vi "deleteMultichannel Lockin-Start Chopping.vi"() -> ()   [LabVIEW 2019, in "Instrument.Lockin.lvclass"]
uses:
  Instrument.Lockin/Instrument.Lockin.lvclass
  <vilib>/Utility/error.llb/DialogType.ctl
  Instrument UI.Lockin/Instrument UI.Lockin.lvclass
  <vilib>/measure/NI_MAPro.lvlib
  Instrument.DAQ/Instrument.DAQ.lvclass
  <vilib>/Utility/config.llb/NI_LVConfig.lvlib
  <vilib>/JKI/JKI SMO/SMO/SMO.lvclass
  <userlib>/LevyLab/Instrument Framework/SMOs/RemoteControl/RemoteControl.lvclass
  <userlib>/LevyLab/Instrument Framework/SMOs/RemoteControl/Typedefs/Message--Cluster.ctl
  <userlib>/LevyLab/Instrument Framework/SMOs/RemoteControl/Typedefs/PrivateEvents--RemoteControl.Configure.ctl
  Instrument.DAQ/Typedefs/Results--Cluster.ctl
  Instrument.DAQ/Typedefs/Set State-enum.ctl
  <vilib>/JKI/JKI SMO/SMO/Typedefs/Reserve State--Enum.ctl
  <vilib>/JKI/JKI SMO/SMO/Typedefs/Public Events.ctl
  <vilib>/JKI/JKI SMO/SMO/Typedefs/SMOState --Enum.ctl
  Instrument.DAQ/Typedefs/DAQ.Sampling.Sample Mode--Ring.ctl
  Instrument.DAQ/Typedefs/Sweep.Configuration--Cluster.ctl
  Instrument.DAQ/Typedefs/PublicEvents--DAQ.getSweepWaveforms.ctl
  Instrument.DAQ/Typedefs/PrivateEvents--DAQ.setCalibration.ctl
  Instrument.Lockin/Typedefs/Offset Mode--Enum.ctl
  Instrument.DAQ/Typedefs/Sweep.Pattern--Enum.ctl
  Instrument.DAQ/Typedefs/Sweep.Channel--Cluster.ctl
  Instrument.DAQ/Typedefs/DAQ.Sampling.Sampling--Cluster.ctl
  Instrument UI.Lockin/private/Set Legend (WFChart).vi
  Instrument UI.Lockin/private/Set Legend (WFGraph).vi
  Instrument UI.Lockin/private/Set Legend (WDTWFGraph).vi
  Instrument UI.Lockin/private/Set All Plot Visibility (WFGraph).vi
  Instrument UI.Lockin/private/Set All Plot Visibility (WFChart).vi
  <vilib>/Platform/browser.llb/Open URL in Default Browser (string).vi
  <userlib>/LevyLab/Instrument Framework/SMOs/Instrument/Instrument.lvclass
  Instrument UI.Lockin/private/Set Plot Visibility (WFGraph).vi
  Instrument UI.Lockin/private/Set Plot Visibility (WFChart).vi
  <userlib>/LevyLab/Instrument Framework/SMOs/Logger.Error/Logger.Error.lvclass
  f8e81ae1-39f2-419c-8ba3-60eeaa59b30a.vi
  Instrument UI.Lockin/private/Set All Plot Visibility (XYGraph).vi
  Instrument UI.Lockin/private/Set Plot Visibility (XYGraph).vi
  <userlib>/_OpenG.lib/error/error.llb/Filter Error Codes (Array)__ogtk.vi
  <vilib>/Waveform/WDTOps.llb/WDT Waveform Duration DBL.vi
  Instrument.DAQ/Typedefs/Sweep.Channel--Cluster--Array.ctl
  C:/Program Files (x86)/National Instruments/LabVIEW 2019/vi.lib/JKI/JKI SMO/SMO/SMO.lvclass
  C:/Program Files (x86)/National Instruments/LabVIEW 2019/user.lib/LevyLab/Instrument Framework/SMOs/Instrument/Instrument.lvclass
  <vilib>/measure/maspectr.llb/FFT Power Spectrum and PSD for N Chan.vi
  Instrument.DAQ/Typedefs/DAQ.Config.AI.Coupling--enum.ctl
  Instrument.DAQ/Typedefs/DAQ.Config.AI.Range--enum.ctl
  Instrument.DAQ/Typedefs/DAQ.Config.AO.Range--enum.ctl
  Instrument.DAQ/Typedefs/AO.Channel.Function--Enum.ctl
  Instrument.DAQ/Typedefs/DAQ.Calibration--Cluster.ctl
  Instrument.DAQ/Typedefs/DAQ.Type--enum.ctl
  Instrument UI.Lockin/Typedefs/Display-Enum.ctl
  Instrument.DAQ/Typedefs/Simulation Mode--enum.ctl
  Instrument.Lockin/Typedefs/DELETE_Lockin.Auto Sample Mode--Enum.ctl
  Instrument.DAQ/Typedefs/DAQ.Configuration--Cluster.ctl
  Instrument.DAQ/Typedefs/REF.Channel--Cluster.ctl
  Instrument.Lockin/Typedefs/Results Type--Enum.ctl
panel:
  out "Results Plot Names":string[](array[string])
  in  "Tab Control 4":T1(tab)
  in  "Disable all AI Ref":bool
  in  "Enable only AI Ref1":bool
  in  "Reset Phase":bool
  in  "AI Channels":T2(array[cluster]) {"References" items=["", "1"]}
  in  "AO freq link":dbl=13.0 format="%.3p"
  in  "AO Amp Limit":dbl=0.009999999 format="%.3p"
  in  "Limit Amplitudes":bool
  in  "Link Frequencies":bool
  in  "LP f (Hz)":dbl=100.0 format="%.3p"
  in  "Line":bool
  in  "Lowpass":bool
  in  "AO Channels":T4(array[cluster]) {"Phase" format="%.3g"; "Frequency" min=0.0001 max=10000.0 format="%.3g"; "Offset" format="%.3p"; "Amplitude" min=0.0 max=10.0 format="%.3p"}
  in  "REF Channels":T5[](array[typedef]) {"Roll-Off" min=1; "TC" min=0.0001 format="%#_3p"; "Phase" format="%.3g"; "Frequency" min=0.0001 max=10000.0 format="%.3g"; "Channel" min=1}
  in  "DAQ Config":T6[](array[typedef]) {"AI.Coupling" items=["AC"=10045, "DC"=10050, "GND"=10066]}
  in  "auto DAQ":bool
  in  "Max Fs Refresh Rate (Hz)":dbl=10.0 format="%#_13g"
  in  "Sampling Mode":T10
  in  "Sampling":T11={"Fs"=10000.0, "#s"=1000}
  in  "DAQ Type":T12=enum."PXI 446x"
  in  "Auto x*F1":dbl=5000.0 format="%#_13g"
  in  "Load Configuration":bool
  in  "Save Configuration":bool
  in  "AI Simulation mode":T13=enum."AI = noise*AO"
  in  "decimating factor":i32=1
  in  "Remove":bool
  in  "Measure":bool
  in  "Channels: Sweep":T15(array[cluster]) {"Channel" items=["AO1"=1, "AO2"=2, "AO3"=3, "AO4"=4, "AO5"=5, "AO6"=6, "AO7"=7, "AO8"=8]; "Start" format="%#_6p"; "End" format="%#_6p"}
  in  "Stop Sweep":bool caption="Stop"
  in  "Sweep Time (s)":dbl=20.0 format="%#_1f"
  in  "Start Sweep":bool caption="Start"
  in  "Initial Wait (s)":dbl=1.0
  out "Sweep Timer (s)":dbl caption="Timer (s)"
  in  "Return to Start?":bool
  out "Sampling Status":string="Good"
  in  "Output Gain":cluster{"AI.Ch":string, "Gain":dbl}[](array[cluster])=[{"AI.Ch"="AO1", "Gain"=1.0}, {"AI.Ch"="AO2", "Gain"=1.0}, {"AI.Ch"="AO3", "Gain"=1.0}, {"AI.Ch"="AO4", "Gain"=1.0}, {"AI.Ch"="AO5", "Gain"=1.0}, {"AI.Ch"="AO6", "Gain"=1.0}, {"AI.Ch"="AO7", "Gain"=1.0}, {"AI.Ch"="AO8", "Gain"=1.0}, {"AI.Ch"="AO9", "Gain"=1.0}, {"AI.Ch"="AO10", "Gain"=1.0}, {"AI.Ch"="AO11", "Gain"=1.0}, {"AI.Ch"="AO12", "Gain"=1.0}, {"AI.Ch"="AO13", "Gain"=1.0}, {"AI.Ch"="AO14", "Gain"=1.0}, {"AI.Ch"="AO15", "Gain"=1.0}, {"AI.Ch"="AO16", "Gain"=1.0}]
  in  "Input Gain":cluster{"AI.Ch":string, "Gain":dbl}[](array[cluster])=[{"AI.Ch"="AI1", "Gain"=1.0}, {"AI.Ch"="AI2", "Gain"=1.0}, {"AI.Ch"="AI3", "Gain"=1.0}, {"AI.Ch"="AI4", "Gain"=1.0}, {"AI.Ch"="AI5", "Gain"=1.0}, {"AI.Ch"="AI6", "Gain"=1.0}, {"AI.Ch"="AI7", "Gain"=1.0}, {"AI.Ch"="AI8", "Gain"=1.0}, {"AI.Ch"="AI9", "Gain"=1.0}, {"AI.Ch"="AI10", "Gain"=1.0}, {"AI.Ch"="AI11", "Gain"=1.0}, {"AI.Ch"="AI12", "Gain"=1.0}, {"AI.Ch"="AI13", "Gain"=1.0}, {"AI.Ch"="AI14", "Gain"=1.0}, {"AI.Ch"="AI15", "Gain"=1.0}, {"AI.Ch"="AI16", "Gain"=1.0}]
  out "State History":string=" Exit\r Data: Cleanup\r Events: Unregister\r UI: Cleanup\r UI: Disable Buttons\r Configuration: Write\r Error Logger: Destroy\r Lockin SMO: Stop\r Remote SMO: Stop\r Macro: Exit\r UI: Update Sweep Timer\r UI: Update Lockin Graphs\r UI: Update Waveform Graphs\r 4461: OUT\r UI: Update Sweep Timer\r UI: Update Lockin Graphs\r UI: Update Waveform Graphs\r 4461: OUT\r UI: Update Sweep Timer\r UI: Update Lockin Graphs\r UI: Update Waveform Graphs\r 4461: OUT"
  out "Refresh time (ms)":u32=103
  out "LockinDAQ SMO State":T16=enum."Stopped" caption="SMO State"
  out "RC SMO State":T16=enum."Stopped" caption="SMO State"
  in  "Update":bool
  in  "Enable Output":bool caption="Enable"
  in  "Output Channel":i32=1 min=1
  out "Output (V)":dbl
  in  "Aux Channel":tag="Dev2/ao0"
  in  "Voltage Output (V)":dbl min=-50.0 max=50.0
  in  "Amplifier Gain":dbl=1.0 min=-15.0 max=15.0
  out "DAQ Output (V)":dbl=-0.0 min=-3.5 max=3.5
  out "Amplified Output (V)":dbl=-0.0 min=-3.5 max=3.5
  in  "AI Channel":i32=1
  in  "Reference Channel":i32=1
  in  "Type":T17
  in  "Allowed remote system":string
  in  "Get Calibration":bool
  out "Cal Info":T18[](array[typedef]) {"SelfCal.LastDate/Time" format="%<%I:%M %p\n%m/%d/%Y>T"}
  in  "Self Calibrate":bool
  in  "Tab Control 3":enum32{"Page 1"}(tab)
  out "X":dbl=0.0014996100939563214 caption="X (V)" format="%#_3p"
  out "Y":dbl=-29.79492153733761 caption="Y (V)" format="%#_3p"
  in  "Channel":i32(ring)=1
  out "R":dbl=0.0014996100939563214 caption="R (V)" format="%#_3p"
  out "Theta":dbl=-29.79492153733761 caption="Theta (°)" format="%#_3p"
  in  "Display":T19=enum."R and Theta" caption="Enum"
  in  "Close":bool
  out "Status":string="Shutdown"
  in  "Pause":bool
  in  "Reset":bool
  in  "Start":bool
  in  "Help":bool
  in  "Trigger":bool
  in  "Tab Control 2":T20(tab)
  in  "AI Graph All":bool
  in  "AI Graph None":bool
  in  "Y Axis (Output)":enum16{"Analog Output", "Reference"}(ring) caption="Enum 3"
  in  "Y Axis (Input)":enum16{"Device", "ADC"}(ring) caption="Enum 3"
  in  "Decimate":enum16{"1", "10", "100", "1000"}(ring) caption="Enum 3"
  in  "X Axis":enum16{"Time", "Samples"}(ring) caption="Enum 3"
  out "AI Graph":waveform(dbl)[](graph)
  out "AO Graph":waveform(dbl)[](graph)
  in  "AO Graph All":bool
  in  "AO Graph None":bool
  in  "Y/Theta Range":dbl caption="Axis Range" format="%#_6p"
  in  "X/R Range":dbl caption="Axis Range" format="%#_6p"
  out "Lockin 2":waveform(dbl)[](graph) caption="Lockin Display 2"
  out "Lockin 1":waveform(dbl)[](graph)
  in  "Lockin 1 None":bool
  in  "Lockin 1 All":bool
  out "Results":string[][](table)
  out "XY Graph":cluster{"Wavenumber":dbl[], "Data":dbl[]}[](graph)
  in  "Numeric":dbl caption="Axis Range" format="%#_6p"
  out "Sweep Results Y":waveform(dbl)[](graph)
  out "Sweep Results X":waveform(dbl)[](graph)
  out "Sweep Results AI":waveform(dbl)[](graph)
  out "Sweep Results AO":waveform(dbl)[](graph)
  in  "# averages":u32=10 min=1
  in  "weighting mode":enum16{"Linear", "Exponential"}(ring)=enum."Exponential"
  in  "averaging mode":T21(ring)=enum."RMS averaging"
  in  "window":u16(ring) items=["Rectangle", "Hanning"]
  in  "export mode":u16(ring)=1 items=["Power Spectrum", "Power Spectral Density"]
  in  "restart":bool
  out "done?":bool=TRUE
  out "PS Chart":dbl[][](graph)
  out "PS WFGraph":cluster{"f0":dbl, "df":dbl, "magnitude":dbl[]}[](graph)
  out "averages":dbl=180.0
  # "Output"
  # "Input"
  # ">> DEVICE >>"
  # "Amp (V)"
  # "(*)"
  # "Ch"
  # "DC (V)"
  # "f (Hz)"
  # "Phase (°)"
  # "Function"
  # "Sweep"
  # "(*)"
  # "Ch"
  # "Ref1   2     3    4"
  # "Input: Pre-Filter"
  # "Output Settings"
  # "Reference"
  # "Reference Settings"
  # "Ch"
  # "f (Hz)"
  # "Phase (°)"
  # "TC (s)"
  # "Order"
  # "DAQ Channels"
  # "AI"
  # "Device"
  # "AO"
  # "Input: Offset"
  # "Ch"
  # "Range"
  # "Ch"
  # "Range"
  # "Coupling"
  # "Other Configuration"
  # "Sampling"
  # "Changing settings in this box will automatically\nreset the lockin and restart acquisition"
  # "Sweep"
  # "Channel"
  # "Start"
  # "End"
  # "Pattern"
  # "Status"
  # "Channel"
  # "Channel"
  # "Input Gain"
  # "Output Gain"
  # "Auxiliary Output"
  # "Configuration"
  # "- Use to control an auxiliiary card such as a multifunction DAQ (6115, 6120, etc)"
  # "Forward Lockin Input --> Lockin Output"
  # "- Choose an input lockin channel and value (X,Y, etc) and it will be written as a DC value to an output channel of your choosing.\n- Output is scaled by the input amplifier gain."
  # "Calibration"
  # "Self Cal\nLast Time"
  # "Self Cal\nLast Temp"
  # "Temp\nNow"
  # "Cal\nDue"
  # "Device"
  # "AI Graph"
  # "AO/Reference Graph"
  # "Lockin Results 1"
  # "Lockin Results 2"
  # "Lockin Results 2"
  # "Sweep Results"
  # "Sweep AO/AI"
  # "Power Spectra"
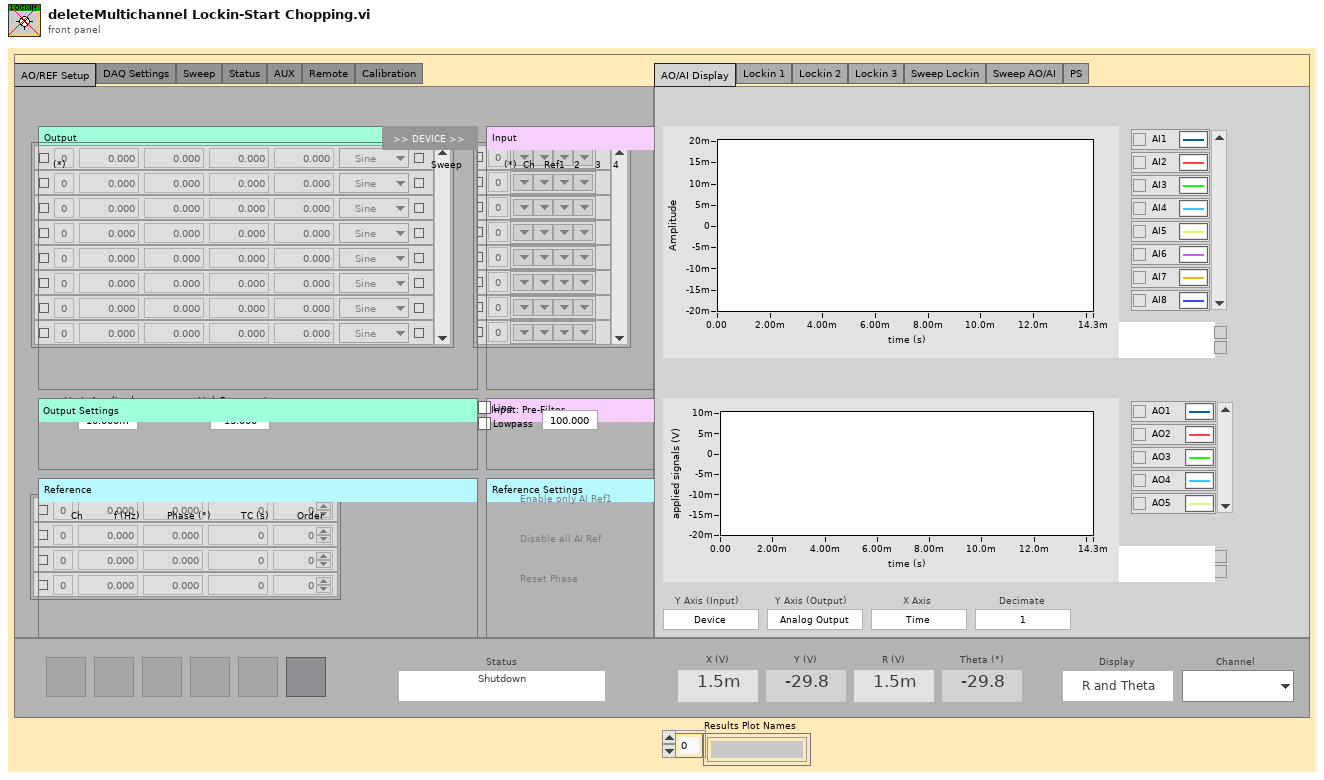
[diagram p1: front panel]
types:
  T1 = enum32{"AO/REF Setup", "DAQ Settings", "Sweep", "Status", "AUX", "Remote", "Calibration"}
  T2 = cluster{"Enable?":bool, "Channel":i32, "References":u16[]}[]
  T3 = typedef "Instrument.DAQ.lvclass/AO.Channel.Function--Enum.ctl" = enum16{"Sine", "Triangle", "Square"}
  T4 = cluster{"Enable?":bool, "Channel":i32, "Amplitude":dbl, "Offset":dbl, "Frequency":dbl, "Phase":dbl, "Function":T3, "Sweeping?":bool}[]
  T5 = typedef "Instrument.DAQ.lvclass/REF.Channel--Cluster.ctl" = cluster{"Enable?":bool, "Channel":i32, "Frequency":dbl, "Phase":dbl, "TC":dbl, "Roll-Off":i32}
  T6 = typedef "Instrument.DAQ.lvclass/DAQ.Configuration--Cluster.ctl" = cluster{"Device":string, "AO.Ch":string, "AO.Range":T7, "AI.Ch":string, "AI.Range":T8, "AI.Coupling":T9}
  T7 = typedef "Instrument.DAQ.lvclass/DAQ.Config.AO.Range--enum.ctl" = enum16{"±0.1", "±1.0", "±10.0"}
  T8 = typedef "Instrument.DAQ.lvclass/DAQ.Config.AI.Range--enum.ctl" = enum16{"±0.316", "±1.00", "±3.16", "±10.0", "±31.6", "±42.4"}
  T9 = typedef "Instrument.DAQ.lvclass/DAQ.Config.AI.Coupling--enum.ctl" = u16
  T10 = typedef "DELETE_Lockin.Auto Sample Mode--Enum.ctl" = enum16{"Manual", "Auto Fs", "Max Fs"}
  T11 = typedef "Instrument.DAQ.lvclass/DAQ.Sampling.Sampling--Cluster.ctl" = cluster{"Fs":dbl, "#s":i32}
  T12 = typedef "Instrument.DAQ.lvclass/DAQ.Type--enum.ctl" = enum16{"None", "USB 4431", "PXI 446x"}
  T13 = typedef "Instrument.DAQ.lvclass/Simulation Mode--enum.ctl" = enum16{"AI = HW simulated", "AI = noise*AO", "AI = waveguide"}
  T14 = typedef "Instrument.DAQ.lvclass/Sweep.Pattern--Enum.ctl" = enum16{"Ramp /", "Ramp /\\", "Smooth Ramp _/", "Smooth Ramp _/\\_", "Frequency"}
  T15 = cluster{"Enable?":bool, "Channel":u16, "Start":dbl, "End":dbl, "Pattern":T14}[]
  T16 = typedef "SMO.lvclass/SMOState --Enum.ctl" = enum16{"unknown", "Created", "Started", "Stopped"}
  T17 = typedef "Instrument.Lockin.lvclass/Results Type--Enum.ctl" = enum16{"X", "Y", "R", "Theta", "Mean"}
  T18 = typedef "Instrument.DAQ.lvclass/DAQ.Calibration--Cluster.ctl" = cluster{"Active Device":string, "SelfCal.LastDate/Time":dbl, "SelfCal.LastTemp":dbl, "DevTemp":dbl, "calibration due?":bool}
  T19 = typedef "Instrument UI.Lockin.lvclass/Display-Enum.ctl" = enum16{"X and Y", "R and Theta", "Mean"}
  T20 = enum32{"AO/AI Display", "Lockin 1", "Lockin 2", "Lockin 3", "Sweep Lockin", "Sweep AO/AI", "PS"}
  T21 = enum16{"No averaging", "Vector averaging", "RMS averaging", "Peak hold"}
  T22 = typedef "Instrument.DAQ.lvclass/Set State-enum.ctl" = enum16{"start", "stop", "reset", "start sweep", "stop sweep"}
  T23 = typedef "Instrument.DAQ.lvclass/Sweep.Configuration--Cluster.ctl" = cluster{"Sweep Time (s)":dbl, "Initial Wait (s)":dbl, "Return to Start":bool, "Channels":T24}
  T24 = typedef "Instrument.DAQ.lvclass/Sweep.Channel--Cluster--Array.ctl" = T25[]
  T25 = typedef "Instrument.DAQ.lvclass/Sweep.Channel--Cluster.ctl" = cluster{"Enable?":bool, "Channel":u16, "Start":dbl, "End":dbl, "Pattern":T14}
  T26 = enum32{"invalid app kind", "Development System", "Run Time System", "Student Edition", "Embedded LabVIEW", "Evaluation", "Custom"}
  T27 = enum8{"Enabled", "Disabled", "Disabled and Grayed Out"}
  T28 = enum32{"Invalid", "Standard", "Closed", "Hidden", "Minimized", "Maximized"}
  T29 = typedef "Instrument.DAQ.lvclass/PrivateEvents--DAQ.setCalibration.ctl" = enum16{"Check", "Calibrate"}
  T30 = cluster{"averaging mode":enum16{"No averaging", "Vector averaging", "RMS averaging", "Peak hold"}, "weighting mode":enum16{"Linear", "Exponential"}, "number of averages":u32}
  T31 = typedef "Instrument.Lockin.lvclass/Offset Mode--Enum.ctl" = enum16{"Measure", "Remove"}
  T32 = typedef "Instrument.DAQ.lvclass/Get State-enum.ctl" = enum16{"idle", "created", "started", "stopped", "sweeping"}
  T33 = typedef "RemoteControl.lvclass/PrivateEvents--RemoteControl.Configure.ctl" = cluster{"address":string, "Port":u16, "AllowedRemote":string, "Commands":string[], "timeout":i32}
  T34 = typedef "RemoteControl.lvclass/Message--Cluster.ctl" = cluster{"Command":string, "Data":variant, "ID":string}
  T35 = typedef "Instrument.DAQ.lvclass/PublicEvents--DAQ.getSweepWaveforms.ctl" = cluster{"Sweep AO":waveform(dbl)[], "Sweep AI":waveform(dbl)[], "Sweep Results X":waveform(dbl)[], "Sweep Results Y":waveform(dbl)[]}
  T36 = cluster{"Core":cluster{"Current VI Reference":refnum<vi>, "Close Panel on Exit?":bool}, "to":i32, "Lockin":refnum<class "Instrument.Lockin.lvclass">, "RemoteControl":refnum<class "RemoteControl.lvclass">, "Lockin.DAQ":refnum<class "Instrument.DAQ.lvclass">, "Logger.Error":refnum<class "Logger.Error.lvclass">, "RemoteControl.Configure":T33, "Message":T34, "HandledMessage":T34, "SweepWaveforms":T35}
  T37 = typedef "Instrument.DAQ.lvclass/State-enum.ctl" = enum16{"idle", "created", "started", "stopped", "sweeping"}
  T38 = typedef "Instrument.DAQ.lvclass/REF.Channel--Cluster--Array.ctl" = T5[]
  T39 = typedef "Instrument.DAQ.lvclass/DAQ Configuration--Cluster--Array.ctl" = T40[]
  T40 = typedef "Instrument.DAQ.lvclass/DAQ Configuration--Cluster.ctl" = cluster{"Device":string, "AO.Ch":string, "AO.Range":T41, "AI.Ch":string, "AI.Range":T42, "AI.Coupling":T43}
  T41 = typedef "Instrument.DAQ.lvclass/446xAO-enum.ctl" = enum16{"±0.1", "±1.0", "±10.0"}
  T42 = typedef "Instrument.DAQ.lvclass/446xAI-enum.ctl" = enum16{"±0.316", "±1.00", "±3.16", "±10.0", "±31.6", "±42.4"}
  T43 = typedef "Instrument.DAQ.lvclass/AI.coupling-enum.ctl" = u16
  T44 = typedef "Instrument.DAQ.lvclass/DAQ.Config.AO--Cluster--Array.ctl" = T45[]
  T45 = typedef "Instrument.DAQ.lvclass/DAQ.Config.AO--Cluster.ctl" = cluster{"Channels":tag, "Range":T7, "output terminal configuration":i32, "Type":T12}
  T46 = typedef "Instrument.DAQ.lvclass/DAQ.Config.AI--Cluster--Array.ctl" = T47[]
  T47 = typedef "Instrument.DAQ.lvclass/DAQ.Config.AI--Cluster.ctl" = cluster{"Channels":tag, "Coupling":T9, "Range":T8, "input terminal configuration":i32, "Type":T12}
  T48 = typedef "Instrument.DAQ.lvclass/Channel.Gain--Cluster--Array.ctl" = T49[]
  T49 = typedef "Instrument.DAQ.lvclass/Channel.Gain--Cluster.ctl" = cluster{"Channel":string, "Gain":dbl}
  T50 = typedef "Instrument.DAQ.lvclass/DAQ.Sampling.Sample Mode--Ring.ctl" = i32
  T51 = typedef "DialogType.ctl" = u16
  T52 = typedef "Instrument.DAQ.lvclass/Results--Cluster.ctl" = cluster{"Time Stamp":timestamp, "Results (Dictionary)":cluster{"key":string, "value":dbl}[]}
  T53 = cluster{"Current VI Reference":refnum<vi>, "Close Panel on Exit?":bool}
  T54 = typedef "SMO.lvclass/Public Events.ctl" = cluster{"Error":refnum<user-event>, "State":refnum<user-event>, "Reserve State":refnum<user-event>}
  T55 = typedef "RemoteControl.lvclass/PublicEvents--Cluster.ctl" = cluster{"SendMessageFromProcess":refnum<user-event>}
  T56 = typedef "Instrument.DAQ.lvclass/PublicEvents--Cluster.ctl" = cluster{"getAIChannels":refnum<user-event>, "getAOChannels":refnum<user-event>, "getREFChannels":refnum<user-event>, "getWaveforms":refnum<user-event>, "getResults":refnum<user-event>, "getSweepWaveforms":refnum<user-event>, "getCalibration":refnum<user-event>, "getDAQState":refnum<user-event>, "getDAQconfig":refnum<user-event>, "getInputGain":refnum<user-event>, "getOutputGain":refnum<user-event>, "getInputOffset":refnum<user-event>}
  T57 = typedef "Instrument.DAQ.lvclass/AI.Channel--Cluster--Array.ctl" = T58[]
  T58 = typedef "Instrument.DAQ.lvclass/AI.Channel--Cluster.ctl" = cluster{"Enable?":bool, "Channel":i32, "References":i32[]}
  T59 = typedef "Instrument.DAQ.lvclass/DAQ.Sampling--Cluster.ctl" = cluster{"Sampling":T11, "Sample Mode":T50, "Fs Mode":T60, "Fs Multiplier":dbl, "Refresh Rate (Hz)":dbl, "Decimation":i32}
  T60 = typedef "Instrument.DAQ.lvclass/DAQ.Sampling.Fs Mode--enum.ctl" = enum16{"Manual", "Auto Fs", "Max Fs"}
  T61 = typedef "Instrument.DAQ.lvclass/AO.Channel--Cluster--Array.ctl" = T62[]
  T62 = typedef "Instrument.DAQ.lvclass/AO.Channel--Cluster.ctl" = cluster{"Enable?":bool, "Channel":i32, "Amplitude":dbl, "Offset":dbl, "Frequency":dbl, "Phase":dbl, "Function":T3, "Sweeping?":bool}
  T63 = typedef "Instrument.DAQ.lvclass/Configuration.Prefilter--Cluster.ctl" = cluster{"60 Hz":bool, "Low Pass":bool, "Low Pass Cutoff (Hz)":dbl}
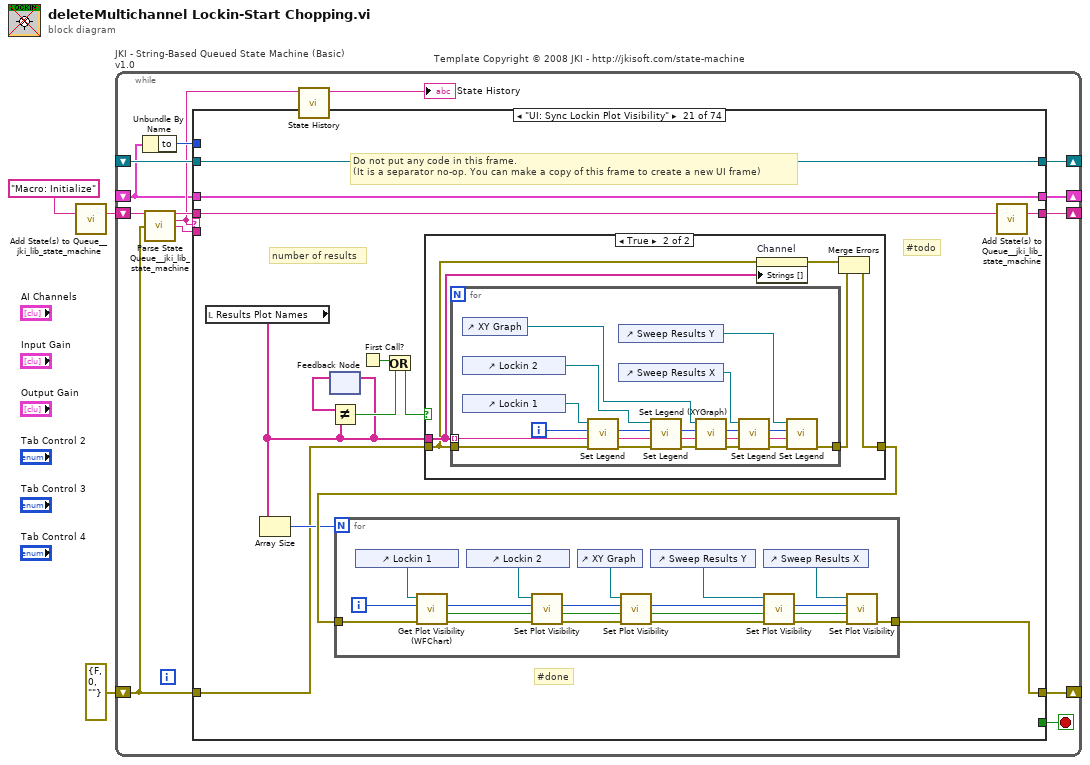
[diagram p0: block diagram]
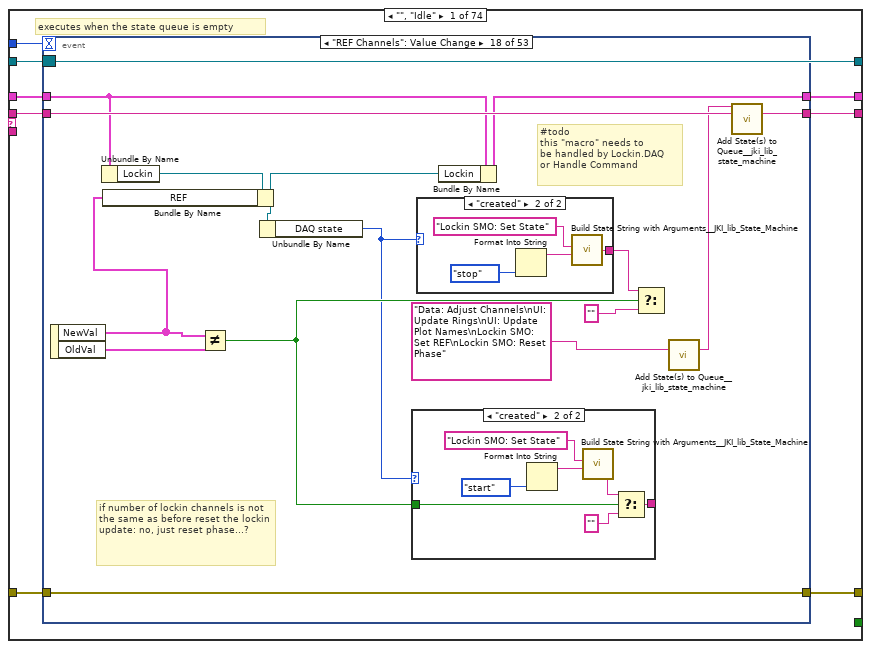
[diagram p2: hidden frame]
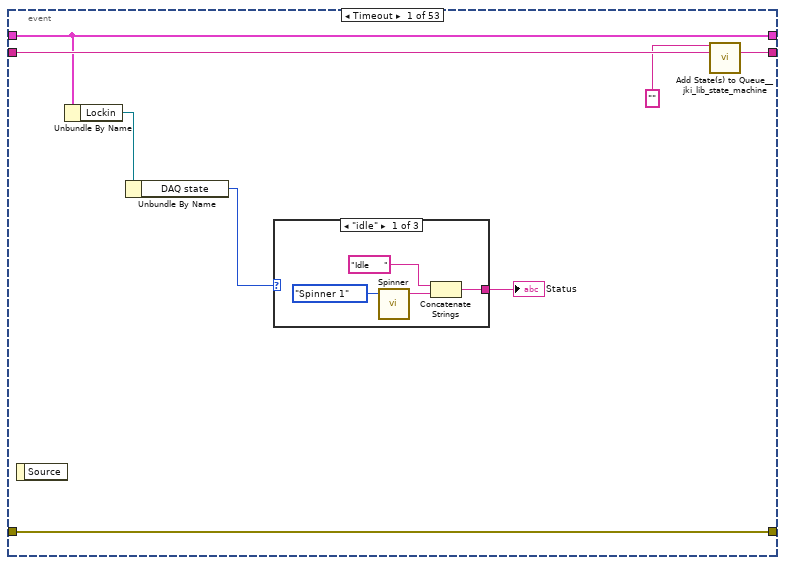
[diagram p3: hidden frame]
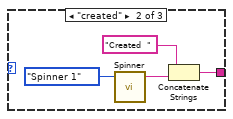
[diagram p4: hidden frame]
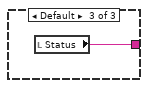
[diagram p5: hidden frame]
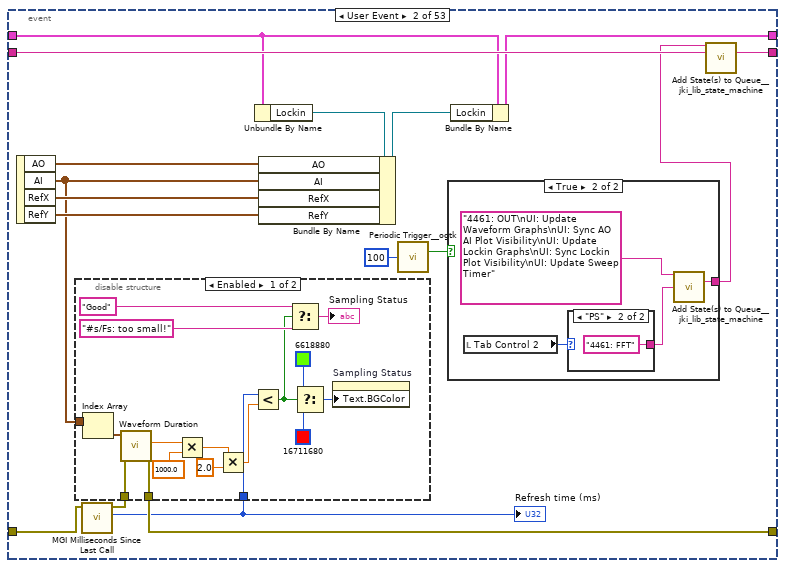
[diagram p6: hidden frame]
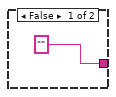
[diagram p7: hidden frame]
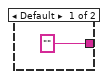
[diagram p8: hidden frame]
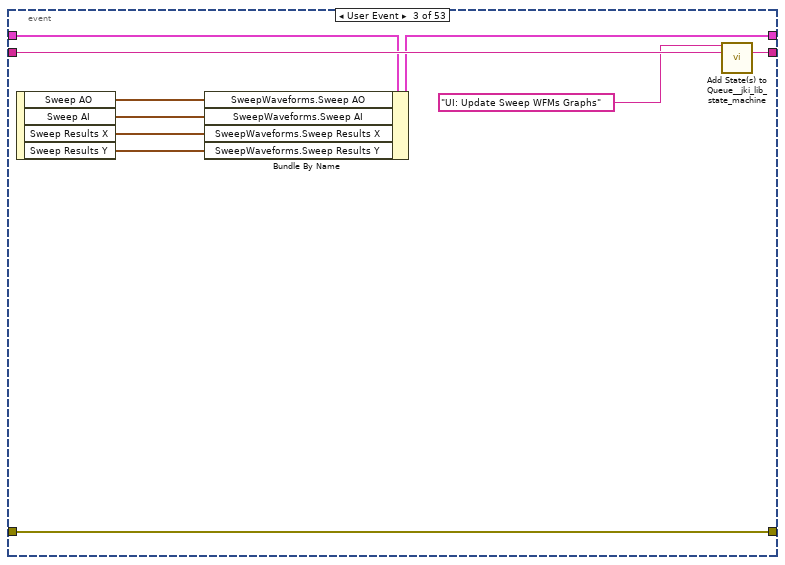
[diagram p10: hidden frame]
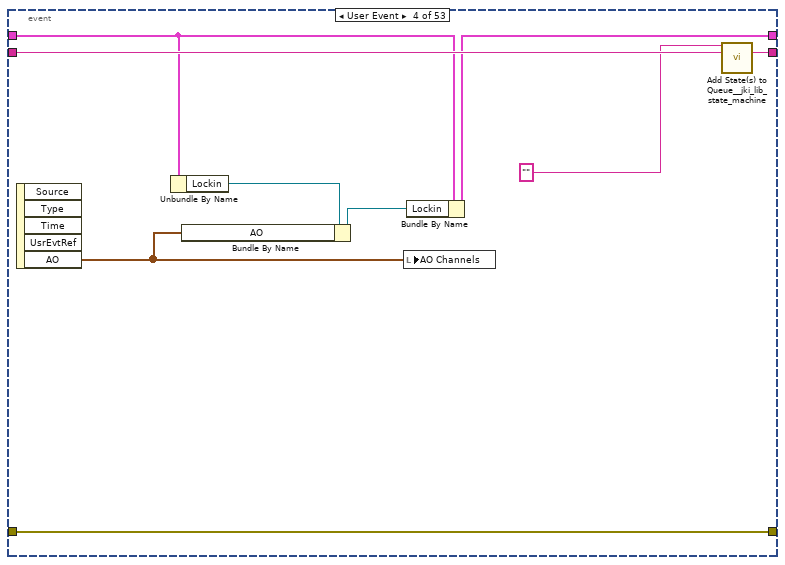
[diagram p11: hidden frame]
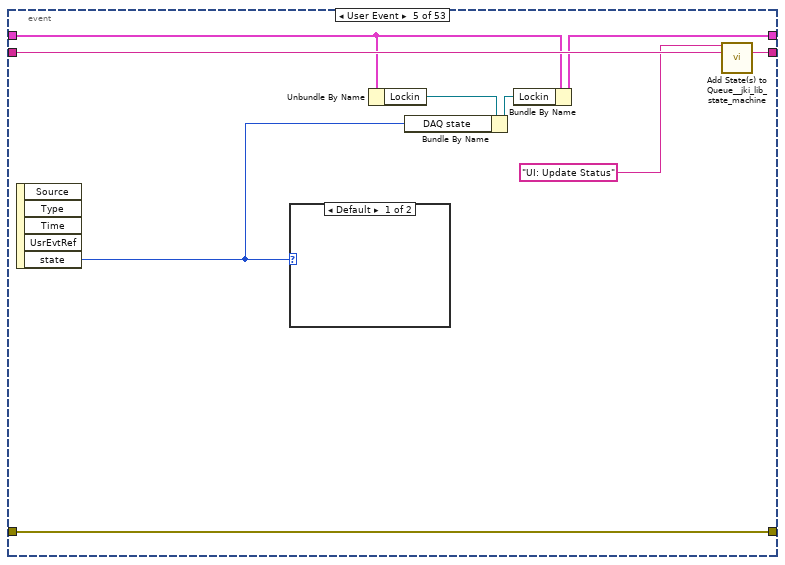
[diagram p12: hidden frame]
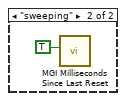
[diagram p13: hidden frame]
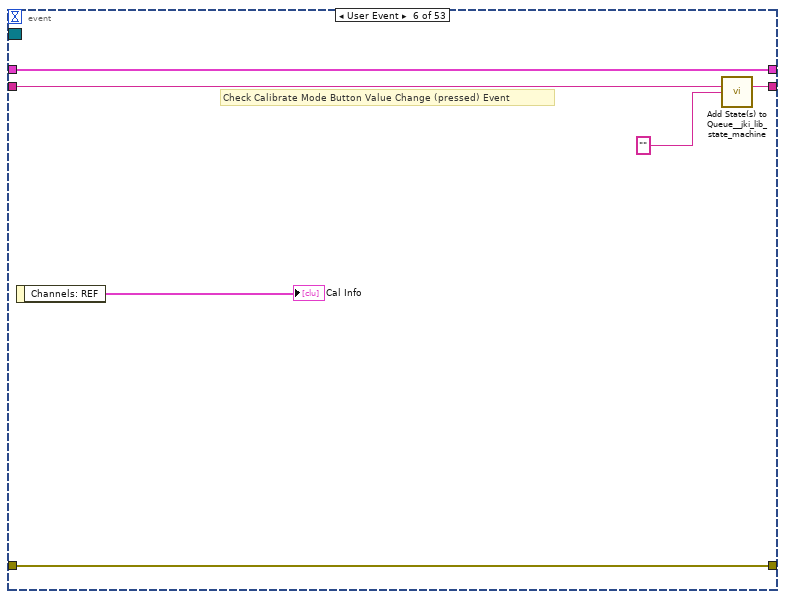
[diagram p14: hidden frame]
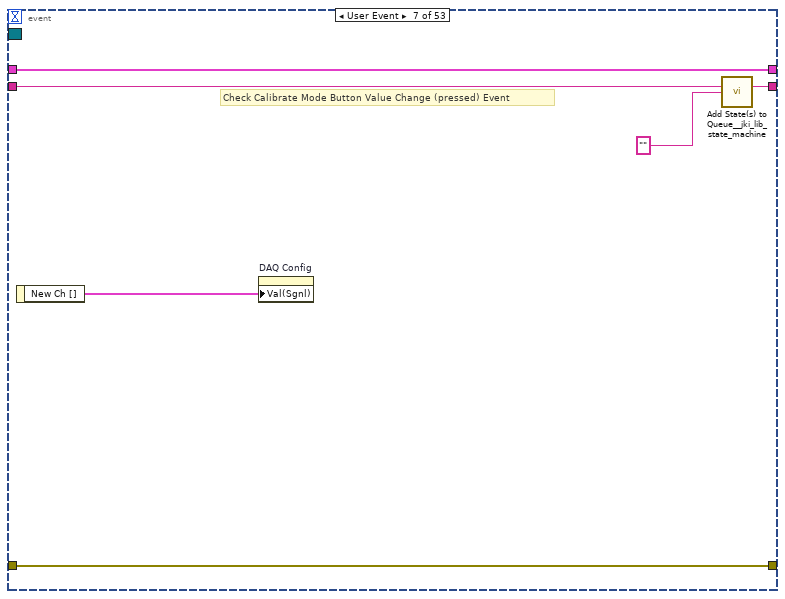
[diagram p15: hidden frame]
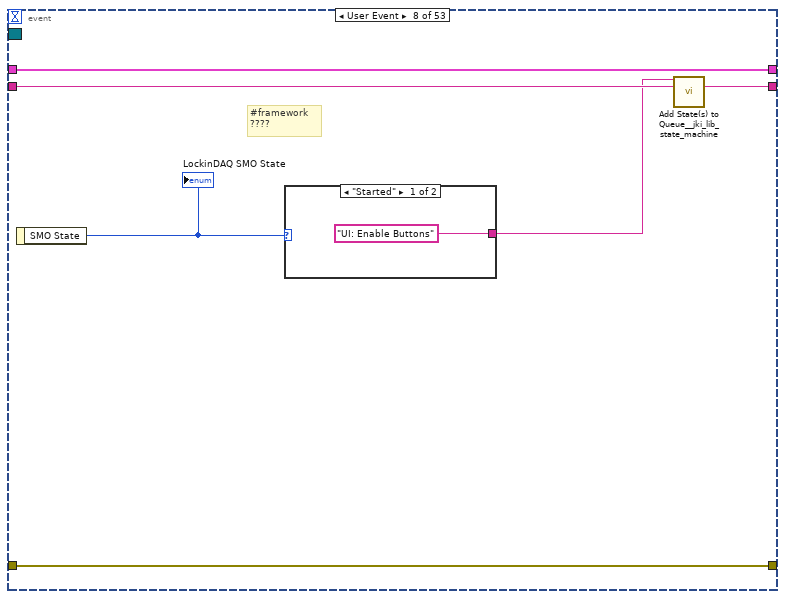
[diagram p16: hidden frame]
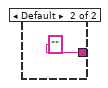
[diagram p17: hidden frame]
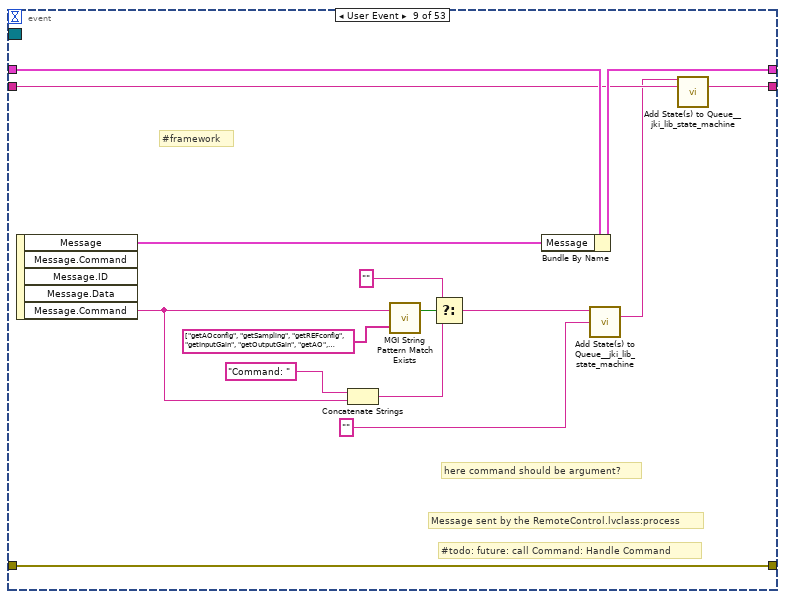
[diagram p18: hidden frame]
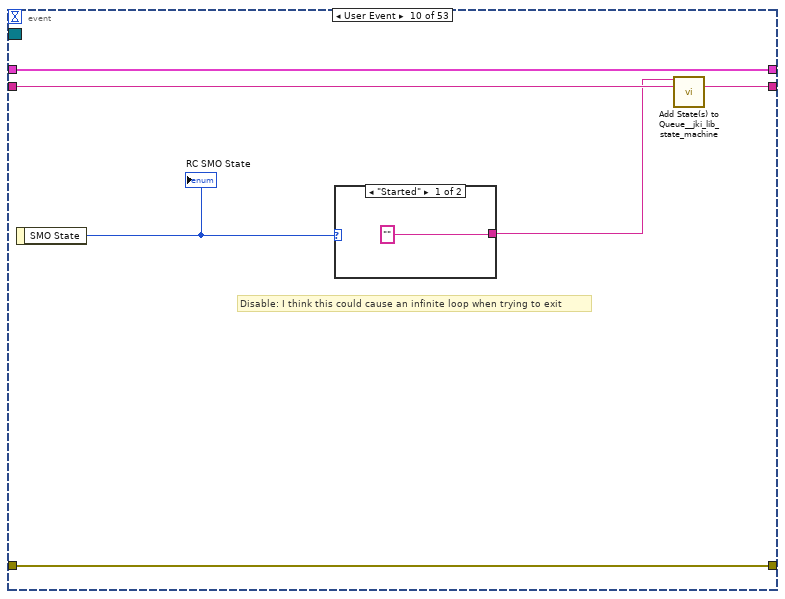
[diagram p19: hidden frame]
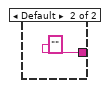
[diagram p20: hidden frame]
diagram:
  # "Template Copyright © 2008 JKI - http://jkisoft.com/state-machine"
  n1 = call <vilib>:"Add State(s) to Queue__jki_lib_state_machine.vi"("State(s) in (\"\")"="Macro: Initialize") -> ("States Out"=w3:string)  [unwired: 14 in]
  n2 = while "JKI - String-Based Queued State Machine (Basic) v1.0" {
    shift-right: [w9] -> _
    shift-left: _ -> [w4]
    shift-right: [w6] -> _
    shift-left: errorcluster {"status"=FALSE, "code"=0, "source"=""} ("error out") -> [w5]
    shift-right: [w16] -> _
    shift-left: w3 -> [w13]
    shift-right: [w10] -> _
    shift-left: _ -> [w11]
    stop <- w15 stop-if-true
    n3 = Unbundle By Name(w4) -> ("to"=w12:i32)
    n4 = call <vilib>:"Parse State Queue__jki_lib_state_machine.vi"("State Queue"=w13, "Error In (no error)"=w5) -> ("Remaining States"=w14:string, "Current State"=w7:string, "Arguments"=w17:string)  [unwired: 11 in]
    n5 = case shown="\"UI: Sync Lockin Plot Visibility\"" w7 {
      selector: w7 -> [_ _ w586 _ _ _ _ _ _ _ _ _ _ _ _ _ _ _ _ _ _ _ _ _ _ _ _ _ _ _ _ _ _ _ _ _ _ _ _ _ _ _ _ _ _ _ _ _ _ _ _ _ _ _ _ _ _ _ _ _ _ _ _ _ _ _ _ _ _ _ _ _ _ _]
      tunnel: w17 -> [_ _ _ _ _ _ _ _ _ _ _ _ _ _ _ _ w750 _ _ _ _ _ _ _ w970 w984 w1003 _ _ _ _ _ _ _ _ _ w1162 w1175 w1185 _ _ _ _ _ _ _ _ w1314 _ _ w1354 _ _ _ _ _ _ _ w1439 _ _ _ _ _ _ _ _ _ _ _ _ _ _ _]
      tunnel: [w24 w582 w589 w607 w620 w632 w637 w652 w673 w680 w685 w710 w715 w726 w737 w748 w761 w781 w799 w820 w862 w919 w948 w961 w974 w987 w1006 w1037 w1067 w1080 w1091 w1099 w1115 w1122 w1130 w1150 w1167 w1176 w1188 w1220 w1225 w1232 w1237 w1245 w1283 w1305 w1310 w1320 w1340 w1349 w1361 w1372 w1389 w1401 w1410 w1419 w1428 w1437 w1446 w1455 w1462 w1469 w1476 w1481 w1495 w1523 w1563 w1572 w1586 w1591 w1607 w1614 w1619 w1624] -> w16
      tunnel: [_ _ _ _ _ TRUE _ _ _ _ _ _ _ _ _ _ _ _ _ _ _ _ _ _ _ _ _ _ _ _ _ _ _ _ _ _ _ _ _ _ _ _ _ _ _ _ _ _ _ _ _ _ _ _ _ _ _ _ _ _ _ _ _ _ _ _ _ _ _ _ _ _ _ _] -> w15
      tunnel: w12 -> [w19 _ _ _ _ _ _ _ _ _ _ _ _ _ _ _ _ _ _ _ _ _ _ _ _ _ _ _ _ _ _ _ _ _ _ _ _ _ _ _ _ _ _ _ _ _ _ _ _ _ _ _ _ _ _ _ _ _ _ _ _ _ _ _ _ _ _ _ _ _ _ _ _ _]
      tunnel: w14 -> [w25 w583 w590 w608 w621 w633 w638 w653 w674 w681 w686 w711 w716 w727 w738 w749 w762 w782 w800 w821 w863 w920 w949 w962 w975 w988 w1007 w1038 w1068 w1081 w1092 w1100 w1116 w1123 w1131 w1151 w1168 w1177 w1189 w1221 w1226 w1227 w1238 w1246 w1284 w1306 w1311 w1321 w1341 w1350 w1362 w1373 w1390 w1402 w1411 w1420 w1429 w1438 w1447 w1456 w1463 w1470 w1477 w1482 w1496 w1522 w1559 w1573 w1587 w1592 w1608 w1615 w1620 w1625]
      tunnel: w11 -> [w18 w580 w585 w596 w616 w629 w635 w650 w672 w679 w683 _ w712 w725 w736 w747 w760 w780 w798 w819 w860 w918 w945 w958 w972 w985 w1004 w1036 w1066 w1078 w1088 w1096 w1113 w1120 w1128 w1147 w1165 w1173 w1182 w1218 w1222 w1230 w1234 w1244 w1281 w1298 w1307 w1319 w1339 w1348 w1360 w1371 w1388 w1400 w1409 w1418 w1427 w1436 w1445 w1454 w1461 w1468 w1475 w1478 w1494 w1521 w1560 w1569 w1585 w1588 w1606 w1611 w1616 w1621]
      tunnel: [w18 w580 w585 w596 w616 w629 w635 w650 w672 w679 w683 w709 w712 w725 w736 w747 w760 w780 w798 w819 w860 w918 w945 w958 w972 w985 w1004 w1036 w1066 w1078 w1088 w1096 w1113 w1120 w1128 w1147 w1165 w1173 w1182 w1218 w1222 w1230 w1234 w1244 w1281 w1298 w1307 w1319 w1339 w1348 w1360 w1371 w1388 w1400 w1409 w1418 w1427 w1436 w1445 w1454 w1461 w1468 w1475 w1478 w1494 w1521 w1560 w1569 w1585 w1588 w1606 w1611 w1616 w1621] -> w10
      tunnel: [w21 w579 w588 w606 w613 w628 w634 w647 w659 w676 w682 w708 w713 w724 w735 w746 w759 w779 w797 w807 w861 w914 w946 w959 w973 w986 w1005 w1028 w1065 w1079 w1089 w1097 w1112 w1119 w1126 w1148 w1166 w1174 w1184 w1219 w1223 w1228 w1235 w1240 w1269 w1299 w1308 w1312 w1333 w1343 w1352 w1365 w1380 w1396 w1407 w1412 w1425 w1432 w1444 w1453 w1460 w1464 w1472 w1479 w1487 w1517 w1557 w1570 w1580 w1589 w1603 w1612 w1617 w1622] -> w9
      tunnel: [w23 w581 w592 w605 w614 w631 w636 w645 w655 w675 w684 w689 w714 w717 w728 w740 w757 w768 w784 w817 w851 w915 w947 w960 w965 w978 w991 w1016 w1053 w1074 w1090 w1098 w1114 w1121 w1129 w1149 w1163 w1171 w1183 w1216 w1224 w1231 w1236 w1239 w1282 w1304 w1309 w1316 w1336 w1345 w1357 w1368 w1381 w1398 w1404 w1416 w1421 w1430 w1441 w1450 w1457 w1465 w1471 w1480 w1483 w1518 w1540 w1571 w1575 w1590 w1594 w1613 w1618 w1623] -> w6
      tunnel: w5 -> [w22 w581 w591 w605 w610 w631 w636 w645 w662 w677 w684 w688 w714 w720 w731 w742 w752 w776 w794 w804 w852 w910 w947 w960 w969 w983 w1001 w1020 w1060 w1075 w1090 w1098 w1114 w1121 w1129 w1149 w1164 w1172 w1187 w1216 w1224 w1231 w1236 w1242 w1282 w1304 w1309 w1317 w1337 w1346 w1358 w1369 w1386 w1395 w1405 w1413 w1423 w1431 w1442 w1451 w1458 w1466 w1473 w1480 w1483 w1516 w1545 w1571 w1576 w1590 w1596 w1613 w1618 w1623]
      tunnel: w4 -> [w20 w579 w588 w599 w613 w628 w634 _ w660 w676 w682 w708 w713 w723 w734 w745 w758 w778 w796 w807 w861 w914 w946 w959 w973 w986 w1005 w1028 w1065 w1079 w1089 w1097 w1112 w1119 w1126 w1148 w1166 w1174 w1184 w1219 w1223 w1228 w1235 w1240 w1269 w1299 w1308 w1312 w1333 w1343 w1352 w1365 w1380 w1396 w1407 w1412 w1425 w1432 w1444 w1453 w1460 w1464 w1472 w1479 w1488 w1517 w1557 w1570 w1578 w1589 w1602 w1612 w1617 w1622]
      frame "", "Idle" {
        # "executes when the state queue is empty"
        n6 = event shown="[17] \"REF Channels\": Value Change" {
          selector: w18 -> [_ _ _ _ _ _ _ _ _ _ _ _ _ _ _ _ _ _ _ _ _ _ _ _ _ _ _ _ _ _ _ _ _ _ _ _ _ w390 _ _ _ _ _ _ _ _ _ _ _ _ _ _ _]
          dyn-events: _ -> [_ _ _ _ _ _ _ _ _ _ _ _ _ _ _ _ _ _ _ _ _ _ _ _ _ _ _ _ _ _ _ _ _ _ _ _ _ _ _ _ _ _ _ _ _ _ _ _ _ _ _ _ _]
          timeout: w19 -> [_ _ _ _ _ _ _ _ _ _ _ _ _ _ _ _ _ _ _ _ _ _ _ _ _ _ _ _ _ _ _ _ _ _ _ _ _ _ _ _ _ _ _ _ _ _ _ _ _ _ _ _ _]
          tunnel: w25 -> [w33 w59 w94 w103 w112 w119 w125 w131 w146 w153 w160 w173 w178 w188 w194 w202 w211 w226 w253 w268 w281 w283 w293 w299 w303 w308 w313 w318 w323 w328 w333 w338 w343 w348 w353 w358 w367 w397 w445 w457 w467 w474 w482 w490 w497 w504 w510 w530 w539 w548 w557 w563 w570]
          tunnel: [w31 w58 w93 w102 w111 w118 w124 w130 w145 w152 w161 w174 w179 w187 w193 w203 w212 w227 w252 w267 w280 w284 w292 w298 w304 w309 w314 w319 w324 w329 w334 w339 w344 w349 w354 w359 w366 w396 w444 w456 w466 w473 w481 w489 w496 w503 w509 w529 w538 w547 w556 w562 w574] -> w24
          tunnel: [w28 w44 w89 w95 w109 w116 w122 w128 w140 w149 w157 w164 w175 w180 w192 w195 w204 w213 w249 w261 w274 w285 w291 w297 w301 w306 w311 w316 w321 w326 w331 w336 w341 w346 w351 w356 w365 w391 w443 w454 w464 w471 w479 w487 w494 w501 w508 w515 w537 w545 w554 w559 w573] -> w23
          tunnel: w22 -> [w28 w46 w89 w95 w109 w116 w122 w128 w140 w149 w157 w164 w175 w180 w192 w195 w204 w213 w241 w256 w274 w285 w291 w297 w301 w306 w311 w316 w321 w326 w331 w336 w341 w346 w351 w356 w365 w392 w443 w454 w464 w471 w479 w487 w494 w501 w508 w528 w537 w545 w554 w560 w573]
          tunnel: [w32 w57 w91 w100 w104 w117 w123 w126 w147 w154 w158 w171 w176 w186 w191 w201 w210 w224 w251 w265 w278 w286 w289 w295 w302 w307 w312 w317 w322 w327 w332 w337 w342 w347 w352 w357 w364 w395 w442 w455 w465 w472 w480 w488 w495 w502 w507 w519 w536 w546 w555 w561 w572] -> w21
          tunnel: w20 -> [w32 w56 w90 w99 w105 w117 w123 w126 w148 w154 w158 w170 w176 w185 w191 w199 w208 w221 w250 w264 w277 w286 w289 w295 w302 w307 w312 w317 w322 w327 w332 w337 w342 w347 w352 w357 w363 w394 w442 w455 w465 w472 w480 w488 w495 w502 w507 w519 w536 w546 w555 w561 w572]
          event Timeout {
            n7 = event-data() -> ()  [unwired: 1 in, 1 out]
            n8 = Unbundle By Name(w32) -> ("Lockin"=w27:refnum<class "Instrument.Lockin.lvclass">)
            n9 = Unbundle By Name(w27) -> ("DAQ state"=w26:T32)
            n10 = case shown="\"idle\"" w26 {
              tunnel: [w36 w40 w42] -> w30
              frame "idle" {
                n11 = call "Spinner.vi"("Enum"=enum16{"Spinner 1", "Spinner 2", "Spinner 3"}."Spinner 1") -> ("Spinner Out"=w34:string)  [unwired: 4 in]
                n12 = Concatenate Strings("Idle     " ("Status"), w34) -> (w36:string)
              }
              frame "created" {
                n13 = call "Spinner.vi"("Enum"=enum16{"Spinner 1", "Spinner 2", "Spinner 3"}."Spinner 1") -> ("Spinner Out"=w38:string)  [unwired: 4 in]
                n14 = Concatenate Strings("Created  " ("Status"), w38) -> (w40:string)
              }
              frame Default {
                n15 = local read "Status"() -> (w42:string)
              }
            }
            "Status" <- w30
            n16 = call <vilib>:"Add State(s) to Queue__jki_lib_state_machine.vi"("State(s) in Front (\"\")"="" ("t"), "State(s) in (\"\")"=w33) -> ("States Out"=w31:string)  [unwired: 13 in]
          }
          event User Event {
            n17 = event-data() -> ("AO"=w54:waveform(dbl)[], "AI"=w50:waveform(dbl)[], "RefX"=w53:waveform(dbl)[], "RefY"=w52:waveform(dbl)[])  [unwired: 1 in]
            n18 = call <userlib>:"MGI Milliseconds Since Last Call.vi"("Error In"=w46) -> ("ms"=w43:u32, "Error Out"=w45:errorcluster)  [unwired: 5 in]
            "Refresh time (ms)" <- w43
            n19 = disable-structure shown="Enabled" {
              disable-tunnel: w45 -> [w76 w84]
              disable-tunnel: [w75 w84] -> w44
              disable-tunnel: w50 -> [w68 _]
              disable-tunnel: w43 -> [w67 _]
              frame Enabled {
                n20 = Index Array(array=w68) -> (element=w83:waveform(dbl))  [unwired: 1 in]
                n21 = call-poly <vilib>:"Waveform Duration.vi"("error in (no error)"=w76, "waveform in"=w83) -> ("error out"=w75:errorcluster, "duration"=w82:dbl)  [unwired: 7 in, 1 out]
                n22 = Multiply(x=w82, y=1000.0) -> (x*y=w73:dbl)
                n23 = Multiply(x=w73, y=2.0) -> (x*y=w72:dbl)
                n24 = Less?(x=w67, y=w72) -> (x < y?=w70:bool)
                n25 = Select(t="Good", s=w70, f="#s/Fs: too small!") -> (s? t:f=→"Sampling Status":string)
                n26 = Select(t=u32 6618880, s=w70, f=u32 16711680) -> (s? t:f=w80:u32)
                n27 = property on="Sampling Status" class="Str"("Text.BGColor"=w80) -> ()  [unwired: 2 in, 2 out]
              }
              frame Disabled {
              }
            }
            n28 = Unbundle By Name(w56) -> ("Lockin"=w55:refnum<class "Instrument.Lockin.lvclass">)
            n29 = Bundle By Name(cluster=w55, "AO"=w54, "AI"=w50, "RefX"=w53, "RefY"=w52) -> (w51:refnum<class "Instrument.Lockin.lvclass">)
            n30 = call <userlib>:"Periodic Trigger__ogtk.vi"("time (ms)"=u32 100) -> ("Triggered"=w48:bool)  [unwired: 12 in, 2 out]
            n31 = case shown="True" w48 {
              tunnel: ["" ("State(s) in Front (\"\")") w63] -> w47
              frame False {
              }
              frame True {
                n32 = local read "Tab Control 2"() -> (w64:T20)
                n33 = case shown="\"PS\"" w64 {
                  tunnel: ["" ("State(s) in Front (\"\")") "4461: FFT" ("State(s) in Front (\"\")")] -> w62
                  frame Default {
                  }
                  frame "PS" {
                  }
                }
                n34 = call <vilib>:"Add State(s) to Queue__jki_lib_state_machine.vi"("State(s) in Front (\"\")"="4461: OUT\nUI: Update Waveform Graphs\nUI: Sync AO AI Plot Visibility\nUI: Update Lockin Graphs\nUI: Sync Lockin Plot Visibility\nUI: Update Sweep Timer" ("State(s) in Front (\"\")"), "State(s) at Back (\"\")"=w62) -> ("States Out"=w63:string)  [unwired: 13 in]
              }
            }
            n35 = Bundle By Name(cluster=w56, "Lockin"=w51) -> (w57:T36)
            n36 = call <vilib>:"Add State(s) to Queue__jki_lib_state_machine.vi"("State(s) in Front (\"\")"=w47, "State(s) in (\"\")"=w59) -> ("States Out"=w58:string)  [unwired: 13 in]
          }
          event User Event {
            n37 = event-data() -> ("Sweep AO"=w88:waveform(dbl)[], "Sweep AI"=w85:waveform(dbl)[], "Sweep Results X"=w86:waveform(dbl)[], "Sweep Results Y"=w87:waveform(dbl)[])  [unwired: 1 in]
            n38 = Bundle By Name(cluster=w90, "SweepWaveforms.Sweep AO"=w88, "SweepWaveforms.Sweep AI"=w85, "SweepWaveforms.Sweep Results X"=w86, "SweepWaveforms.Sweep Results Y"=w87) -> (w91:T36)
            n39 = call <vilib>:"Add State(s) to Queue__jki_lib_state_machine.vi"("State(s) in Front (\"\")"="UI: Update Sweep WFMs Graphs" ("State(s) in Front (\"\")"), "State(s) in (\"\")"=w94) -> ("States Out"=w93:string)  [unwired: 13 in]
          }
          event User Event {
            n40 = event-data() -> ("AO"=w96:waveform(dbl)[])  [unwired: 1 in, 4 out]
            n41 = Unbundle By Name(w99) -> ("Lockin"=w98:refnum<class "Instrument.Lockin.lvclass">)
            n42 = Bundle By Name(cluster=w98, "AO"=w96) -> (w97:refnum<class "Instrument.Lockin.lvclass">)
            n43 = local write "AO Channels"(w96) -> ()
            n44 = Bundle By Name(cluster=w99, "Lockin"=w97) -> (w100:T36)
            n45 = call <vilib>:"Add State(s) to Queue__jki_lib_state_machine.vi"("State(s) in Front (\"\")"="" ("State(s) in Front (\"\")"), "State(s) in (\"\")"=w103) -> ("States Out"=w102:string)  [unwired: 13 in]
          }
          event User Event {
            n46 = event-data() -> ("state"=w106:T37)  [unwired: 1 in, 4 out]
            n47 = case shown="Default" w106 {
              frame Default {
              }
              frame "sweeping" {
                n48 = call <userlib>:"MGI Milliseconds Since Last Reset.vi"("Reset (F)"=TRUE) -> ()  [unwired: 5 in, 2 out]
              }
            }
            n49 = Unbundle By Name(w105) -> ("Lockin"=w108:refnum<class "Instrument.Lockin.lvclass">)
            n50 = Bundle By Name(cluster=w108, "DAQ state"=w106) -> (w107:refnum<class "Instrument.Lockin.lvclass">)
            n51 = Bundle By Name(cluster=w105, "Lockin"=w107) -> (w104:T36)
            n52 = call <vilib>:"Add State(s) to Queue__jki_lib_state_machine.vi"("State(s) in Front (\"\")"="UI: Update Status" ("State(s) in Front (\"\")"), "State(s) in (\"\")"=w112) -> ("States Out"=w111:string)  [unwired: 13 in]
          }
          event User Event {
            # "Check Calibrate Mode Button Value Change (pressed) Event"
            n53 = event-data() -> ("Channels: REF"=→"Cal Info":T38)  [unwired: 1 in]
            n54 = call <vilib>:"Add State(s) to Queue__jki_lib_state_machine.vi"("State(s) in (\"\")"=w119, "State(s) at Back (\"\")"="" ("State(s) at Back (\"\")")) -> ("States Out"=w118:string)  [unwired: 13 in]
          }
          event User Event {
            # "Check Calibrate Mode Button Value Change (pressed) Event"
            n55 = event-data() -> ("New Ch []"=w120:T39)  [unwired: 1 in]
            n56 = property on="DAQ Config" class="Arr (strict)"("Val(Sgnl)"=w120) -> ()  [unwired: 2 in, 2 out]
            n57 = call <vilib>:"Add State(s) to Queue__jki_lib_state_machine.vi"("State(s) in (\"\")"=w125, "State(s) at Back (\"\")"="" ("State(s) at Back (\"\")")) -> ("States Out"=w124:string)  [unwired: 13 in]
          }
          event User Event {
            # "#framework\n????"
            n58 = event-data() -> ("SMO State"=w127:T16)  [unwired: 1 in]
            "LockinDAQ SMO State" <- w127
            n59 = case shown="\"Started\"" w127 {
              tunnel: ["UI: Enable Buttons" ("State Queue") "" ("State Queue")] -> w129
              frame "Started" {
              }
              frame Default {
              }
            }
            n60 = call <vilib>:"Add State(s) to Queue__jki_lib_state_machine.vi"("State(s) in Front (\"\")"=w129, "State(s) in (\"\")"=w131) -> ("States Out"=w130:string)  [unwired: 13 in]
          }
          event User Event {
            # "#framework"
            # "here command should be argument?"
            # "#todo: future: call Command: Handle Command"
            # "Message sent by the RemoteControl.lvclass:process"
            n61 = event-data() -> ("Message"=w141:T34, "Message.Command"=w137:string)  [unwired: 1 in, 3 out]
            n62 = Concatenate Strings("Command: ", w137) -> (w136:string)
            n63 = call <userlib>:"MGI String Pattern Match Exists.vi"("Patterns to Try"=string[] ["getAOconfig", "getSampling", "getREFconfig", "getInputGain", "getOutputGain", "getAO", "getAI", "getResults", "getStatus", "getSweepResults", "getSweepWaveforms", "getAutoSampling", "getState", "setAO", "setAO_Amplitude", "setAO_DC", "setAO_Frequency", "setAO_Phase", "setAO_Function", "setREF", "setREF_Frequency", "setREF_Phase", "setREF_TC", "setREF_RollOff", "setSweepConfiguration", "setState", "setSampling", "setSamplingMode", "setInputGain", "setOutputGain", "setDAQ", "HELP", "ACK", "getAll"] ("Array"), "String"=w137) -> ("Match Found"=w139:bool)  [unwired: 1 out]
            n64 = Select(t="" ("State(s) in Front (\"\")"), s=w139, f=w136) -> (s? t:f=w134:string)
            n65 = Bundle By Name(cluster=w148, "Message"=w141) -> (w147:T36)
            n66 = call <vilib>:"Add State(s) to Queue__jki_lib_state_machine.vi"("State(s) in Front (\"\")"=w134, "State(s) at Back (\"\")"="") -> ("States Out"=w143:string)  [unwired: 13 in]
            n67 = call <vilib>:"Add State(s) to Queue__jki_lib_state_machine.vi"("State(s) in Front (\"\")"=w143, "State(s) in (\"\")"=w146) -> ("States Out"=w145:string)  [unwired: 13 in]
          }
          event User Event {
            # "Disable: I think this could cause an infinite loop when trying to exit"
            n68 = event-data() -> ("SMO State"=w150:T16)  [unwired: 1 in]
            "RC SMO State" <- w150
            n69 = case shown="\"Started\"" w150 {
              tunnel: ["" ("State Queue") "" ("State Queue")] -> w151
              frame "Started" {
              }
              frame Default {
              }
            }
            n70 = call <vilib>:"Add State(s) to Queue__jki_lib_state_machine.vi"("State(s) in Front (\"\")"=w151, "State(s) in (\"\")"=w153) -> ("States Out"=w152:string)  [unwired: 13 in]
          }
          event Value Change {
            n71 = event-data() -> ()  [unwired: 1 in, 6 out]
            n72 = call <vilib>:"Add State(s) to Queue__jki_lib_state_machine.vi"("State(s) in Front (\"\")"="" ("State(s) in Front (\"\")"), "State(s) in (\"\")"=w160) -> ("States Out"=w161:string)  [unwired: 13 in]
          }
          event "DAQ Config": Value Change {
            w168 = -1 items=["Default"=-1, "RSE"=10083, "Differential"=10106, "Pseudodifferential"=12529] ("output terminal configuration")
            w169 = -1 items=["Default"=-1, "RSE"=10083, "NRSE"=10078, "Differential"=10106, "Pseudodifferential"=12529] ("input terminal configuration")
            n73 = event-data() -> ("NewVal"=w167:T6[])  [unwired: 1 in]
            n74 = Unbundle By Name(w170) -> ("Lockin"=w166:refnum<class "Instrument.Lockin.lvclass">)
            n75 = call "config UI to not UI (AO and AI).vi"("output terminal configuration"=w168, "input terminal configuration"=w169, "New Ch []"=w167) -> ("AO Config"=w162:T44, "AI Config"=w163:T46)  [unwired: 7 in]
            n76 = Bundle By Name(cluster=w166, "AI"=w163, "AO"=w162) -> (w165:refnum<class "Instrument.Lockin.lvclass">)
            n77 = Bundle By Name(cluster=w170, "Lockin"=w165) -> (w171:T36)
            n78 = call <vilib>:"Add State(s) to Queue__jki_lib_state_machine.vi"("State(s) in Front (\"\")"="Lockin SMO: Set AO Config\nLockin SMO: Set AI Config\nUI: Update AI Ch\nUI: Update Plot Names" ("State(s) in Front (\"\")"), "State(s) in (\"\")"=w173) -> ("States Out"=w174:string)  [unwired: 13 in]
          }
          event Value Change {
            n79 = event-data() -> ()  [unwired: 1 in, 1 out]
            n80 = call <vilib>:"Add State(s) to Queue__jki_lib_state_machine.vi"("State(s) in Front (\"\")"="Lockin SMO: Set AI Config" ("State(s) in Front (\"\")"), "State(s) in (\"\")"=w178) -> ("States Out"=w179:string)  [unwired: 13 in]
          }
          event Value Change {
            n81 = event-data() -> ("NewVal"=w181:T11)  [unwired: 1 in, 1 out]
            n82 = Unbundle By Name(w185) -> ("Lockin"=w183:refnum<class "Instrument.Lockin.lvclass">)
            n83 = Bundle By Name(cluster=w183, "Sampling"=w181) -> (w182:refnum<class "Instrument.Lockin.lvclass">)
            n84 = Bundle By Name(cluster=w185, "Lockin"=w182) -> (w186:T36)
            n85 = call <vilib>:"Add State(s) to Queue__jki_lib_state_machine.vi"("State(s) in Front (\"\")"="Macro: Update Sampling" ("State(s) in Front (\"\")"), "State(s) in (\"\")"=w188) -> ("States Out"=w187:string)  [unwired: 13 in]
          }
          event "Auto x*F1", "Max Fs Refresh Rate (Hz)", "decimating factor": Value Change {
            n86 = event-data() -> ()  [unwired: 1 in, 6 out]
            n87 = call <vilib>:"Add State(s) to Queue__jki_lib_state_machine.vi"("State(s) in Front (\"\")"="Macro: Update Sampling" ("State(s) in Front (\"\")")) -> ("States Out"=w190:string)  [unwired: 14 in]
            n88 = call <vilib>:"Add State(s) to Queue__jki_lib_state_machine.vi"("State(s) in Front (\"\")"=w190, "State(s) in (\"\")"=w194) -> ("States Out"=w193:string)  [unwired: 13 in]
          }
          event "AO Channels": Value Change {
            n89 = event-data() -> ("NewVal"=w196:T4)  [unwired: 1 in, 5 out]
            n90 = Unbundle By Name(w199) -> ("Lockin"=w198:refnum<class "Instrument.Lockin.lvclass">)
            n91 = Bundle By Name(cluster=w198, "AO"=w196) -> (w197:refnum<class "Instrument.Lockin.lvclass">)
            n92 = Bundle By Name(cluster=w199, "Lockin"=w197) -> (w201:T36)
            n93 = call <vilib>:"Add State(s) to Queue__jki_lib_state_machine.vi"("State(s) in Front (\"\")"="Data: Adjust Channels\nUI: Update Rings\nLockin SMO: Set AO" ("f"), "State(s) in (\"\")"=w202) -> ("States Out"=w203:string)  [unwired: 13 in]
          }
          event "AI Channels": Value Change {
            n94 = event-data() -> ("NewVal"=w205:T2)  [unwired: 1 in]
            n95 = Unbundle By Name(w208) -> ("Lockin"=w207:refnum<class "Instrument.Lockin.lvclass">)
            n96 = Bundle By Name(cluster=w207, "AI"=w205) -> (w206:refnum<class "Instrument.Lockin.lvclass">)
            n97 = Bundle By Name(cluster=w208, "Lockin"=w206) -> (w210:T36)
            n98 = call <vilib>:"Add State(s) to Queue__jki_lib_state_machine.vi"("State(s) in Front (\"\")"="UI: Update Rings\nLockin SMO: Set AI" ("f"), "State(s) in (\"\")"=w211) -> ("States Out"=w212:string)  [unwired: 13 in]
          }
          event "REF Channels": Value Change {
            # "#todo\nthis \"macro\" needs to\nbe handled by Lockin.DAQ\nor Handle Command"
            # "if number of lockin channels is not the same as before reset the lockin\nupdate: no, just reset phase...?"
            n99 = event-data() -> ("NewVal"=w214:T5[], "OldVal"=w218:T5[])  [unwired: 1 in]
            n100 = Unbundle By Name(w221) -> ("Lockin"=w216:refnum<class "Instrument.Lockin.lvclass">)
            n101 = Bundle By Name(cluster=w216, "REF"=w214) -> (w215:refnum<class "Instrument.Lockin.lvclass">)
            n102 = Not Equal?(x=w214, y=w218) -> (x != y?=w219:bool)
            n103 = Unbundle By Name(w215) -> ("DAQ state"=w217:T32)
            n104 = case shown="\"created\"" w217 {
              tunnel: ["" ("f") w235] -> _
              tunnel: w219 -> [_ w234]
              frame "idle", Default {
              }
              frame "created" {
                n105 = Format Into String(Set_State-enum."start" ("State")) -> (resulting string=w237:string)  [unwired: 3 in, 1 out]
                n106 = call <vilib>:"Build State String with Arguments__JKI_lib_State_Machine.vi"("Arguments (\"\")"=w237, "State"="Lockin SMO: Set State" ("f")) -> ("State with Arguments"=w240:string)  [unwired: 4 in]
                n107 = Select(t=w240, s=w234, f="") -> (s? t:f=w235:string)
              }
            }
            n108 = case shown="\"created\"" w217 {
              tunnel: ["" ("State with Arguments") w229] -> w222
              frame "idle", Default {
              }
              frame "created" {
                n109 = Format Into String(Set_State-enum."stop" ("State")) -> (resulting string=w232:string)  [unwired: 3 in, 1 out]
                n110 = call <vilib>:"Build State String with Arguments__JKI_lib_State_Machine.vi"("Arguments (\"\")"=w232, "State"="Lockin SMO: Set State" ("f")) -> ("State with Arguments"=w229:string)  [unwired: 4 in]
              }
            }
            n111 = Bundle By Name(cluster=w221, "Lockin"=w215) -> (w224:T36)
            n112 = Select(t=w222, s=w219, f="") -> ()  [unwired: 1 out]
            n113 = call <vilib>:"Add State(s) to Queue__jki_lib_state_machine.vi"("State(s) in (\"\")"="Data: Adjust Channels\nUI: Update Rings\nUI: Update Plot Names\nLockin SMO: Set REF\nLockin SMO: Reset Phase" ("f")) -> ("States Out"=w223:string)  [unwired: 14 in]
            n114 = call <vilib>:"Add State(s) to Queue__jki_lib_state_machine.vi"("State(s) in Front (\"\")"=w223, "State(s) in (\"\")"=w226) -> ("States Out"=w227:string)  [unwired: 13 in]
          }
          event "Input Gain": Value Change {
            n115 = event-data() -> ("NewVal"=w247:cluster{"AI.Ch":string, "Gain":dbl}[])  [unwired: 1 in, 5 out]
            n116 = for {
              tunnel: w247 -> [w255] mode=indexing
              tunnel: [w254] -> w242 mode=indexing
              n117 = Unbundle(w255) -> ("Gain"=w254:dbl)  [unwired: 1 out]
            }
            n118 = Unbundle By Name(w250) -> ("Lockin"=w245:refnum<class "Instrument.Lockin.lvclass">)
            n119 = Bundle By Name(cluster=w245, "AI.Gain"=w242) -> (w244:refnum<class "Instrument.Lockin.lvclass">)
            n120 = call "Initialize Input Gain.vi"("error in (no error)"=w241, "Instrument.DAQ"=w244) -> ("error out"=w249:errorcluster, "Input Gain"=w243:T48, "Instrument.DAQ out"=w248:refnum<class "Instrument.DAQ.lvclass">)  [unwired: 7 in]
            n121 = local write "Input Gain"(w243) -> ()
            n122 = Bundle By Name(cluster=w250, "Lockin"=w248) -> (w251:T36)
            n123 = call <vilib>:"Add State(s) to Queue__jki_lib_state_machine.vi"("State(s) in Front (\"\")"="Lockin SMO: Set Input Gain" ("State(s) in Front (\"\")"), "State(s) in (\"\")"=w253) -> ("States Out"=w252:string)  [unwired: 13 in]
          }
          event "Output Gain": Value Change {
            n124 = event-data() -> ("NewVal"=w263:cluster{"AI.Ch":string, "Gain":dbl}[])  [unwired: 1 in, 5 out]
            n125 = for {
              tunnel: w263 -> [w270] mode=indexing
              tunnel: [w269] -> w259 mode=indexing
              n126 = Unbundle(w270) -> ("Gain"=w269:dbl)  [unwired: 1 out]
            }
            n127 = Unbundle By Name(w264) -> ("Lockin"=w258:refnum<class "Instrument.Lockin.lvclass">)
            n128 = Bundle By Name(cluster=w258, "AO.Gain"=w259) -> (w257:refnum<class "Instrument.Lockin.lvclass">)
            n129 = call "Initialize Ouput Gain.vi"("error in (no error)"=w256, "Instrument.DAQ"=w257) -> ("error out"=w261:errorcluster, "Output Gain"=w260:T48, "Instrument.DAQ out"=w262:refnum<class "Instrument.DAQ.lvclass">)  [unwired: 7 in]
            n130 = local write "Output Gain"(w260) -> ()
            n131 = Bundle By Name(cluster=w264, "Lockin"=w262) -> (w265:T36)
            n132 = call <vilib>:"Add State(s) to Queue__jki_lib_state_machine.vi"("State(s) in Front (\"\")"="Lockin SMO: Set Output Gain" ("State(s) in Front (\"\")"), "State(s) in (\"\")"=w268) -> ("States Out"=w267:string)  [unwired: 13 in]
          }
          event "Line", "Lowpass", "LP f (Hz)": Value Change {
            n133 = event-data() -> ()  [unwired: 1 in, 6 out]
            n134 = Unbundle By Name(w277) -> ("Lockin"=w276:refnum<class "Instrument.Lockin.lvclass">)
            n135 = Bundle By Name(cluster=w276, "60 Hz"="Line", "Low Pass"="Lowpass", "Low Pass Cutoff (Hz)"="LP f (Hz)") -> (w275:refnum<class "Instrument.Lockin.lvclass">)
            n136 = Bundle By Name(cluster=w277, "Lockin"=w275) -> (w278:T36)
            n137 = call <vilib>:"Add State(s) to Queue__jki_lib_state_machine.vi"("State(s) in Front (\"\")"="Lockin SMO: Set Prefilter" ("State(s) in Front (\"\")"), "State(s) in (\"\")"=w281) -> ("States Out"=w280:string)  [unwired: 13 in]
          }
          event "Allowed remote system": Value Change {
            n138 = event-data() -> ()  [unwired: 1 in, 6 out]
            n139 = call <vilib>:"Add State(s) to Queue__jki_lib_state_machine.vi"("State(s) in Front (\"\")"="" ("State(s) in Front (\"\")"), "State(s) in (\"\")"=w283) -> ("States Out"=w284:string)  [unwired: 13 in]
          }
          event "Self Calibrate": Value Change {
            # "Self Calibrate Mode Button Value Change (pressed) Event"
            n140 = event-data() -> ()  [unwired: 1 in, 2 out]
            n141 = local write "Self Calibrate"(FALSE ("Self Calibrate")) -> ()
            n142 = property on="Pause" class="Bool (strict)"("Val(Sgnl)"=TRUE ("Value (Signaling)")) -> ()  [unwired: 2 in, 2 out]
            n143 = call <vilib>:"Add State(s) to Queue__jki_lib_state_machine.vi"("State(s) in Front (\"\")"="\nLockin SMO: Calibration >> True" ("f"), "State(s) in (\"\")"=w293) -> ("States Out"=w292:string)  [unwired: 13 in]
          }
          event "Get Calibration": Value Change {
            # "Self Calibrate Mode Button Value Change (pressed) Event"
            n144 = event-data() -> ()  [unwired: 1 in, 2 out]
            n145 = local write "Get Calibration"(FALSE ("Self Calibrate")) -> ()
            n146 = call <vilib>:"Add State(s) to Queue__jki_lib_state_machine.vi"("State(s) in Front (\"\")"="Lockin SMO: Calibration >> False" ("f"), "State(s) in (\"\")"=w299) -> ("States Out"=w298:string)  [unwired: 13 in]
          }
          event "X Axis": Value Change {
            # "X Axis, Y Axis Out Value Change (pressed) Event\ncall: UI: Update Waveform Graph Labels"
            n147 = event-data() -> ()  [unwired: 1 in, 6 out]
            n148 = call <vilib>:"Add State(s) to Queue__jki_lib_state_machine.vi"("State(s) in Front (\"\")"="UI: Update Waveform Graph Labels" ("State(s) in Front (\"\")"), "State(s) in (\"\")"=w303) -> ("States Out"=w304:string)  [unwired: 13 in]
          }
          event "Y Axis (Output)": Value Change {
            # "X Axis, Y Axis Out Value Change (pressed) Event\ncall: UI: Update Waveform Graph Labels"
            n149 = event-data() -> ()  [unwired: 1 in, 6 out]
            n150 = call <vilib>:"Add State(s) to Queue__jki_lib_state_machine.vi"("State(s) in Front (\"\")"="UI: Update Plot Names" ("State(s) in Front (\"\")"), "State(s) in (\"\")"=w308) -> ("States Out"=w309:string)  [unwired: 13 in]
          }
          event "AI Graph All": Value Change {
            # "X Axis, Y Axis Out Value Change (pressed) Event\ncall: UI: Update Waveform Graph Labels"
            n151 = event-data() -> ()  [unwired: 1 in, 6 out]
            n152 = call <vilib>:"Add State(s) to Queue__jki_lib_state_machine.vi"("State(s) in Front (\"\")"="UI: AI Graph Plot Visible >> All" ("State(s) in Front (\"\")"), "State(s) in (\"\")"=w313) -> ("States Out"=w314:string)  [unwired: 13 in]
          }
          event "AI Graph None": Value Change {
            # "X Axis, Y Axis Out Value Change (pressed) Event\ncall: UI: Update Waveform Graph Labels"
            n153 = event-data() -> ()  [unwired: 1 in, 6 out]
            n154 = call <vilib>:"Add State(s) to Queue__jki_lib_state_machine.vi"("State(s) in Front (\"\")"="UI: AI Graph Plot Visible >> None" ("State(s) in Front (\"\")"), "State(s) in (\"\")"=w318) -> ("States Out"=w319:string)  [unwired: 13 in]
          }
          event "AO Graph All": Value Change {
            # "X Axis, Y Axis Out Value Change (pressed) Event\ncall: UI: Update Waveform Graph Labels"
            n155 = event-data() -> ()  [unwired: 1 in, 6 out]
            n156 = call <vilib>:"Add State(s) to Queue__jki_lib_state_machine.vi"("State(s) in Front (\"\")"="UI: AO Graph Plot Visible >> All" ("State(s) in Front (\"\")"), "State(s) in (\"\")"=w323) -> ("States Out"=w324:string)  [unwired: 13 in]
          }
          event "AO Graph None": Value Change {
            # "X Axis, Y Axis Out Value Change (pressed) Event\ncall: UI: Update Waveform Graph Labels"
            n157 = event-data() -> ()  [unwired: 1 in, 6 out]
            n158 = call <vilib>:"Add State(s) to Queue__jki_lib_state_machine.vi"("State(s) in Front (\"\")"="UI: AO Graph Plot Visible >> None" ("State(s) in Front (\"\")"), "State(s) in (\"\")"=w328) -> ("States Out"=w329:string)  [unwired: 13 in]
          }
          event "Lockin 1 All": Value Change {
            # "X Axis, Y Axis Out Value Change (pressed) Event\ncall: UI: Update Waveform Graph Labels"
            n159 = event-data() -> ()  [unwired: 1 in, 6 out]
            n160 = call <vilib>:"Add State(s) to Queue__jki_lib_state_machine.vi"("State(s) in Front (\"\")"="UI: Lockin 1 Plot Visible >> All" ("State(s) in Front (\"\")"), "State(s) in (\"\")"=w333) -> ("States Out"=w334:string)  [unwired: 13 in]
          }
          event "Lockin 1 None": Value Change {
            # "X Axis, Y Axis Out Value Change (pressed) Event\ncall: UI: Update Waveform Graph Labels"
            n161 = event-data() -> ()  [unwired: 1 in, 6 out]
            n162 = call <vilib>:"Add State(s) to Queue__jki_lib_state_machine.vi"("State(s) in Front (\"\")"="UI: Lockin 1 Plot Visible >> None" ("State(s) in Front (\"\")"), "State(s) in (\"\")"=w338) -> ("States Out"=w339:string)  [unwired: 13 in]
          }
          event "Update": Value Change {
            # "Update Value Change (pressed) Event\ncall: AUX: Set AUX"
            n163 = event-data() -> ()  [unwired: 1 in, 6 out]
            n164 = call <vilib>:"Add State(s) to Queue__jki_lib_state_machine.vi"("State(s) in Front (\"\")"="AUX: Set AUX" ("State(s) in Front (\"\")"), "State(s) in (\"\")"=w343) -> ("States Out"=w344:string)  [unwired: 13 in]
          }
          event "Numeric", "X/R Range", "Y/Theta Range": Value Change {
            # "X&Y Axis Range\", \"XorR Axis Range\", \"YorTheta Axis Range\" Value Change (pressed) Event\ncall: UI: Update Lockin Graph Range"
            n165 = event-data() -> ()  [unwired: 1 in, 6 out]
            n166 = call <vilib>:"Add State(s) to Queue__jki_lib_state_machine.vi"("State(s) in Front (\"\")"="UI: Update Lockin Graph Range" ("State(s) in Front (\"\")"), "State(s) in (\"\")"=w348) -> ("States Out"=w349:string)  [unwired: 13 in]
          }
          event "Link Frequencies", "Limit Amplitudes", "AO freq link": Value Change {
            # "Same f\", \"Limit Amp\", \"AO freq link\": Value Change Value Change (pressed) Event\ncall:\nData: Adjust Channels\nConfiguration: Write\nLockin SMO: Set AO\nLockin SMO: Set REF"
            n167 = event-data() -> ()  [unwired: 1 in, 6 out]
            n168 = call <vilib>:"Add State(s) to Queue__jki_lib_state_machine.vi"("State(s) in Front (\"\")"="Data: Adjust Channels\nUI: Update Rings\nLockin SMO: Set AO\nLockin SMO: Set REF" ("f"), "State(s) in (\"\")"=w353) -> ("States Out"=w354:string)  [unwired: 13 in]
          }
          event Value Change {
            # "Display Value Change Value Change (pressed) Event\ncall:\nUI: Update Displays"
            n169 = event-data() -> ()  [unwired: 1 in, 6 out]
            n170 = call <vilib>:"Add State(s) to Queue__jki_lib_state_machine.vi"("State(s) in Front (\"\")"="UI: Update Displays" ("f"), "State(s) in (\"\")"=w358) -> ("States Out"=w359:string)  [unwired: 13 in]
          }
          event "Start": Value Change {
            # "Start Button Value Change (pressed) Event\nIf DAQ=idle:\n1. Set Sampling to Continuous Samples\n2. Start acquisition\n3. Set Pause=False\n4. Set timout=10\n\nIf DAQ=running:\n1. Do nothing"
            n171 = event-data() -> ()  [unwired: 1 in, 2 out]
            n172 = Unbundle By Name(w363) -> ("Lockin"=w361:refnum<class "Instrument.Lockin.lvclass">)
            n173 = Unbundle By Name(w361) -> ("DAQ state"=w360:T32)
            n174 = case shown="\"idle\", Default" w360 {
              tunnel: [w374 "" ("State with Arguments")] -> w362
              tunnel: w363 -> [w380 w386]
              tunnel: [w379 w386] -> w364
              frame "idle", Default {
                w375 = T50 10123 items=["Finite Samples"=10178, "Continuous Samples"=10123] ("Sample Mode")
                n175 = local write "Pause"(FALSE ("Pause")) -> ()
                n176 = Format Into String(w375) -> (resulting string=w376:string)  [unwired: 3 in, 1 out]
                n177 = Format Into String(Set_State-enum."start" ("State")) -> (resulting string=w384:string)  [unwired: 3 in, 1 out]
                n178 = First Call?() -> (First Call?: T/F=w371:bool)
                n179 = call <vilib>:"Build State String with Arguments__JKI_lib_State_Machine.vi"("Arguments (\"\")"=w376, "State"="Lockin SMO: Set Sampling" ("f")) -> ("State with Arguments"=w373:string)  [unwired: 4 in]
                n180 = call <vilib>:"Build State String with Arguments__JKI_lib_State_Machine.vi"("Arguments (\"\")"=w384, "State"="Lockin SMO: Set State" ("f")) -> ("State with Arguments"=w372:string)  [unwired: 4 in]
                n181 = Select(t="Macro: Update Sampling" ("f"), s=w371, f="") -> (s? t:f=w369:string)
                n182 = call <vilib>:"Add State(s) to Queue__jki_lib_state_machine.vi"("State(s) in Front (\"\")"=w369, "State(s) in (\"\")"=w373, "State(s) at Back (\"\")"=w372) -> ("States Out"=w374:string)  [unwired: 12 in]
                n183 = Bundle By Name(cluster=w380, "to"=-1) -> (w379:T36)
              }
              frame "created" {
              }
            }
            n184 = call <vilib>:"Add State(s) to Queue__jki_lib_state_machine.vi"("State(s) in (\"\")"=w367, "State(s) at Back (\"\")"=w362) -> ("States Out"=w366:string)  [unwired: 13 in]
          }
          event "Pause": Value Change {
            # "Pause Button Value Change (pressed) Event\nPause=True & DAQ=running:\n1. Set Sampling to Finite Samples\n2. STOP acquisition\n3. Set timeout=-1 (wait forever)\nPause=True & DAQ=idle\n1. Set timeout=-1\n2. Set Sampling to Finite\nPause=False:\n1. send T=Val(Sgnl) to Start"
            n185 = event-data() -> ("NewVal"=w393:bool)  [unwired: 1 in]
            n186 = Unbundle By Name(w394) -> ("Lockin"=w388:refnum<class "Instrument.Lockin.lvclass">)
            n187 = Unbundle By Name(w388) -> ("DAQ state"=w387:T32)
            n188 = Flush Event Queue(0:w390, 3:w392) -> (11:w391:errorcluster)  [unwired: 4 in, 2 out]
            n189 = case shown="True" w393 {
              tunnel: [w399 "" ("States Out")] -> w389
              tunnel: w394 -> [w401 w427]
              tunnel: [w400 w427] -> w395
              tunnel: w387 -> [w398 _]
              frame True {
                n190 = case shown="\"started\"" w398 {
                  tunnel: w401 -> [w406 w422]
                  tunnel: [w405 w421] -> w400
                  tunnel: [w402 w412] -> w399
                  frame "idle", Default {
                    w408 = T50 10178 items=["Finite Samples"=10178, "Continuous Samples"=10123] ("Sample Mode")
                    n191 = Format Into String(w408) -> (resulting string=w409:string)  [unwired: 3 in, 1 out]
                    n192 = call <vilib>:"Build State String with Arguments__JKI_lib_State_Machine.vi"("Arguments (\"\")"=w409, "State"="Lockin SMO: Set Sampling" ("f")) -> ("State with Arguments"=w403:string)  [unwired: 4 in]
                    n193 = call <vilib>:"Add State(s) to Queue__jki_lib_state_machine.vi"("State(s) at Back (\"\")"=w403) -> ("States Out"=w402:string)  [unwired: 14 in]
                    n194 = Bundle By Name(cluster=w406, "to"=100) -> (w405:T36)
                  }
                  frame "started" {
                    w417 = T50 10178 items=["Finite Samples"=10178, "Continuous Samples"=10123] ("Sample Mode")
                    n195 = Format Into String(Set_State-enum."stop" ("State")) -> (resulting string=w425:string)  [unwired: 3 in, 1 out]
                    n196 = Format Into String(w417) -> (resulting string=w418:string)  [unwired: 3 in, 1 out]
                    n197 = call <vilib>:"Build State String with Arguments__JKI_lib_State_Machine.vi"("Arguments (\"\")"=w425, "State"="Lockin SMO: Set State" ("f")) -> ("State with Arguments"=w410:string)  [unwired: 4 in]
                    n198 = call <vilib>:"Build State String with Arguments__JKI_lib_State_Machine.vi"("Arguments (\"\")"=w418, "State"="Lockin SMO: Set Sampling" ("f")) -> ("State with Arguments"=w411:string)  [unwired: 4 in]
                    n199 = local write "Status"("Finite Acquisition" ("Status")) -> ()
                    n200 = call <vilib>:"Add State(s) to Queue__jki_lib_state_machine.vi"("State(s) in Front (\"\")"="Lockin SMO: Set AO Zero Amplitude" ("f"), "State(s) in (\"\")"=w411, "State(s) at Back (\"\")"=w410) -> ("States Out"=w414:string)  [unwired: 12 in]
                    n201 = Bundle By Name(cluster=w422, "to"=100) -> (w421:T36)
                    n202 = call <vilib>:"Add State(s) to Queue__jki_lib_state_machine.vi"("State(s) in Front (\"\")"=w414, "State(s) at Back (\"\")"="Lockin SMO: Set AO" ("f")) -> ("States Out"=w412:string)  [unwired: 13 in]
                  }
                }
              }
              frame False {
                n203 = property on="Start" class="Bool (strict)"("Val(Sgnl)"=TRUE ("Value (Signaling)")) -> ()  [unwired: 2 in, 2 out]
              }
            }
            n204 = call <vilib>:"Add State(s) to Queue__jki_lib_state_machine.vi"("State(s) in Front (\"\")"=w389, "State(s) in (\"\")"=w397) -> ("States Out"=w396:string)  [unwired: 13 in]
          }
          event "Trigger": Value Change {
            w441 = T50 10178 items=["Finite Samples"=10178, "Continuous Samples"=10123] ("Sample Mode")
            # "Trigger Button Value Change (pressed) Event\nIf DAQ=idle:\n1. put into finite sample mode\n2. start (one) acquisition)\nIf DAQ=running:\n1. Stop current acquisition\n2. put into finite sample mode\n3. start (one) acquisition)"
            n205 = event-data() -> ()  [unwired: 1 in, 2 out]
            n206 = disable-structure shown="Disabled" {
              frame Disabled {
                n207 = local write "Trigger"(FALSE ("Trigger")) -> ()
              }
              frame Enabled {
              }
            }
            n208 = Unbundle By Name(w442) -> ("Lockin"=w429:refnum<class "Instrument.Lockin.lvclass">)
            n209 = Unbundle By Name(w429) -> ("DAQ state"=w430:T32)
            n210 = case shown="\"created\"" w430 {
              tunnel: ["" ("State with Arguments") w448] -> w433
              frame "idle", Default {
              }
              frame "created" {
                n211 = Format Into String(Set_State-enum."stop" ("State")) -> (resulting string=w451:string)  [unwired: 3 in, 1 out]
                n212 = call <vilib>:"Build State String with Arguments__JKI_lib_State_Machine.vi"("Arguments (\"\")"=w451, "State"="Lockin SMO: Set State" ("f")) -> ("State with Arguments"=w448:string)  [unwired: 4 in]
              }
            }
            n213 = local write "Pause"(TRUE ("Pause")) -> ()
            n214 = Format Into String(w441) -> (resulting string=w440:string)  [unwired: 3 in, 1 out]
            n215 = Format Into String(Set_State-enum."start" ("State")) -> (resulting string=w436:string)  [unwired: 3 in, 1 out]
            n216 = call <vilib>:"Build State String with Arguments__JKI_lib_State_Machine.vi"("Arguments (\"\")"=w440, "State"="Lockin SMO: Set Sampling" ("f")) -> ("State with Arguments"=w435:string)  [unwired: 4 in]
            n217 = call <vilib>:"Build State String with Arguments__JKI_lib_State_Machine.vi"("Arguments (\"\")"=w436, "State"="Lockin SMO: Set State" ("f")) -> ("State with Arguments"=w434:string)  [unwired: 4 in]
            n218 = call <vilib>:"Add State(s) to Queue__jki_lib_state_machine.vi"("State(s) in Front (\"\")"=w433, "State(s) in (\"\")"=w435, "State(s) at Back (\"\")"=w434) -> ("States Out"=w432:string)  [unwired: 12 in]
            n219 = call <vilib>:"Add State(s) to Queue__jki_lib_state_machine.vi"("State(s) in Front (\"\")"=w432, "State(s) in (\"\")"=w445) -> ("States Out"=w444:string)  [unwired: 13 in]
          }
          event "Reset": Value Change {
            # "RESET Button Value Change (pressed) Event\n1. Call 4461: SETUP State to calculate new Sampling\ninformation\n2. If sampling information changes, \"Sampling: value\nchange event will be triggered.\n3. Sampling: Value Change will call Stop, Set Sampling, Start"
            n220 = event-data() -> ()  [unwired: 1 in, 1 out]
            n221 = disable-structure shown="Disabled" {
              frame Disabled {
                n222 = Format Into String(Set_State-enum."reset" ("State")) -> (resulting string=w460:string)  [unwired: 3 in, 1 out]
                n223 = call <vilib>:"Build State String with Arguments__JKI_lib_State_Machine.vi"("Arguments (\"\")"=w460, "State"="Lockin SMO: Set State" ("f")) -> ()  [unwired: 4 in, 1 out]
              }
              frame Enabled {
              }
            }
            n224 = local write "Reset"(FALSE ("Reset")) -> ()
            n225 = call <vilib>:"Add State(s) to Queue__jki_lib_state_machine.vi"("State(s) in Front (\"\")"="Macro: Initialize UI\nMacro: Initialize DAQ SMO\n//UI: Update Plot Names >>Reset" ("State(s) in Front (\"\")"), "State(s) in (\"\")"=w457) -> ("States Out"=w456:string)  [unwired: 13 in]
          }
          event "Measure": Value Change {
            # "Measure Offset Button Value Change (pressed) Event\n1. send \"measure offset\" command to DAQ"
            n226 = event-data() -> ()  [unwired: 1 in, 1 out]
            n227 = local write "Measure"(FALSE ("Measure\nOffset")) -> ()
            n228 = call <vilib>:"Add State(s) to Queue__jki_lib_state_machine.vi"("State(s) in Front (\"\")"="Lockin SMO: Measure Offset" ("State(s) in Front (\"\")")) -> ("States Out"=w463:string)  [unwired: 14 in]
            n229 = call <vilib>:"Add State(s) to Queue__jki_lib_state_machine.vi"("State(s) in Front (\"\")"=w463, "State(s) in (\"\")"=w467) -> ("States Out"=w466:string)  [unwired: 13 in]
          }
          event "Reset Phase": Value Change {
            # "Measure Offset Button Value Change (pressed) Event\n1. send \"measure offset\" command to DAQ"
            n230 = event-data() -> ()  [unwired: 1 in, 1 out]
            n231 = local write "Reset Phase"(FALSE ("Measure\nOffset")) -> ()
            n232 = call <vilib>:"Add State(s) to Queue__jki_lib_state_machine.vi"("State(s) in Front (\"\")"="Lockin SMO: Reset Phase" ("State(s) in Front (\"\")")) -> ("States Out"=w470:string)  [unwired: 14 in]
            n233 = call <vilib>:"Add State(s) to Queue__jki_lib_state_machine.vi"("State(s) in Front (\"\")"=w470, "State(s) in (\"\")"=w474) -> ("States Out"=w473:string)  [unwired: 13 in]
          }
          event "Disable all AI Ref": Value Change {
            # "Measure Offset Button Value Change (pressed) Event\n1. send \"measure offset\" command to DAQ"
            n234 = event-data() -> ()  [unwired: 1 in, 1 out]
            n235 = local write "Disable all AI Ref"(FALSE ("Measure\nOffset")) -> ()
            n236 = call <vilib>:"Build State String with Arguments__JKI_lib_State_Machine.vi"("Arguments (\"\")"="Disable" ("Arguments (\"\")"), "State"="UI: Update AI Reference Channels" ("State(s) in Front (\"\")")) -> ("State with Arguments"=w478:string)  [unwired: 4 in]
            n237 = call <vilib>:"Add State(s) to Queue__jki_lib_state_machine.vi"("State(s) in Front (\"\")"=w478, "State(s) in (\"\")"=w482) -> ("States Out"=w481:string)  [unwired: 13 in]
          }
          event "Enable only AI Ref1": Value Change {
            # "Measure Offset Button Value Change (pressed) Event\n1. send \"measure offset\" command to DAQ"
            n238 = event-data() -> ()  [unwired: 1 in, 1 out]
            n239 = local write "Enable only AI Ref1"(FALSE ("Measure\nOffset")) -> ()
            n240 = call <vilib>:"Build State String with Arguments__JKI_lib_State_Machine.vi"("Arguments (\"\")"="All 1" ("Arguments (\"\")"), "State"="UI: Update AI Reference Channels" ("State(s) in Front (\"\")")) -> ("State with Arguments"=w486:string)  [unwired: 4 in]
            n241 = call <vilib>:"Add State(s) to Queue__jki_lib_state_machine.vi"("State(s) in Front (\"\")"=w486, "State(s) in (\"\")"=w490) -> ("States Out"=w489:string)  [unwired: 13 in]
          }
          event "auto DAQ": Value Change {
            # "Measure Offset Button Value Change (pressed) Event\n1. send \"measure offset\" command to DAQ"
            n242 = event-data() -> ()  [unwired: 1 in, 1 out]
            n243 = local write "auto DAQ"(FALSE ("Measure\nOffset")) -> ()
            n244 = call <vilib>:"Add State(s) to Queue__jki_lib_state_machine.vi"("State(s) in Front (\"\")"="Lockin SMO: Auto DAQ" ("State(s) in Front (\"\")")) -> ("States Out"=w493:string)  [unwired: 14 in]
            n245 = call <vilib>:"Add State(s) to Queue__jki_lib_state_machine.vi"("State(s) in Front (\"\")"=w493, "State(s) in (\"\")"=w497) -> ("States Out"=w496:string)  [unwired: 13 in]
          }
          event "Remove": Value Change {
            # "Zero Offset Button Value Change (pressed) Event\n1. send \"zero offset\" command to DAQ"
            n246 = event-data() -> ()  [unwired: 1 in, 1 out]
            n247 = local write "Remove"(FALSE ("Zero\nOffset")) -> ()
            n248 = call <vilib>:"Add State(s) to Queue__jki_lib_state_machine.vi"("State(s) in Front (\"\")"="Lockin SMO: Remove Offset" ("State(s) in Front (\"\")")) -> ("States Out"=w500:string)  [unwired: 14 in]
            n249 = call <vilib>:"Add State(s) to Queue__jki_lib_state_machine.vi"("State(s) in Front (\"\")"=w500, "State(s) in (\"\")"=w504) -> ("States Out"=w503:string)  [unwired: 13 in]
          }
          event "Close": Value Change {
            w505 = "Macro: Exit"
            # "Stop Button Value Change (pressed) Event\n(this executes Macro: Exit to terminate the VI)"
            n250 = event-data() -> ("OldVal"=w506:bool)  [unwired: 1 in]
            n251 = local write "Close"(w506) -> ()
            n252 = disable-structure shown="Disabled" {
              disable-tunnel: w505 -> [w511 _]
              frame Disabled {
                n253 = Two Button Dialog(message="Are you sure you want to exit?") -> (T button?=w513:bool)  [unwired: 2 in]
                n254 = Select(t=w511, s=w513, f="") -> ()  [unwired: 1 out]
              }
              frame Enabled {
              }
            }
            n255 = call <vilib>:"Add State(s) to Queue__jki_lib_state_machine.vi"("State(s) in Front (\"\")"=w505, "State(s) in (\"\")"=w510) -> ("States Out"=w509:string)  [unwired: 13 in]
          }
          event "Start Sweep": Value Change {
            # "New Start Button Value Change (pressed) Event"
            n256 = event-data() -> ()  [unwired: 1 in, 1 out]
            n257 = Unbundle By Name(w519) -> ("Lockin.DAQ"=w517:refnum<class "Instrument.DAQ.lvclass">)
            n258 = Bundle By Name(cluster=T23 {"Sweep Time (s)"=0.0, "Initial Wait (s)"=0.0, "Return to Start"=FALSE, "Channels"=[]} ("Configure Sweep"), "Channels"="Channels: Sweep", "Sweep Time (s)"="Sweep Time (s)", "Initial Wait (s)"="Initial Wait (s)", "Return to Start"="Return to Start?") -> (w526:T23)
            n259 = call "DAQ.setSweep.vi"("error in (no error)"=w528, "setSweep"=w526, "Instrument.DAQ"=w517) -> ("error out"=w515:errorcluster)  [unwired: 7 in, 1 out]
            n260 = Format Into String(Set_State-enum."start sweep" ("State")) -> (resulting string=w525:string)  [unwired: 3 in, 1 out]
            n261 = call <vilib>:"Build State String with Arguments__JKI_lib_State_Machine.vi"("Arguments (\"\")"=w525, "State"="Lockin SMO: Set State" ("f")) -> ("State with Arguments"=w522:string)  [unwired: 4 in]
            n262 = call <vilib>:"Add State(s) to Queue__jki_lib_state_machine.vi"("State(s) in Front (\"\")"=w522, "State(s) in (\"\")"=w530) -> ("States Out"=w529:string)  [unwired: 13 in]
          }
          event "Stop Sweep": Value Change {
            # "New Start Button Value Change (pressed) Event"
            n263 = event-data() -> ()  [unwired: 1 in, 6 out]
            n264 = local write "Stop Sweep"(FALSE ("Sweep Start")) -> ()
            n265 = Format Into String(Set_State-enum."stop sweep" ("State")) -> (resulting string=w534:string)  [unwired: 3 in, 1 out]
            n266 = call <vilib>:"Build State String with Arguments__JKI_lib_State_Machine.vi"("Arguments (\"\")"=w534, "State"="Lockin SMO: Set State" ("f")) -> ("State with Arguments"=w531:string)  [unwired: 4 in]
            n267 = call <vilib>:"Add State(s) to Queue__jki_lib_state_machine.vi"("State(s) in Front (\"\")"=w531, "State(s) in (\"\")"=w539) -> ("States Out"=w538:string)  [unwired: 13 in]
          }
          event "Load Configuration": Value Change {
            # "LOAD CONFIG Button Value Change (pressed) Event"
            n268 = event-data() -> ("NewVal"=w544:bool)  [unwired: 1 in, 1 out]
            n269 = local write "Load Configuration"(FALSE ("load config")) -> ()
            n270 = Select(t="" ("State(s) at Back (\"\")"), s=w544, f="") -> (s? t:f=w541:string)
            n271 = call <vilib>:"Add State(s) to Queue__jki_lib_state_machine.vi"("State(s) in Front (\"\")"=w541, "State(s) in (\"\")"=w548) -> ("States Out"=w547:string)  [unwired: 13 in]
          }
          event "Save Configuration": Value Change {
            # "save config Button Value Change (pressed) Event"
            n272 = event-data() -> ("NewVal"=w551:bool)  [unwired: 1 in]
            n273 = local write "Save Configuration"(FALSE ("save config")) -> ()
            n274 = Select(t="" ("State(s) at Back (\"\")"), s=w551, f="") -> (s? t:f=w552:string)
            n275 = call <vilib>:"Add State(s) to Queue__jki_lib_state_machine.vi"("State(s) in Front (\"\")"=w552, "State(s) in (\"\")"=w557) -> ("States Out"=w556:string)  [unwired: 13 in]
          }
          event "Help": Value Change {
            # "Help Button Value Change (pressed) Event\nIf Help = True: Send user to help webpage; Set Help=False\nIf Help=Fale, Do nothing"
            n276 = event-data() -> ("NewVal"=w558:bool)  [unwired: 1 in]
            n277 = case shown="False" w558 {
              tunnel: w560 -> [w564 w568]
              tunnel: [w564 w566] -> w559
              frame False {
              }
              frame True {
                n278 = local write "Help"(FALSE ("Help")) -> ()
                n279 = call-poly <vilib>:"Open URL in Default Browser.vi"("error in (no error)"=w568, "URL"="https://app.asana.com/0/205665857037275/list") -> ("error out"=w566:errorcluster)  [unwired: 4 in, 1 out]
              }
            }
            n280 = call <vilib>:"Add State(s) to Queue__jki_lib_state_machine.vi"("State(s) in (\"\")"=w563) -> ("States Out"=w562:string)  [unwired: 14 in]
          }
          event Panel Close? {
            w569 = "Macro: Exit"
            # "Discard the event because we'll close the front panel ourselves in Macro: Exit"
            # "Close Panel button (pressed) Event\n(this executes Macro: Exit to terminate the VI)"
            n281 = event-data() -> ()  [unwired: 1 in, 1 out]
            n282 = disable-structure shown="Disabled" {
              disable-tunnel: w569 -> [w575 _]
              frame Disabled {
                n283 = Two Button Dialog(message="Are you sure you want to exit?") -> (T button?=w577:bool)  [unwired: 2 in]
                n284 = Select(t=w575, s=w577, f="") -> ()  [unwired: 1 out]
              }
              frame Enabled {
              }
            }
            n285 = call <vilib>:"Add State(s) to Queue__jki_lib_state_machine.vi"("State(s) in Front (\"\")"=w569, "State(s) in (\"\")"=w570) -> ("States Out"=w574:string)  [unwired: 13 in]
            n286 = event-data("Discard?"=TRUE) -> ()  [unwired: 1 in, 1 out]
          }
        }
      }
      frame "---------- Core ----------" {
        # "Do not put any code in this frame.\n(it is a separator no-op)"
        n287 = call <vilib>:"Add State(s) to Queue__jki_lib_state_machine.vi"("State(s) in (\"\")"=w583) -> ("States Out"=w582:string)  [unwired: 14 in]
      }
      frame Default {
        w595 = 42 items=["No error", "Argument error", "Memory is full", "Out of zone", "End of file", "File already open", "Generic file I/O error", "File not found", "File permission error", "Disk is full", "Duplicate path", "Too many files open", "System feature not enabled", "Resource file not found", "Cannot add resource", "Resource not found", "Image not found", "Image memory error", "Pen does not exist", "Config type invalid", "Config token not found", "Config parse error", "Config memory error", "Bad external code format", "Bad external code offset", "External code not present", "Null window", "Destroy window error", "Null menu", "Print aborted", "Bad print record", "Print driver error", "Windows error during printing", "Memory error during printing", "Print dialog error", "Generic print error", "Invalid device refnum", "Device not found", "Device parameter error", "Device unit error", "Cannot open device", "Device call aborted", "Generic error", "Cancelled by user", "Object ID too low", "Object ID too high", "Object not in heap", "Unknown heap", "Unknown object (invalid DefProc)", "Unknown object (DefProc not in table)", "Message out of range", "Invalid (null) method", "Unknown message", "Manager call not supported", "Bad address", "Network operation in progress", "Network operation timed out", "Connection is busy", "Network attribute not supported", "Network error", "Address in use", "System out of memory", "Connection aborted", "Connection refused", "Not connected", "Already connected", "Connection closed", "Initialization error (interapplication manager)", "Bad occurrence", "Wait on unbound occurrence handler", "Occurrence queue overflow", "Datalog type conflict", "Unused", "Unrecognized type (interapplication manager)", "Memory corrupt", "Failed to make temporary DLL", "Old CIN version", "Drag socket not found", "Failed to load drop-object", "Failed to register OLE object", "Failed to release OLE object", "Format specifier type mismatch", "Unknown format specifier", "Too few format specifiers", "Too many format specifiers", "Scan failed", "Newer CIN version", "Error converting to variant", "Runtime menu error", "Password tampered", "Variant attribute not found", "Incompatible variant data type", "Event data is not available", "Event Store is not present", "Occurrence is not found", "Event Queue is not created", "Event info is not available", "Refnum passed is NULL", "Error retrieving Class GUID", "Error retrieving CoClass GUID", "Error retrieving TypeLib GUID.", "Bad built application magic bytes.", "Specific driver is different from the specific driver associated with the Logical Name.", "There is no session opened to the class driver.", "Max Error", "MAX - Error with config objects", "MAX - Error loading configuration", "MAX - Group not supported"]
        # "Current State"
        # "Do not delete, rename, or modify this frame.\n(this is used to capture unhandled states and typos)"
        # "Handle mistyped state name (developer tool)"
        n288 = Format Into String(format string="Software Exception: Unhandled State \"%s\"." ("message"), error in=w591, w586) -> (resulting string=w594:string, error out=w593:errorcluster)  [unwired: 1 in]
        n289 = call <vilib>:"Error Cluster From Error Code.vi"("show call chain? (False)"=TRUE, "error in (no error)"=w593, "error message (\"\")"=w594, "error code (0)"=w595) -> ("error out"=w592:errorcluster)  [unwired: 5 in]
        n290 = call <vilib>:"Add State(s) to Queue__jki_lib_state_machine.vi"("State(s) in (\"\")"=w590) -> ("States Out"=w589:string)  [unwired: 14 in]
      }
      frame "Initialize Core Data" {
        # "Do not delete, rename, or modify this frame.\n(this is used to determine panel behavior on exit)"
        # "originally closed?"
        # "exe?"
        # "If panel starts closed or is an EXE, then close it when we exit"
        n291 = property class="VI"() -> ("Front Panel.Open"=w604:bool)  [unwired: 2 in, 2 out]
        n292 = property class="App"() -> ("App.Kind"=w603:T26)  [unwired: 2 in, 2 out]
        n293 = control-ref of="Current VI Reference"() -> (w597:refnum<vi>)
        n294 = Not(x=w604) -> (.not. x?=w601:bool)
        n295 = Equal?(x=w603, y=T26."Run Time System" ("Application:Kind")) -> (x = y?=w600:bool)
        n296 = Or(x=w601, y=w600) -> (x .or. y?=w598:bool)
        n297 = Bundle By Name(cluster=w599, "Core.Current VI Reference"=w597, "Core.Close Panel on Exit?"=w598) -> (w606:T36)
        n298 = call <vilib>:"Add State(s) to Queue__jki_lib_state_machine.vi"("State(s) in (\"\")"=w608) -> ("States Out"=w607:string)  [unwired: 14 in]
      }
      frame "Error Handler" {
        # "Handle any errors here.\nYou can also output any states to clean-up after errors occur"
        # "Clear error"
        n299 = Unbundle By Name(w613) -> ("Lockin"=w612:refnum<class "Instrument.Lockin.lvclass">)
        n300 = call-dynamic "Handle Error.vi"("Stop on Unhandled Error (T)"=FALSE, "error in"=w610, "SMO"=w612) -> ("handling error"=w609:errorcluster)  [unwired: 6 in, 2 out]
        n301 = call-poly <userlib>:"Filter Error Codes__ogtk.vi"("Error In"=w609, "Error Codes to Filter"=i32[] [-200077, -200462, -200245, -200279]) -> ("Error Out"=w617:errorcluster)  [unwired: 7 in, 2 out]
        n302 = case shown="Error" w617 {
          selector: w617 -> [w622 w627]
          tunnel: ["" "Macro: Exit"] -> w619
          tunnel: [w622 w624] -> w615
          frame No Error {
          }
          frame Error {
            w625 = T51 1 items=["no dialog", "OK message", "continue or stop message", "OK message + warnings", "continue/stop + warnings"] ("type of dialog (OK msg:1)")
            # "Unhandled Error -- Display it"
            n303 = call <vilib>:"General Error Handler.vi"("type of dialog (OK msg:1)"=w625, "error in (no error)"=w627) -> ("error out"=w624:errorcluster)  [unwired: 9 in, 4 out]
          }
        }
        n304 = call <userlib>:"Clear All Errors__ogtk.vi"("Error In"=w615) -> ("Error Out"=w614:errorcluster)  [unwired: 3 in]
        n305 = call <vilib>:"Add State(s) to Queue__jki_lib_state_machine.vi"("State(s) in Front (\"\")"=w619, "State(s) in (\"\")"=w621) -> ("States Out"=w620:string)  [unwired: 13 in]
      }
      frame "Exit" {
        # "Do not put any code in this frame.\n(No errors that occur here will be handled.)"
        n306 = call <vilib>:"Add State(s) to Queue__jki_lib_state_machine.vi"("State(s) in (\"\")"=w633) -> ("States Out"=w632:string)  [unwired: 14 in]
      }
      frame "---------- Data ----------" {
        # "Do not put any code in this frame.\n(It is a separator no-op. You can make a copy of this frame to create a new Data frame)"
        n307 = call <vilib>:"Add State(s) to Queue__jki_lib_state_machine.vi"("State(s) in (\"\")"=w638) -> ("States Out"=w637:string)  [unwired: 14 in]
      }
      frame "Data: Initialize" {
        w640 = T34 {"Command"="", "Data"=variant, "ID"=""}  # Message
        w641 = refnum<class "Logger.Error.lvclass"> refnum  # Logger.Error
        w643 = refnum<class "Instrument.DAQ.lvclass"> refnum  # Lockin.DAQ
        w646 = T35 {"Sweep AO"=[], "Sweep AI"=[], "Sweep Results X"=[], "Sweep Results Y"=[]}  # SweepWaveforms
        w648 = T33 {"address"="", "Port"=0, "AllowedRemote"="", "Commands"=[], "timeout"=0}  # RemoteControl.Configure
        (unwired) T52 {"Time Stamp"=timestamp(0 s since 1904-01-01), "Results (Dictionary)"=[]}  # Results
        w649 = T34 {"Command"="", "Data"=variant, "ID"=""}  # HandledMessage
        w639 = refnum<class "Instrument.Lockin.lvclass"> refnum  # Lockin
        w642 = refnum<class "RemoteControl.lvclass"> refnum  # RemoteControl
        (unwired) waveform(dbl)[] []  # AI WFM
        w644 = 100  # to
        (unwired) waveform(dbl)[] []  # AO WFM
        (unwired) waveform(dbl)[] []  # REF WFM
        w651 = T53 {"Current VI Reference"=refnum, "Close Panel on Exit?"=FALSE}  # Core
        # "#todo\nPut all of this stuff on the class wire\nso I can use Handle Command.vi..."
        # "is sent to RC:process"
        # "comes from RC:process"
        # "do not delete - used by framework"
        # "Initialize the shift-register data, here.\n(data names are defined by what you wire into the bundle function)"
        n308 = call <vilib>:"Add State(s) to Queue__jki_lib_state_machine.vi"("State(s) in (\"\")"=w653) -> ("States Out"=w652:string)  [unwired: 14 in]
        n309 = Bundle("Core"=w651, "to"=w644, "Lockin"=w639, "RemoteControl"=w642, "Lockin.DAQ"=w643, "Logger.Error"=w641, "RemoteControl.Configure"=w648, "Message"=w640, "HandledMessage"=w649, "SweepWaveforms"=w646) -> (w647:T36)  [unwired: 1 in]
      }
      frame "Data: Adjust Channels" {
        # "#todo\nshould some of these methods be owned by Lockin.DAQ?"
        n310 = Unbundle By Name(w660) -> ("Lockin"=w661:refnum<class "Instrument.Lockin.lvclass">)
        n311 = call "Initialize REF Channels.vi"("error in (no error)"=w662, "Instrument.DAQ"=w661) -> ("error out"=w663:errorcluster, "Instrument.DAQ out"=w664:refnum<class "Instrument.DAQ.lvclass">)  [unwired: 8 in]
        n312 = call "Initialize AO Channels.vi"("error in (no error)"=w663, "Instrument.DAQ"=w664) -> ("error out"=w668:errorcluster, "Instrument.DAQ out"=w670:refnum<class "Instrument.DAQ.lvclass">)  [unwired: 8 in]
        n313 = call "Limit AO Amplitude.vi"("error in (no error)"=w668, 9:"Limit Amplitudes", 10:"AO Amp Limit", "Instrument.DAQ"=w670) -> ("error out"=w667:errorcluster, "Instrument.DAQ out"=w669:refnum<class "Instrument.DAQ.lvclass">)  [unwired: 6 in]
        n314 = call "Set all f same.vi"("error in (no error)"=w667, 9:"Link Frequencies", 10:"AO freq link", "Instrument.DAQ"=w669) -> ("error out"=w655:errorcluster, "Instrument.DAQ out"=w665:refnum<class "Instrument.DAQ.lvclass">)  [unwired: 6 in]
        n315 = Unbundle By Name(w665) -> ("AO"=w654, "REF"=w671)
        n316 = Bundle By Name(cluster=w660, "Lockin"=w665) -> (w659:T36)
        n317 = local write "REF Channels"(w671) -> ()
        n318 = local write "AO Channels"(w654) -> ()
        n319 = call <vilib>:"Add State(s) to Queue__jki_lib_state_machine.vi"("State(s) in (\"\")"=w674) -> ("States Out"=w673:string)  [unwired: 14 in]
      }
      frame "Data: Cleanup" {
        # "Cleanup any data and references, here.\n(this is called automatically, by the Macro: Exit)"
        n320 = Unbundle By Name(w676) -> ("Core.Current VI Reference"=w678:refnum<vi>)
        n321 = Close Reference(reference=w678, error in (no error)=w677) -> (error out=w675:errorcluster)
        n322 = call <vilib>:"Add State(s) to Queue__jki_lib_state_machine.vi"("State(s) in (\"\")"=w681) -> ("States Out"=w680:string)  [unwired: 14 in]
      }
      frame "---------- Events ----------" {
        # "Template Separator\n(You can make a copy of, or modify, this frame)"
        n323 = call <vilib>:"Add State(s) to Queue__jki_lib_state_machine.vi"("State(s) in (\"\")"=w686) -> ("States Out"=w685:string)  [unwired: 14 in]
      }
      frame "Events: Register" {
        w695 = T54 {"Error"=refnum, "State"=refnum, "Reserve State"=refnum}  # LockinDAQ SMO Public Events
        w704 = T54 {"Error"=refnum, "State"=refnum, "Reserve State"=refnum}  # RC SMO Public Events
        n324 = Unbundle By Name(w708) -> ("RemoteControl"=w700:refnum<class "RemoteControl.lvclass">, "Lockin.DAQ"=w687:refnum<class "Instrument.DAQ.lvclass">)
        n325 = call <vilib>:"GetPublicEvents.vi"("SMO"=w700) -> ("error out"=w699:errorcluster, "Public Events"=w703:T54, "SMO out"=w697:refnum<class "RemoteControl.lvclass">)  [unwired: 8 in]
        n326 = Variant To Data(error in=w699, type=w704, Variant=w703) -> (data=w702:T54, error out=w698:errorcluster)
        n327 = call <vilib>:"GetPublicEvents.vi"("SMO"=w687) -> ("error out"=w692:errorcluster, "Public Events"=w694:T54, "SMO out"=w690:refnum<class "Instrument.DAQ.lvclass">)  [unwired: 8 in]
        n328 = call <userlib>:"RemoteControl.GetPublicEvents.vi"("RemoteControl"=w697) -> ("error out"=w696:errorcluster, "RC Public Events"=w707:T55)  [unwired: 8 in, 1 out]
        n329 = Variant To Data(error in=w692, type=w695, Variant=w694) -> (data=w693:T54, error out=w691:errorcluster)
        n330 = call "DAQ.GetPublicEvents.vi"("Instrument.DAQ"=w690) -> ("error out"=w705:errorcluster, "DAQ Public Events"=w701:T56)  [unwired: 8 in, 1 out]
        n331 = register-events(w702, w707, w693, w701) -> (reference out=w709:refnum<event-registration>, error out=w706:errorcluster)  [unwired: 2 in]
        n332 = Merge Errors(w706, w705, w696, w691, w698, w688) -> (w689:errorcluster)
        n333 = call <vilib>:"Add State(s) to Queue__jki_lib_state_machine.vi"("State(s) in (\"\")"=w711) -> ("States Out"=w710:string)  [unwired: 14 in]
      }
      frame "---------- UI ----------" {
        # "Do not put any code in this frame.\n(It is a separator no-op. You can make a copy of this frame to create a new UI frame)"
        n334 = call <vilib>:"Add State(s) to Queue__jki_lib_state_machine.vi"("State(s) in (\"\")"=w716) -> ("States Out"=w715:string)  [unwired: 14 in]
      }
      frame "UI: Initialize REF Ch" {
        n335 = Unbundle By Name(w723) -> ("Lockin"=w722:refnum<class "Instrument.Lockin.lvclass">)
        n336 = call "Initialize REF Channels.vi"("error in (no error)"=w720, "Instrument.DAQ"=w722) -> ("error out"=w718:errorcluster, 2:w719, "Instrument.DAQ out"=w721:refnum<class "Instrument.DAQ.lvclass">)  [unwired: 7 in]
        n337 = property on="REF Channels" class="Arr (strict)"(error in=w718, "Val(Sgnl)"=w719) -> (error out=w717:errorcluster)  [unwired: 1 in, 1 out]
        n338 = Bundle By Name(cluster=w723, "Lockin"=w721) -> (w724:T36)
        n339 = call <vilib>:"Add State(s) to Queue__jki_lib_state_machine.vi"("State(s) in (\"\")"=w727) -> ("States Out"=w726:string)  [unwired: 14 in]
      }
      frame "UI: Initialize AO Ch" {
        n340 = Unbundle By Name(w734) -> ("Lockin"=w733:refnum<class "Instrument.Lockin.lvclass">)
        n341 = call "Initialize AO Channels.vi"("error in (no error)"=w731, "Instrument.DAQ"=w733) -> ("error out"=w730:errorcluster, 2:w729, "Instrument.DAQ out"=w732:refnum<class "Instrument.DAQ.lvclass">)  [unwired: 7 in]
        n342 = property on="AO Channels" class="Arr (strict)"(error in=w730, "Val(Sgnl)"=w729) -> (error out=w728:errorcluster)  [unwired: 1 in, 1 out]
        n343 = Bundle By Name(cluster=w734, "Lockin"=w732) -> (w735:T36)
        n344 = call <vilib>:"Add State(s) to Queue__jki_lib_state_machine.vi"("State(s) in (\"\")"=w738) -> ("States Out"=w737:string)  [unwired: 14 in]
      }
      frame "UI: Update AI Ch" {
        # "Add or remove AI channels"
        n345 = Unbundle By Name(w745) -> ("Lockin"=w743:refnum<class "Instrument.Lockin.lvclass">)
        n346 = call "Initialize AI Channels.vi"("error in (no error)"=w742, "Instrument.DAQ"=w743) -> ("error out"=w741:errorcluster, 2:w744, "Instrument.DAQ out"=w739:refnum<class "Instrument.DAQ.lvclass">)  [unwired: 7 in]
        n347 = property on="AI Channels" class="Arr (strict)"(error in=w741, "Val(Sgnl)"=w744) -> (error out=w740:errorcluster)  [unwired: 1 in, 1 out]
        n348 = Bundle By Name(cluster=w745, "Lockin"=w739) -> (w746:T36)
        n349 = call <vilib>:"Add State(s) to Queue__jki_lib_state_machine.vi"("State(s) in (\"\")"=w749) -> ("States Out"=w748:string)  [unwired: 14 in]
      }
      frame "UI: Update AI Reference Channels" {
        # "Add or remove AI channels"
        n350 = Unbundle By Name(w758) -> ("Lockin"=w755:refnum<class "Instrument.Lockin.lvclass">)
        n351 = case shown="\"All 1\"" w750 {
          tunnel: [u16[] [1] ("References") u16[] [0] ("References")] -> w751
          frame "All 1" {
          }
          frame "Disable", Default {
          }
        }
        n352 = Unbundle By Name(w755) -> ("AI"=w756:T57)
        n353 = for {
          tunnel: w756 -> [w767] mode=indexing
          tunnel: [w766] -> w754 mode=indexing
          tunnel: w751 -> [w765]
          n354 = Bundle By Name(cluster=w767, "References"=w765) -> (w766:T58)
        }
        n355 = Bundle By Name(cluster=w755, "AI"=w754) -> (w753:refnum<class "Instrument.Lockin.lvclass">)
        n356 = property on="AI Channels" class="Arr (strict)"(error in=w752, "Val(Sgnl)"=w754) -> (error out=w757:errorcluster)  [unwired: 1 in, 1 out]
        n357 = Bundle By Name(cluster=w758, "Lockin"=w753) -> (w759:T36)
        n358 = call <vilib>:"Add State(s) to Queue__jki_lib_state_machine.vi"("State(s) in (\"\")"=w762) -> ("States Out"=w761:string)  [unwired: 14 in]
      }
      frame "UI: Initialize Gains" {
        n359 = Unbundle By Name(w778) -> ("Lockin"=w777:refnum<class "Instrument.Lockin.lvclass">)
        n360 = call "Initialize Input Gain.vi"("error in (no error)"=w776, "Instrument.DAQ"=w777) -> ("error out"=w774:errorcluster, "Input Gain"=w772:T48, "Instrument.DAQ out"=w775:refnum<class "Instrument.DAQ.lvclass">)  [unwired: 7 in]
        n361 = property on="Input Gain" class="Arr (strict)"(error in=w774, "Val(Sgnl)"=w772) -> (error out=w773:errorcluster)  [unwired: 1 in, 1 out]
        n362 = call "Initialize Ouput Gain.vi"("error in (no error)"=w773, "Instrument.DAQ"=w775) -> ("error out"=w769:errorcluster, "Output Gain"=w771:T48, "Instrument.DAQ out"=w770:refnum<class "Instrument.DAQ.lvclass">)  [unwired: 7 in]
        n363 = property on="Output Gain" class="Arr (strict)"(error in=w769, "Val(Sgnl)"=w771) -> (error out=w768:errorcluster)  [unwired: 1 in, 1 out]
        n364 = Bundle By Name(cluster=w778, "Lockin"=w770) -> (w779:T36)
        n365 = call <vilib>:"Add State(s) to Queue__jki_lib_state_machine.vi"("State(s) in (\"\")"=w782) -> ("States Out"=w781:string)  [unwired: 14 in]
      }
      frame "UI: Update Rings" {
        # "update Sweep Channel ring"
        n366 = Unbundle By Name(w796) -> ("Lockin"=w795:refnum<class "Instrument.Lockin.lvclass">)
        n367 = disable-structure shown="Enabled" {
          frame Disabled {
            n368 = call "Get AI REF (f) StringsAndValues.vi"() -> ("error out"=w803:errorcluster, "AI REF (f) StringsAndValues"=w802:cluster{string, i32}[], 3:w801)  [unwired: 9 in]
            n369 = property on="Channel" class="Ring (strict)"(error in=w803, "StringsAndValues[]"=w802) -> ()  [unwired: 1 in, 2 out]
          }
          frame Enabled {
          }
        }
        n370 = call "Get AO StringsAndValues.vi"("error in (no error)"=w794, "Configuration.DAQ"=w795) -> ("error out"=w792:errorcluster, "AO Strings and Values"=w793:cluster{string, i32}[], 3:w790)  [unwired: 7 in]
        n371 = property on="Channel" class="Ring (strict)"(error in=w792, "StringsAndValues[]"=w793) -> (error out=w789:errorcluster)  [unwired: 1 in, 1 out]
        n372 = call "Get REF StringsAndValues.vi"("error in (no error)"=w789, "Channels.REF"=w790) -> ("error out"=w791:errorcluster, "REF Strings and Values"=w788:cluster{string, i32}[], 3:w787)  [unwired: 7 in]
        n373 = property on="Reference" class="Ring (strict)"(error in=w791, "StringsAndValues[]"=w788) -> (error out=w785:errorcluster)  [unwired: 1 in, 1 out]
        n374 = call "Remove Unused References.vi"("error in (no error)"=w785, "Channels.AI"=w787) -> ("error out"=w784:errorcluster, 2:w783, "Channels.AI out"=w786:T57)  [unwired: 7 in]
        n375 = Bundle By Name(cluster=w796, "Lockin"=w786) -> (w797:T36)
        n376 = local write "AI Channels"(w783) -> ()
        n377 = call <vilib>:"Add State(s) to Queue__jki_lib_state_machine.vi"("State(s) in (\"\")"=w800) -> ("States Out"=w799:string)  [unwired: 14 in]
      }
      frame "UI: Update Plot Names" {
        n378 = Unbundle By Name(w807) -> ("Lockin"=w812:refnum<class "Instrument.Lockin.lvclass">)
        n379 = call "Get AO StringsAndValues.vi"("error in (no error)"=w804, "Configuration.DAQ"=w812) -> ("error out"=w814:errorcluster, "AO Strings and Values"=w809:cluster{string, i32}[])  [unwired: 8 in]
        n380 = call "Get AI StringsAndValues.vi"("error in (no error)"=w804, "Configuration.DAQ"=w812) -> ("error out"=w815:errorcluster, "AI StringsAndValues"=w816:cluster{string, i32}[])  [unwired: 8 in]
        n381 = call "Get AI REF StringsAndValues.vi"("error in (no error)"=w804, "Channels.REF"=w812) -> ("error out"=w805:errorcluster, "REF StringsAndValues"=w806:cluster{string, i32}[])  [unwired: 8 in]
        n382 = for {
          tunnel: w809 -> [w833] mode=indexing
          tunnel: w814 -> [w834]
          tunnel: [w831] -> w813
          i -> [w835]
          n383 = control-ref of="Sweep Results AO"() -> (w832:refnum<vi>)
          n384 = Unbundle(w833) -> (w836:string)  [unwired: 1 out]
          n385 = call-poly "Set Legend.vi"("error in (no error)"=w834, "Plot.Plot Name"=w836, "Active Plot"=w835, "WFGraph in"=w832) -> ("error out"=w831:errorcluster)  [unwired: 4 in, 3 out]
        }
        n386 = for {
          tunnel: w816 -> [w846] mode=indexing
          tunnel: w815 -> [w847]
          tunnel: [w841] -> w818
          i -> [w848]
          n387 = control-ref of="AI Graph"() -> (w849:refnum<vi>)
          n388 = Unbundle(w846) -> (w850:string)  [unwired: 1 out]
          n389 = control-ref of="Sweep Results AI"() -> (w837:refnum<vi>)
          n390 = call-poly "Set Legend.vi"("error in (no error)"=w847, "Plot.Plot Name"=w850, "Active Plot"=w848, "WFGraph in"=w849) -> ("error out"=w845:errorcluster, "Plot.Plot Name"=w844:string, "Active Plot"=w843:i32)  [unwired: 4 in, 1 out]
          n391 = call-poly "Set Legend.vi"("error in (no error)"=w845, "Plot.Plot Name"=w844, "Active Plot"=w843, "WFGraph in"=w837) -> ("error out"=w842:errorcluster, "Plot.Plot Name"=w840:string, "Active Plot"=w839:i32)  [unwired: 4 in, 1 out]
          n392 = control-ref of="PS WFGraph"() -> (w838:refnum<vi>)
          n393 = call-poly "Set Legend.vi"("error in (no error)"=w842, "Plot.Plot Name"=w840, "Active Plot"=w839, "WFGraph (WDT) in"=w838) -> ("error out"=w841:errorcluster)  [unwired: 4 in, 3 out]
          n394 = call-poly "Set Legend.vi"("WFGraph (WDT) in"=w838) -> ()  [unwired: 7 in, 4 out]
          n395 = call-poly "Set Legend.vi"("WFGraph in"=w837) -> ()  [unwired: 7 in, 4 out]
        }
        n396 = local read "Y Axis (Output)"() -> (w808:enum16{"Analog Output", "Reference"})
        n397 = case shown="\"Analog Output\", Default" w808 {
          tunnel: [w822 w824] -> w811
          tunnel: w806 -> [_ w823]
          tunnel: w809 -> [w822 _]
          frame "Analog Output", Default {
          }
          frame "Reference" {
            n398 = Interleave 1D Arrays(w823, w823) -> (w824:cluster{string, i32}[])
          }
        }
        n399 = for {
          tunnel: w811 -> [w829] mode=indexing
          tunnel: w805 -> [w827]
          tunnel: [w826] -> w810
          i -> [w828]
          n400 = Unbundle(w829) -> (w825:string)  [unwired: 1 out]
          n401 = control-ref of="AO Graph"() -> (w830:refnum<vi>)
          n402 = call-poly "Set Legend.vi"("error in (no error)"=w827, "Plot.Plot Name"=w825, "Active Plot"=w828, "WFGraph in"=w830) -> ("error out"=w826:errorcluster)  [unwired: 4 in, 3 out]
        }
        n403 = call <vilib>:"Add State(s) to Queue__jki_lib_state_machine.vi"("State(s) in (\"\")"=w821) -> ("States Out"=w820:string)  [unwired: 14 in]
        n404 = Merge Errors(w813, w818, w810, w804) -> (w817:errorcluster)
      }
      frame "UI: Sync Lockin Plot Visibility" {
        # "#todo"
        # "#done"
        # "number of results"
        # "Do not put any code in this frame.\n(It is a separator no-op. You can make a copy of this frame to create a new UI frame)"
        n405 = local read "Results Plot Names"() -> (w853:string[])
        n406 = Array Size(array=w853) -> (size(s)=w854:i32)
        n407 = feedback #1() -> (w856:string[])  [unwired: 1 in]
        n408 = feedback-in #1(w853) -> ()
        n409 = Not Equal?(x=w856, y=w853) -> (x != y?=w858:bool)
        n410 = First Call?() -> (First Call?: T/F=w859:bool)
        n411 = Or(x=w859, y=w858) -> (x .or. y?=w857:bool)
        n412 = case shown="True" w857 {
          tunnel: w852 -> [w881 w885]
          tunnel: w853 -> [_ w886]
          tunnel: [w881 w882] -> w855
          frame False {
          }
          frame True {
            n413 = for {
              tunnel: w885 -> [w907]
              tunnel: [w892] -> w883
              tunnel: w886 -> [w887] mode=indexing
              i -> [w902]
              n414 = control-ref of="XY Graph"() -> (w897:refnum<vi>)
              n415 = control-ref of="Lockin 2"() -> (w898:refnum<vi>)
              n416 = control-ref of="Lockin 1"() -> (w899:refnum<vi>)
              n417 = call-poly "Set Legend.vi"("error in (no error)"=w907, "Plot.Plot Name"=w887, "Active Plot"=w902, "WaveformChart in"=w899) -> ("error out"=w903:errorcluster, "Plot.Plot Name"=w901:string, "Active Plot"=w906:i32)  [unwired: 4 in, 1 out]
              n418 = control-ref of="Sweep Results Y"() -> (w895:refnum<vi>)
              n419 = control-ref of="Sweep Results X"() -> (w896:refnum<vi>)
              n420 = call-poly "Set Legend.vi"("error in (no error)"=w903, "Plot.Plot Name"=w901, "Active Plot"=w906, "WaveformChart in"=w898) -> ("error out"=w904:errorcluster, "Plot.Plot Name"=w900:string, "Active Plot"=w905:i32)  [unwired: 4 in, 1 out]
              n421 = call "Set Legend (XYGraph).vi"("error in (no error)"=w904, "Plot.Plot Name"=w900, "Active Plot"=w905, "XYGraph in"=w897) -> ("error out"=w894:errorcluster, "Plot.Plot Name"=w888:string, "Active Plot"=w891:i32)  [unwired: 4 in, 1 out]
              n422 = call-poly "Set Legend.vi"("error in (no error)"=w894, "Plot.Plot Name"=w888, "Active Plot"=w891, "WFGraph in"=w896) -> ("error out"=w893:errorcluster, "Plot.Plot Name"=w889:string, "Active Plot"=w890:i32)  [unwired: 4 in, 1 out]
              n423 = call-poly "Set Legend.vi"("error in (no error)"=w893, "Plot.Plot Name"=w889, "Active Plot"=w890, "WFGraph in"=w895) -> ("error out"=w892:errorcluster)  [unwired: 4 in, 3 out]
            }
            n424 = property on="Channel" class="Ring (strict)"(error in=w885, "Strings []"=w886) -> (error out=w884:errorcluster)  [unwired: 1 in, 1 out]
            n425 = Merge Errors(w884, w883) -> (w882:errorcluster)
          }
        }
        n426 = for {
          N: w854 -> [_]
          tunnel: w855 -> [w870]
          tunnel: [w865] -> w851
          i -> [w879]
          n427 = control-ref of="Lockin 1"() -> (w880:refnum<vi>)
          n428 = call "Get Plot Visibility (WFChart).vi"("error in (no error)"=w870, "ActPlot"=w879, "WaveformChart in"=w880) -> ("error out"=w869:errorcluster, "Plot.Visible?"=w864:bool, "Active Plot"=w874:i32)  [unwired: 6 in]
          n429 = control-ref of="Lockin 2"() -> (w878:refnum<vi>)
          n430 = call-poly "Set Plot Visibility.vi"("error in (no error)"=w869, "Plot.Visible?"=w864, "ActPlot"=w874, "WaveformChart in"=w878) -> ("error out"=w868:errorcluster, "Active Plot"=w873:i32)  [unwired: 6 in]
          n431 = control-ref of="XY Graph"() -> (w877:refnum<vi>)
          n432 = call-poly "Set Plot Visibility.vi"("error in (no error)"=w868, "Plot.Visible?"=w864, "ActPlot"=w873, "XYGraph in"=w877) -> ("error out"=w867:errorcluster, "Active Plot"=w872:i32)  [unwired: 6 in]
          n433 = control-ref of="Sweep Results Y"() -> (w876:refnum<vi>)
          n434 = control-ref of="Sweep Results X"() -> (w875:refnum<vi>)
          n435 = call-poly "Set Plot Visibility.vi"("error in (no error)"=w867, "Plot.Visible?"=w864, "ActPlot"=w872, "WFGraph in"=w876) -> ("error out"=w866:errorcluster, "Active Plot"=w871:i32)  [unwired: 6 in]
          n436 = call-poly "Set Plot Visibility.vi"("error in (no error)"=w866, "Plot.Visible?"=w864, "ActPlot"=w871, "WFGraph in"=w875) -> ("error out"=w865:errorcluster)  [unwired: 6 in, 1 out]
        }
        n437 = call <vilib>:"Add State(s) to Queue__jki_lib_state_machine.vi"("State(s) in (\"\")"=w863) -> ("States Out"=w862:string)  [unwired: 14 in]
      }
      frame "UI: Sync AO AI Plot Visibility" {
        # "#done"
        # "Do not put any code in this frame.\n(It is a separator no-op. You can make a copy of this frame to create a new UI frame)"
        n438 = Unbundle By Name(w914) -> ("Lockin"=w912:refnum<class "Instrument.Lockin.lvclass">)
        n439 = call "Get AO StringsAndValues.vi"("error in (no error)"=w910, "Configuration.DAQ"=w912) -> ("error out"=w908:errorcluster, "AO Strings and Values"=w911:cluster{string, i32}[])  [unwired: 8 in]
        n440 = call "Get AI StringsAndValues.vi"("error in (no error)"=w910, "Configuration.DAQ"=w912) -> ("error out"=w909:errorcluster, "AI StringsAndValues"=w913:cluster{string, i32}[])  [unwired: 8 in]
        n441 = for {
          tunnel: w909 -> [w934]
          tunnel: [w930] -> w916
          tunnel: w913 -> [_] mode=indexing
          i -> [w937]
          n442 = control-ref of="AI Graph"() -> (w933:refnum<vi>)
          n443 = property on="Property Node" class="WFGraph (strict)"(reference=w933, error in=w934, "Active Plot"=w937) -> (error out=w938:errorcluster, "Plot.Visible?"=w936:bool)  [unwired: 1 out]
          n444 = control-ref of="Sweep Results AI"() -> (w935:refnum<vi>)
          n445 = property on="Property Node" class="WFGraph (strict)"(reference=w935, error in=w938, "Active Plot"=w937, "Plot.Visible?"=w936) -> (error out=w931:errorcluster)  [unwired: 1 out]
          n446 = call <vilib>:"Clear Errors.vi"("error in (no error)"=w931, "specific error code to clear (0: all)"=1077) -> ("error out"=w930:errorcluster)  [unwired: 4 in, 1 out]
        }
        n447 = for {
          tunnel: w908 -> [w924]
          tunnel: [w921] -> w917
          tunnel: w911 -> [_] mode=indexing
          i -> [w928]
          n448 = control-ref of="AO Graph"() -> (w925:refnum<vi>)
          n449 = property on="Property Node" class="WFGraph (strict)"(reference=w925, error in=w924, "Active Plot"=w928) -> (error out=w929:errorcluster, "Plot.Visible?"=w927:bool)  [unwired: 1 out]
          n450 = control-ref of="Sweep Results AO"() -> (w926:refnum<vi>)
          n451 = property on="Property Node" class="WFGraph (strict)"(reference=w926, error in=w929, "Active Plot"=w928, "Plot.Visible?"=w927) -> (error out=w922:errorcluster)  [unwired: 1 out]
          n452 = call <vilib>:"Clear Errors.vi"("error in (no error)"=w922, "specific error code to clear (0: all)"=1077) -> ("error out"=w921:errorcluster)  [unwired: 4 in, 1 out]
        }
        n453 = Merge Errors(w916, w917) -> (w915:errorcluster)
        n454 = call <vilib>:"Add State(s) to Queue__jki_lib_state_machine.vi"("State(s) in (\"\")"=w920) -> ("States Out"=w919:string)  [unwired: 14 in]
      }
      frame "UI: Disable Buttons" {
        # "#done"
        n455 = control-ref of="Start"() -> (w944:refnum<vi>)
        n456 = control-ref of="Pause"() -> (w943:refnum<vi>)
        n457 = control-ref of="Trigger"() -> (w942:refnum<vi>)
        n458 = control-ref of="Reset"() -> (w941:refnum<vi>)
        n459 = control-ref of="Help"() -> (w940:refnum<vi>)
        n460 = Build Array(w944, w943, w942, w941, w940) -> (w939:refnum<vi>[])
        n461 = for {
          tunnel: w939 -> [w951] mode=indexing
          n462 = property class="Bool (strict)"(reference=w951, "DisabledEnum"=T27."Disabled and Grayed Out" ("Disabled")) -> ()  [unwired: 1 in, 2 out]
        }
        n463 = call <vilib>:"Add State(s) to Queue__jki_lib_state_machine.vi"("State(s) in (\"\")"=w949) -> ("States Out"=w948:string)  [unwired: 14 in]
      }
      frame "UI: Enable Buttons" {
        # "#done"
        n464 = control-ref of="Start"() -> (w957:refnum<vi>)
        n465 = control-ref of="Pause"() -> (w956:refnum<vi>)
        n466 = control-ref of="Trigger"() -> (w955:refnum<vi>)
        n467 = control-ref of="Reset"() -> (w954:refnum<vi>)
        n468 = control-ref of="Help"() -> (w953:refnum<vi>)
        n469 = Build Array(w957, w956, w955, w954, w953) -> (w952:refnum<vi>[])
        n470 = for {
          tunnel: w952 -> [w964] mode=indexing
          n471 = property class="Bool (strict)"(reference=w964, "DisabledEnum"=T27."Enabled" ("Disabled")) -> ()  [unwired: 1 in, 2 out]
        }
        n472 = call <vilib>:"Add State(s) to Queue__jki_lib_state_machine.vi"("State(s) in (\"\")"=w962) -> ("States Out"=w961:string)  [unwired: 14 in]
      }
      frame "UI: AI Graph Plot Visible" {
        # "#done"
        # "Do not put any code in this frame.\n(It is a separator no-op. You can make a copy of this frame to create a new UI frame)"
        n473 = case shown="\"None\", Default" w970 {
          tunnel: [FALSE TRUE] -> w967
          frame "None", Default {
          }
          frame "ALL" {
          }
        }
        n474 = control-ref of="AI Graph"() -> (w971:refnum<vi>)
        n475 = control-ref of="Sweep Results AI"() -> (w968:refnum<vi>)
        n476 = call-poly "Set All Plot Visibility.vi"("error in (no error)"=w969, "All Visible?"=w967, "WFGraph in"=w971) -> ("error out"=w966:errorcluster)  [unwired: 7 in, 1 out]
        n477 = call-poly "Set All Plot Visibility.vi"("error in (no error)"=w966, "All Visible?"=w967, "WFGraph in"=w968) -> ("error out"=w965:errorcluster)  [unwired: 7 in, 1 out]
        n478 = call <vilib>:"Add State(s) to Queue__jki_lib_state_machine.vi"("State(s) in (\"\")"=w975) -> ("States Out"=w974:string)  [unwired: 14 in]
      }
      frame "UI: AO Graph Plot Visible" {
        # "#done"
        # "Do not put any code in this frame.\n(It is a separator no-op. You can make a copy of this frame to create a new UI frame)"
        n479 = case shown="\"ALL\"" w984 {
          tunnel: [FALSE TRUE] -> w980
          frame "None", Default {
          }
          frame "ALL" {
          }
        }
        n480 = control-ref of="AO Graph"() -> (w982:refnum<vi>)
        n481 = call-poly "Set All Plot Visibility.vi"("error in (no error)"=w983, "All Visible?"=w980, "WFGraph in"=w982) -> ("error out"=w979:errorcluster)  [unwired: 7 in, 1 out]
        n482 = control-ref of="Sweep Results AO"() -> (w981:refnum<vi>)
        n483 = call-poly "Set All Plot Visibility.vi"("error in (no error)"=w979, "All Visible?"=w980, "WFGraph in"=w981) -> ("error out"=w978:errorcluster)  [unwired: 7 in, 1 out]
        n484 = call <vilib>:"Add State(s) to Queue__jki_lib_state_machine.vi"("State(s) in (\"\")"=w988) -> ("States Out"=w987:string)  [unwired: 14 in]
      }
      frame "UI: Lockin 1 Plot Visible" {
        # "#done"
        # "Do not put any code in this frame.\n(It is a separator no-op. You can make a copy of this frame to create a new UI frame)"
        n485 = case shown="\"ALL\"" w1003 {
          tunnel: [FALSE TRUE] -> w999
          frame "None", Default {
          }
          frame "ALL" {
          }
        }
        n486 = control-ref of="Lockin 1"() -> (w1002:refnum<vi>)
        n487 = control-ref of="Lockin 2"() -> (w1000:refnum<vi>)
        n488 = control-ref of="Sweep Results X"() -> (w998:refnum<vi>)
        n489 = control-ref of="Sweep Results Y"() -> (w997:refnum<vi>)
        n490 = call-poly "Set All Plot Visibility.vi"("error in (no error)"=w1001, "All Visible?"=w999, "WaveformChart in"=w1002) -> ("error out"=w995:errorcluster)  [unwired: 7 in, 1 out]
        n491 = call-poly "Set All Plot Visibility.vi"("error in (no error)"=w995, "All Visible?"=w999, "WaveformChart in"=w1000) -> ("error out"=w994:errorcluster)  [unwired: 7 in, 1 out]
        n492 = call-poly "Set All Plot Visibility.vi"("error in (no error)"=w994, "All Visible?"=w999, "WFGraph in"=w998) -> ("error out"=w993:errorcluster)  [unwired: 7 in, 1 out]
        n493 = control-ref of="XY Graph"() -> (w996:refnum<vi>)
        n494 = call-poly "Set All Plot Visibility.vi"("error in (no error)"=w993, "All Visible?"=w999, "WFGraph in"=w997) -> ("error out"=w992:errorcluster)  [unwired: 7 in, 1 out]
        n495 = call-poly "Set All Plot Visibility.vi"("error in (no error)"=w992, "All Visible?"=w999, "XYGraph in"=w996) -> ("error out"=w991:errorcluster)  [unwired: 7 in, 1 out]
        n496 = call <vilib>:"Add State(s) to Queue__jki_lib_state_machine.vi"("State(s) in (\"\")"=w1007) -> ("States Out"=w1006:string)  [unwired: 14 in]
      }
      frame "UI: Update Waveform Graphs" {
        # "#todo\nshould be owned by Lockin UI"
        # "private"
        # "private"
        n497 = Unbundle By Name(w1028) -> ("Lockin"=w1021:refnum<class "Instrument.Lockin.lvclass">)
        n498 = Unbundle By Name(w1021) -> ("AI.Gain"=w1017:T48, "AI"=w1031:waveform(dbl)[], "AO"=w1011:waveform(dbl)[], "RefX"=w1013:waveform(dbl)[], "RefY"=w1012:waveform(dbl)[])
        n499 = local read "Y Axis (Output)"() -> (w1014:enum16{"Analog Output", "Reference"})
        n500 = Interleave 1D Arrays(w1013, w1012) -> (w1010:waveform(dbl)[])
        n501 = case shown="\"Analog Output\", Default" w1014 {
          tunnel: w1011 -> [w1039 _]
          tunnel: w1010 -> [_ w1040]
          tunnel: [w1039 w1040] -> w1022
          frame "Analog Output", Default {
          }
          frame "Reference" {
          }
        }
        n502 = local read "X Axis"() -> (w1019:enum16{"Time", "Samples"})
        n503 = Power Of 10(x="Decimate") -> (10^x=w1023:dbl)
        n504 = call "Display n or dt.vi"("error in (no error)"=w1020, "X Axis"=w1019, "Input Waveforms"=w1031) -> ("error out"=w1030:errorcluster, "Output Waveforms"=w1018:waveform(dbl)[])  [unwired: 7 in]
        n505 = call "Display n or dt.vi"("error in (no error)"=w1020, "X Axis"=w1019, "Input Waveforms"=w1022) -> ("error out"=w1029:errorcluster, "Output Waveforms"=w1034:waveform(dbl)[])  [unwired: 7 in]
        n506 = call "Decimate Waveforms.vi"("WFM"=w1034, "averaging"=FALSE, "decimating factor"=w1023, "error in (no error)"=w1029) -> ("WFM out"=→"AO Graph":waveform(dbl)[])  [unwired: 5 in, 1 out]
        n507 = call "Decimate Waveforms.vi"("WFM"=w1018, "averaging"=FALSE, "decimating factor"=w1023, "error in (no error)"=w1030) -> ("WFM out"=w1027:waveform(dbl)[], "error out"=w1025:errorcluster)  [unwired: 5 in]
        n508 = case shown="\"ADC\"" "Y Axis (Input)" {
          tunnel: w1027 -> [w1042 w1047]
          tunnel: w1017 -> [_ w1045]
          tunnel: [w1042 w1046] -> w1026
          tunnel: w1025 -> [w1041 w1044]
          tunnel: [w1041 w1043] -> w1016
          frame "Device", Default {
          }
          frame "ADC" {
            n509 = call "Multiply by Gain.vi"("error in (no error)"=w1044, "Gain"=w1045, "WFM in"=w1047) -> ("error out"=w1043:errorcluster, "WFM out"=w1046:waveform(dbl)[])  [unwired: 7 in]
          }
        }
        "AI Graph" <- w1026
        n510 = call <vilib>:"Add State(s) to Queue__jki_lib_state_machine.vi"("State(s) in (\"\")"=w1038) -> ("States Out"=w1037:string)  [unwired: 14 in]
      }
      frame "UI: Update Lockin Graphs" {
        # "#todo\nshould be owned by Lockin UI"
        # "#todo\nshould be owned by Lockin UI"
        # "#todo\nshould be owned by Lockin UI"
        n511 = Unbundle By Name(w1065) -> ("Lockin"=w1055:refnum<class "Instrument.Lockin.lvclass">)
        n512 = call "Parse Results (table).vi"("error in (no error)"=w1060, "Results (Dictionary)"=w1055) -> ("error out"=w1059:errorcluster, 1:→"Results", "Table"=w1054:string[][])  [unwired: 6 in, 1 out]
        n513 = call "Dictionary to Chart.vi"("error in (no error)"=w1059, "Display"="Display", "Results (Dictionary)"=w1054) -> ("error out"=w1061:errorcluster, "Y/Theta Array"=→"XY Graph":waveform(dbl)[], "X/R Array"=→"Lockin 2":waveform(dbl)[], "Results (Dictionary) out"=→"Lockin 1":cluster{"key":string, "value":dbl}[], "Plot Names"=→"Results Plot Names":string[])  [unwired: 4 in]
        n514 = call "Dictionary to Indicator.vi"("Results (Dictionary)"=w1054, "AI Channel"="Channel", "error in (no error)"=w1061) -> ("X"=→"X":dbl, "Y"=→"Y":dbl, "R"=→"R":dbl, "Theta"=→"Theta":dbl, "error out"=w1053:errorcluster)  [unwired: 8 in]
        n515 = call <vilib>:"Add State(s) to Queue__jki_lib_state_machine.vi"("State(s) in (\"\")"=w1068) -> ("States Out"=w1067:string)  [unwired: 14 in]
      }
      frame "UI: Update Waveform Graph Labels" {
        n516 = control-ref of="AI Graph"() -> (w1073:refnum<vi>)
        n517 = control-ref of="AO Graph"() -> (w1070:refnum<vi>)
        n518 = call "Set AO AI Graph X Axis (WFGraph).vi"("error in (no error)"=w1075, "X Axis"="X Axis", "WaveformGraph in"=w1073) -> ("error out"=w1077:errorcluster)  [unwired: 8 in]
        n519 = call "Set AO AI Graph X Axis (WFGraph).vi"("error in (no error)"=w1077, "X Axis"="X Axis", "WaveformGraph in"=w1070) -> ("error out"=w1076:errorcluster)  [unwired: 8 in]
        n520 = control-ref of="AO Graph"() -> (w1071:refnum<vi>)
        n521 = call "Set AO Graph Y Axis (WFGraph).vi"("error in (no error)"=w1076, "Y Axis (Output)"="Y Axis (Output)", "WaveformGraph in"=w1071) -> ("error out"=w1074:errorcluster)  [unwired: 8 in]
        n522 = call <vilib>:"Add State(s) to Queue__jki_lib_state_machine.vi"("State(s) in (\"\")"=w1081) -> ("States Out"=w1080:string)  [unwired: 14 in]
      }
      frame "UI: Update Lockin Graph Range" {
        n523 = Negate(x="Numeric") -> (-x=w1084:dbl)
        n524 = Negate(x="X/R Range") -> (-x=w1086:dbl)
        n525 = Negate(x="Y/Theta Range") -> (-x=w1087:dbl)
        n526 = property on="Lockin 1" class="WFChart (strict)"("YScale.Maximum"="X/R Range", "YScale.Minimum"=w1086) -> ()  [unwired: 2 in, 2 out]
        n527 = property on="Lockin 2" class="WFChart (strict)"("YScale.Maximum"="Y/Theta Range", "YScale.Minimum"=w1087) -> ()  [unwired: 2 in, 2 out]
        n528 = property on="XY Graph" class="XYGraph (strict)"("XScale.Maximum"="Numeric", "XScale.Minimum"=w1084, "YScale.Maximum"="Numeric", "YScale.Minimum"=w1084) -> ()  [unwired: 2 in, 2 out]
        n529 = call <vilib>:"Add State(s) to Queue__jki_lib_state_machine.vi"("State(s) in (\"\")"=w1092) -> ("States Out"=w1091:string)  [unwired: 14 in]
      }
      frame "UI: Update Displays" {
        n530 = local read "Display"() -> (w1095:T19)
        n531 = case shown="\"R and Theta\"" w1095 {
          tunnel: ["X (V)" "R (V)"] -> _
          tunnel: ["Y (V)" "Theta (°)"] -> _
          tunnel: ["Lockin X (V)" "R (V)"] -> w1094
          tunnel: ["Lockin Y (V)" "Theta (°)"] -> w1093
          frame "X and Y", Default {
          }
          frame "R and Theta" {
          }
        }
        n532 = property on="Lockin 1" class="WFChart (strict)"("YScale.NameLbl.Text"=w1094) -> ()  [unwired: 2 in, 2 out]
        n533 = property on="Lockin 2" class="WFChart (strict)"("YScale.NameLbl.Text"=w1093) -> ()  [unwired: 2 in, 2 out]
        n534 = call <vilib>:"Add State(s) to Queue__jki_lib_state_machine.vi"("State(s) in (\"\")"=w1100) -> ("States Out"=w1099:string)  [unwired: 14 in]
      }
      frame "UI: Update Sweep Results Graphs" {
        n535 = Unbundle By Name(w1112) -> ("Lockin"=w1111:refnum<class "Instrument.Lockin.lvclass">)
        n536 = Unbundle By Name(w1111) -> ("Sweep Results X"=→"Sweep Results X":waveform(dbl)[], "Sweep Results Y"=→"Sweep Results Y":waveform(dbl)[])
        n537 = call <vilib>:"Add State(s) to Queue__jki_lib_state_machine.vi"("State(s) in (\"\")"=w1116) -> ("States Out"=w1115:string)  [unwired: 14 in]
      }
      frame "UI: Update Sweep WFMs Graphs" {
        n538 = Unbundle By Name(w1119) -> ("SweepWaveforms.Sweep AO"=→"Sweep Results AO":waveform(dbl)[], "SweepWaveforms.Sweep AI"=→"Sweep Results AI":waveform(dbl)[])
        n539 = call <vilib>:"Add State(s) to Queue__jki_lib_state_machine.vi"("State(s) in (\"\")"=w1123) -> ("States Out"=w1122:string)  [unwired: 14 in]
      }
      frame "UI: Update Status" {
        n540 = Unbundle By Name(w1126) -> ("Lockin"=w1125:refnum<class "Instrument.Lockin.lvclass">)
        n541 = Unbundle By Name(w1125) -> ("DAQ state"=w1124:T32)
        n542 = case shown="\"idle\", Default" w1124 {
          tunnel: ["Idle" ("Status") "Started" ("Status") "Stopped" ("Status") "Running" ("Status") "Sweeping" ("Status")] -> w1127
          frame "idle", Default {
            w1133 = FALSE ("Trigger")
            n543 = local write "Reset"(w1133) -> ()
            n544 = local write "Trigger"(w1133) -> ()
            n545 = local write "Start"(w1133) -> ()
          }
          frame "started" {
            w1134 = FALSE ("Trigger")
            n546 = local write "Start Sweep"(w1134) -> ()
            n547 = local write "Reset"(w1134) -> ()
            n548 = local write "Stop Sweep"(w1134) -> ()
            n549 = disable-structure shown="Disabled" {
              frame Disabled {
                n550 = local read "Trigger"() -> ()  [unwired: 1 in]
              }
              frame Enabled {
              }
            }
            n551 = local write "Start"(TRUE ("Trigger")) -> ()
          }
          frame "stopped" {
            w1139 = FALSE ("Trigger")
            n552 = local write "Reset"(w1139) -> ()
            n553 = local write "Trigger"(w1139) -> ()
            n554 = local write "Start"(FALSE ("Trigger")) -> ()
          }
          frame "created" {
            n555 = local write "Start"(TRUE ("Start")) -> ()
            n556 = local write "Reset"(FALSE ("Reset")) -> ()
          }
          frame "sweeping" {
            n557 = call <userlib>:"MGI Milliseconds Since Last Reset.vi"("Reset (F)"=TRUE) -> ()  [unwired: 5 in, 2 out]
          }
        }
        n558 = local write "Status"(w1127) -> ()
        n559 = call <vilib>:"Add State(s) to Queue__jki_lib_state_machine.vi"("State(s) in (\"\")"=w1131) -> ("States Out"=w1130:string)  [unwired: 14 in]
      }
      frame "UI: Update Sweep Timer" {
        n560 = local read "Status"() -> (w1146:string)
        n561 = case shown="\"Sweeping\"" w1146 {
          tunnel: [0.0 w1154] -> w1145
          frame Default {
          }
          frame "Sweeping" {
            # "some overhead"
            n562 = call <userlib>:"MGI Milliseconds Since Last Reset.vi"() -> ("ms"=w1160:u32)  [unwired: 6 in, 1 out]
            n563 = local read "Sweep Time (s)"() -> (w1156:dbl)
            n564 = local read "Initial Wait (s)"() -> (w1157:dbl)
            n565 = Divide(x=w1160, y=u32 1000) -> (x/y=w1158:dbl)
            n566 = Negate(x=w1158) -> (-x=w1155:dbl)
            n567 = Compound Arithmetic op=ADD(2.0 ("value"), w1157, w1156, w1155) -> (w1154:dbl)
          }
        }
        "Sweep Timer (s)" <- w1145
        n568 = call <vilib>:"Add State(s) to Queue__jki_lib_state_machine.vi"("State(s) in (\"\")"=w1151) -> ("States Out"=w1150:string)  [unwired: 14 in]
      }
      frame "UI: Defer Panel Updates" {
        n569 = case shown="\"True\"" w1162 {
          tunnel: [FALSE ("Defer Updates?") TRUE ("Defer Updates?")] -> w1161
          frame "False", Default {
          }
          frame "True" {
          }
        }
        n570 = call <userlib>:"MGI Defer Panel Updates.vi"("Error In"=w1164, "Defer Updates?"=w1161) -> ("Error Out"=w1163:errorcluster)  [unwired: 9 in]
        n571 = call <vilib>:"Add State(s) to Queue__jki_lib_state_machine.vi"("State(s) in (\"\")"=w1168) -> ("States Out"=w1167:string)  [unwired: 14 in]
      }
      frame "UI: Cursor Set" {
        # "Argument"
        # "Set and Unset Cursor Busy.\n(Usage: \"UI: Cursor Set >> Busy|Idle\")"
        n572 = case shown="\"Busy\"" w1175 {
          tunnel: w1172 -> [w1179 w1181]
          tunnel: [w1178 w1180] -> w1171
          frame "Idle", Default {
            n573 = call <vilib>:"Unset Busy.vi"("error in (no error)"=w1179) -> ("error out"=w1178:errorcluster)  [unwired: 10 in]
          }
          frame "Busy" {
            n574 = call <vilib>:"Set Busy.vi"("error in (no error)"=w1181) -> ("error out"=w1180:errorcluster)  [unwired: 9 in, 1 out]
          }
        }
        n575 = call <vilib>:"Add State(s) to Queue__jki_lib_state_machine.vi"("State(s) in (\"\")"=w1177) -> ("States Out"=w1176:string)  [unwired: 14 in]
      }
      frame "UI: Front Panel State" {
        # "Argument"
        n576 = Unbundle By Name(w1184) -> ("Core.Current VI Reference"=w1186:refnum<vi>)
        n577 = case shown="\"Open\", Default" w1185 {
          tunnel: w1187 -> [w1193 w1206]
          tunnel: [w1195 w1207] -> w1183
          tunnel: w1186 -> [w1194 w1204]
          frame "Open", Default {
            n578 = property class="VI"(reference=w1194, error in=w1193) -> (reference out=w1191:refnum<vi>, error out=w1192:errorcluster, "Front Panel.Open"=w1190:bool)
            n579 = case shown="True" w1190 {
              tunnel: [w1198 w1201] -> w1195
              tunnel: w1192 -> [w1197 w1201]
              tunnel: w1191 -> [w1196 _]
              frame False {
                n580 = invoke class="VI" method="FP.Open"(reference=w1196, error in=w1197, "Activate"=TRUE, "State"=T28."Standard") -> (error out=w1198:errorcluster)  [unwired: 1 in, 4 out]
              }
              frame True {
              }
            }
          }
          frame "Close" {
            n581 = property class="VI"(reference=w1204, error in=w1206) -> (reference out=w1203:refnum<vi>, error out=w1205:errorcluster, "Front Panel.Open"=w1202:bool)
            n582 = case shown="True" w1202 {
              tunnel: [w1208 w1211] -> w1207
              tunnel: w1205 -> [w1208 w1210]
              tunnel: w1203 -> [_ w1209]
              frame False {
              }
              frame True {
                n583 = invoke class="VI" method="FP.Close"(reference=w1209, error in=w1210) -> (error out=w1211:errorcluster)  [unwired: 1 in, 2 out]
              }
            }
          }
        }
        n584 = call <vilib>:"Add State(s) to Queue__jki_lib_state_machine.vi"("State(s) in (\"\")"=w1189) -> ("States Out"=w1188:string)  [unwired: 14 in]
      }
      frame "UI: Cleanup" {
        w1213 = FALSE ("Close")
        w1212 = waveform(dbl)[] [] ("Signals Graph")
        w1215 = waveform(dbl)[][] [] ("History Data")
        # "Initialize the User Interface, here.\n(this is called automatically, by the Macro: Exit)"
        n585 = property on="Lockin 1" class="WFChart (strict)"("History Data"=w1215) -> ()  [unwired: 2 in, 2 out]
        n586 = local write "Sweep Results X"(w1212) -> ()
        n587 = local write "Sweep Results Y"(w1212) -> ()
        n588 = property on="AI Graph" class="WFGraph (strict)"("Value"=w1212) -> (error out=w1214:errorcluster)  [unwired: 2 in, 1 out]
        n589 = property on="Lockin 2" class="WFChart (strict)"("History Data"=w1215) -> ()  [unwired: 2 in, 2 out]
        n590 = property on="AO Graph" class="WFGraph (strict)"(error in=w1214, "Value"=w1212) -> ()  [unwired: 1 in, 2 out]
        n591 = local write "Self Calibrate"(w1213) -> ()
        n592 = local write "Trigger"(w1213) -> ()
        n593 = local write "Close"(w1213) -> ()
        n594 = local write "Pause"(w1213) -> ()
        n595 = local write "Reset"(w1213) -> ()
        n596 = local write "Start"(w1213) -> ()
        n597 = local write "Status"("Shutdown" ("Status")) -> ()
        n598 = call <vilib>:"Add State(s) to Queue__jki_lib_state_machine.vi"("State(s) in (\"\")"=w1221) -> ("States Out"=w1220:string)  [unwired: 14 in]
      }
      frame "---------- Macro ----------" {
        # "Do not put any code in this frame.\n(It is a separator no-op. You can make a copy of this frame to create a new Macro frame)"
        n599 = call <vilib>:"Add State(s) to Queue__jki_lib_state_machine.vi"("State(s) in (\"\")"=w1226) -> ("States Out"=w1225:string)  [unwired: 14 in]
      }
      frame "Macro: Initialize" {
        n600 = call <vilib>:"Add State(s) to Queue__jki_lib_state_machine.vi"("State(s) in Front (\"\")"="Data: Initialize\nInitialize Core Data\n\n\nEvents: Register\n\n\nUI: Front Panel State >> Open\n\n\nMacro: Initialize UI\nUI: Update Sweep WFMs Graphs\nUI: Disable Buttons\n\n\nMacro: Initialize DAQ SMO", "State(s) in (\"\")"=w1227) -> ("States Out"=w1232:string)  [unwired: 13 in]
      }
      frame "Macro: Initialize UI" {
        n601 = call <vilib>:"Add State(s) to Queue__jki_lib_state_machine.vi"("State(s) in Front (\"\")"="UI: Update AI Ch\nUI: Update Plot Names\nUI: Update Waveform Graph Labels\nUI: Update Displays" ("State(s) in Front (\"\")"), "State(s) in (\"\")"=w1238) -> ("States Out"=w1237:string)  [unwired: 13 in]
      }
      frame "Macro: Initialize DAQ SMO" {
        n602 = Unbundle By Name(w1240) -> ("Lockin.DAQ"=w1243:refnum<class "Instrument.DAQ.lvclass">)
        n603 = while {
          tunnel: [w1258] -> w1241
          tunnel: w1243 -> [w1257]
          tunnel: w1242 -> [w1256]
          tunnel: [w1254] -> w1239
          i -> [w1251]
          stop <- w1248 stop-if-true
          n604 = call <vilib>:"GetState.vi"("error in (no error)"=w1256, "SMO"=w1257) -> ("error out"=w1255:errorcluster, "SMO State"=w1253:T16)  [unwired: 7 in, 1 out]
          n605 = case shown="\"Started\"" w1253 {
            tunnel: ["" "Lockin SMO: Set AI Config\nLockin SMO: Set AO Config\nLockin SMO: Set AI\nLockin SMO: Set AO\nLockin SMO: Set REF\nLockin SMO: Set Input Gain\nLockin SMO: Set Output Gain\nMacro: Update Sampling\n//Lockin SMO: Set Sampling"] -> w1258
            tunnel: w1255 -> [w1260 w1263]
            tunnel: [w1259 w1263] -> w1254
            frame Default {
              n606 = call <userlib>:"Wait (ms)__ogtk.vi"("error in (no error)"=w1260, "milliseconds to wait"=u32 100) -> ("error out"=w1259:errorcluster)  [unwired: 8 in, 1 out]
            }
            frame "Started" {
              # "send all stuff to the Lockin.DAQ"
            }
          }
          n607 = Equal?(x=w1253, y=SMOState_--Enum."Started") -> (x = y?=w1249:bool)
          n608 = Greater?(x=w1251, y=10) -> (0:w1247:bool)
          n609 = Or(x=w1249, y=w1247) -> (x .or. y?=w1248:bool)
        }
        n610 = call <vilib>:"Add State(s) to Queue__jki_lib_state_machine.vi"("State(s) in Front (\"\")"=w1241, "State(s) in (\"\")"=w1246) -> ("States Out"=w1245:string)  [unwired: 13 in]
      }
      frame "Macro: Update Sampling" {
        w1279 = T50 10123 items=["Finite Samples"=10178, "Continuous Samples"=10123] ("Sample Mode")
        w1278 = T50 10178 items=["Finite Samples"=10178, "Continuous Samples"=10123] ("Sample Mode")
        # "#todo\nthis \"macro\" needs to\nbe handled by Lockin.DAQ\nor Handle Command"
        n611 = Unbundle By Name(w1269) -> ("Lockin"=w1266:refnum<class "Instrument.Lockin.lvclass">)
        n612 = Unbundle By Name(w1266) -> ("DAQ state"=w1265:T32)
        n613 = local read "Start"() -> (w1267:bool)
        n614 = case shown="\"created\", Default" w1265 {
          tunnel: ["" ("State with Arguments") w1291] -> w1273
          frame "idle" {
          }
          frame "created", Default {
            n615 = Format Into String(Set_State-enum."start" ("State")) -> (resulting string=w1292:string)  [unwired: 3 in, 1 out]
            n616 = call <vilib>:"Build State String with Arguments__JKI_lib_State_Machine.vi"("Arguments (\"\")"=w1292, "State"="Lockin SMO: Set State" ("f")) -> ("State with Arguments"=w1291:string)  [unwired: 4 in]
          }
        }
        n617 = case shown="\"created\", Default" w1265 {
          tunnel: ["" ("State with Arguments") w1286] -> w1275
          frame "idle" {
          }
          frame "created", Default {
            n618 = Format Into String(Set_State-enum."stop" ("State")) -> (resulting string=w1289:string)  [unwired: 3 in, 1 out]
            n619 = call <vilib>:"Build State String with Arguments__JKI_lib_State_Machine.vi"("Arguments (\"\")"=w1289, "State"="Lockin SMO: Set State" ("f")) -> ("State with Arguments"=w1286:string)  [unwired: 4 in]
          }
        }
        n620 = Select(t=w1279, s=w1267, f=w1278) -> (s? t:f=w1277:T50)
        n621 = Format Into String(w1277) -> (resulting string=w1276:string)  [unwired: 3 in, 1 out]
        n622 = call <vilib>:"Build State String with Arguments__JKI_lib_State_Machine.vi"("Arguments (\"\")"=w1276, "State"="Lockin SMO: Set Sampling") -> ("State with Arguments"=w1274:string)  [unwired: 4 in]
        n623 = call <vilib>:"Add State(s) to Queue__jki_lib_state_machine.vi"("State(s) in Front (\"\")"=w1275, "State(s) in (\"\")"=w1274, "State(s) at Back (\"\")"=w1273) -> ("States Out"=w1268:string)  [unwired: 12 in]
        n624 = call <vilib>:"Add State(s) to Queue__jki_lib_state_machine.vi"("State(s) in Front (\"\")"="4461: SAMPLING SETUP" ("State(s) in Front (\"\")"), "State(s) in (\"\")"="" ("State(s) in Front (\"\")"), "State(s) at Back (\"\")"=w1268) -> ("States Out"=w1270:string)  [unwired: 12 in]
        n625 = call <vilib>:"Add State(s) to Queue__jki_lib_state_machine.vi"("State(s) in Front (\"\")"=w1270, "State(s) in (\"\")"=w1284) -> ("States Out"=w1283:string)  [unwired: 13 in]
      }
      frame "Macro: Exit" {
        # "Exit Macro\n(This is called once, when the VI exits)"
        n626 = Unbundle By Name(w1299) -> ("Core.Close Panel on Exit?"=w1303:bool)
        n627 = Select(t="UI: Front Panel State >> Close", s=w1303, f="") -> (s? t:f=w1302:string)
        n628 = call <vilib>:"Add State(s) to Queue__jki_lib_state_machine.vi"("State(s) in Front (\"\")"="Lockin SMO: Set AO Zero Amplitude\nUI: Disable Buttons\nUI: Cleanup", "State(s) in (\"\")"=w1302, "State(s) at Back (\"\")"="Data: Cleanup\nExit") -> ("States Out"=w1300:string)  [unwired: 12 in]
        n629 = call <vilib>:"Add State(s) to Queue__jki_lib_state_machine.vi"("State(s) in Front (\"\")"=w1300, "State(s) in (\"\")"=w1306) -> ("States Out"=w1305:string)  [unwired: 13 in]
      }
      frame "---------- Lockin SMO ----------" {
        n630 = call <vilib>:"Add State(s) to Queue__jki_lib_state_machine.vi"("State(s) in (\"\")"=w1311) -> ("States Out"=w1310:string)  [unwired: 14 in]
      }
      frame "Lockin SMO: Set State" {
        # "#lockin:process"
        n631 = Unbundle By Name(w1312) -> ("Lockin.DAQ"=w1318:refnum<class "Instrument.DAQ.lvclass">)
        n632 = case shown="\"start\"" w1314 {
          tunnel: [Set_State-enum."stop" ("State") Set_State-enum."start" ("State") Set_State-enum."reset" ("State") Set_State-enum."start sweep" ("State") Set_State-enum."stop sweep" ("State")] -> w1313
          tunnel: [FALSE ("Trigger") TRUE ("Trigger") w1326 TRUE ("Trigger") TRUE ("Trigger")] -> w1315
          frame "stop", Default {
          }
          frame "start" {
          }
          frame "reset" {
            n633 = local read "Start"() -> (w1326:bool)
          }
          frame "start sweep" {
          }
          frame "stop sweep" {
          }
        }
        n634 = local write "Start"(w1315) -> ()
        n635 = call "DAQ.setstate.vi"("error in (no error)"=w1317, "setState"=w1313, "Instrument.DAQ"=w1318) -> ("error out"=w1316:errorcluster)  [unwired: 7 in, 1 out]
        n636 = call <vilib>:"Add State(s) to Queue__jki_lib_state_machine.vi"("State(s) in (\"\")"=w1321) -> ("States Out"=w1320:string)  [unwired: 14 in]
      }
      frame "Lockin SMO: Set AI Config" {
        # "#lockin:process"
        n637 = Unbundle By Name(w1333) -> ("Lockin.DAQ"=w1338:refnum<class "Instrument.DAQ.lvclass">, "Lockin"=w1334:refnum<class "Instrument.Lockin.lvclass">)
        n638 = Unbundle By Name(w1334) -> ("AI"=w1335:T46)
        n639 = call "DAQ.setAIconfig.vi"("error in (no error)"=w1337, "Simulation mode"="AI Simulation mode", "AI Configuration"=w1335, "Instrument.DAQ"=w1338) -> ("error out"=w1336:errorcluster)  [unwired: 6 in, 1 out]
        n640 = call <vilib>:"Add State(s) to Queue__jki_lib_state_machine.vi"("State(s) in (\"\")"=w1341) -> ("States Out"=w1340:string)  [unwired: 14 in]
      }
      frame "Lockin SMO: Set AO Config" {
        # "#lockin:process"
        n641 = Unbundle By Name(w1343) -> ("Lockin.DAQ"=w1347:refnum<class "Instrument.DAQ.lvclass">, "Lockin"=w1344:refnum<class "Instrument.Lockin.lvclass">)
        n642 = Unbundle By Name(w1344) -> ("AO"=w1342:T44)
        n643 = call "DAQ.setAOconfig.vi"("error in (no error)"=w1346, "AO Configuration"=w1342, "Instrument.DAQ"=w1347) -> ("error out"=w1345:errorcluster)  [unwired: 7 in, 1 out]
        n644 = call <vilib>:"Add State(s) to Queue__jki_lib_state_machine.vi"("State(s) in (\"\")"=w1350) -> ("States Out"=w1349:string)  [unwired: 14 in]
      }
      frame "Lockin SMO: Set Sampling" {
        # "#lockin:process"
        # "Is there a more elegant way to do this?"
        n645 = Unbundle By Name(w1352) -> ("Lockin.DAQ"=w1359:refnum<class "Instrument.DAQ.lvclass">, "Lockin"=w1355:refnum<class "Instrument.Lockin.lvclass">)
        n646 = Unbundle By Name(w1355) -> ("Sampling"=w1353:T59)
        n647 = case shown="\"10178\", Default" w1354 {
          tunnel: [w1363 w1364] -> w1356
          frame "10178", Default {
            w1363 = T50 10178 items=["Finite Samples"=10178, "Continuous Samples"=10123] ("Sample Mode")
          }
          frame "10123" {
            w1364 = T50 10123 items=["Finite Samples"=10178, "Continuous Samples"=10123] ("Sample Mode")
          }
        }
        n648 = call "DAQ.setSampling.vi"(6:"decimating factor", "error in (no error)"=w1358, 9:w1356, "Sampling"=w1353, "Instrument.DAQ"=w1359) -> ("error out"=w1357:errorcluster)  [unwired: 5 in, 1 out]
        n649 = call <vilib>:"Add State(s) to Queue__jki_lib_state_machine.vi"("State(s) in (\"\")"=w1362) -> ("States Out"=w1361:string)  [unwired: 14 in]
      }
      frame "Lockin SMO: Set AO" {
        # "#lockin:process"
        n650 = Unbundle By Name(w1365) -> ("Lockin.DAQ"=w1370:refnum<class "Instrument.DAQ.lvclass">, "Lockin"=w1367:refnum<class "Instrument.Lockin.lvclass">)
        n651 = Unbundle By Name(w1367) -> ("AO"=w1366:T61)
        n652 = call "DAQ.setAO.vi"("error in (no error)"=w1369, "AO Channels"=w1366, "Instrument.DAQ"=w1370) -> ("error out"=w1368:errorcluster)  [unwired: 7 in, 1 out]
        n653 = call <vilib>:"Add State(s) to Queue__jki_lib_state_machine.vi"("State(s) in (\"\")"=w1373) -> ("States Out"=w1372:string)  [unwired: 14 in]
      }
      frame "Lockin SMO: Set AO Zero Amplitude" {
        # "#lockin:process"
        n654 = Unbundle By Name(w1380) -> ("Lockin.DAQ"=w1387:refnum<class "Instrument.DAQ.lvclass">, "Lockin"=w1379:refnum<class "Instrument.Lockin.lvclass">)
        n655 = Unbundle By Name(w1379) -> ("AO"=w1374:T61, "#s"=w1385:i32, "Fs"=w1384:dbl)
        n656 = Divide(x=w1385, y=w1384) -> (x/y=w1377:dbl)
        n657 = Multiply(x=1000.0 ("y"), y=w1377) -> (x*y=w1383:dbl)
        n658 = for {
          tunnel: w1374 -> [w1393] mode=indexing
          tunnel: [w1391] -> w1376 mode=indexing
          n659 = Bundle By Name(cluster=w1393, "Amplitude"=0.0 ("element")) -> (w1391:T62)
        }
        n660 = To Unsigned Long Integer(number=w1383) -> (unsigned 32bit integer=w1382:u32)
        n661 = call "DAQ.setAO.vi"("error in (no error)"=w1386, "AO Channels"=w1376, "Instrument.DAQ"=w1387) -> ("error out"=w1375:errorcluster)  [unwired: 7 in, 1 out]
        n662 = call <userlib>:"Wait (ms)__ogtk.vi"("error in (no error)"=w1375, "milliseconds to wait"=w1382) -> ("error out"=w1381:errorcluster)  [unwired: 8 in, 1 out]
        n663 = call <vilib>:"Add State(s) to Queue__jki_lib_state_machine.vi"("State(s) in (\"\")"=w1390) -> ("States Out"=w1389:string)  [unwired: 14 in]
      }
      frame "Lockin SMO: Set REF" {
        # "#lockin:process"
        n664 = Unbundle By Name(w1396) -> ("Lockin.DAQ"=w1399:refnum<class "Instrument.DAQ.lvclass">, "Lockin"=w1397:refnum<class "Instrument.Lockin.lvclass">)
        n665 = Unbundle By Name(w1397) -> ("REF"=w1394:T38)
        n666 = call "DAQ.setREF.vi"("error in (no error)"=w1395, "Channels: Lockin"=w1394, "Instrument.DAQ"=w1399) -> ("error out"=w1398:errorcluster)  [unwired: 7 in, 1 out]
        n667 = call <vilib>:"Add State(s) to Queue__jki_lib_state_machine.vi"("State(s) in (\"\")"=w1402) -> ("States Out"=w1401:string)  [unwired: 14 in]
      }
      frame "Lockin SMO: Set AI" {
        # "#lockin:process"
        n668 = Unbundle By Name(w1407) -> ("Lockin.DAQ"=w1406:refnum<class "Instrument.DAQ.lvclass">, "Lockin"=w1408:refnum<class "Instrument.Lockin.lvclass">)
        n669 = Unbundle By Name(w1408) -> ("AI"=w1403:T57)
        n670 = call "DAQ.setAI.vi"("error in (no error)"=w1405, "AI Channels"=w1403, "Instrument.DAQ"=w1406) -> ("error out"=w1404:errorcluster)  [unwired: 7 in, 1 out]
        n671 = call <vilib>:"Add State(s) to Queue__jki_lib_state_machine.vi"("State(s) in (\"\")"=w1411) -> ("States Out"=w1410:string)  [unwired: 14 in]
      }
      frame "Lockin SMO: Set Input Gain" {
        # "#lockin:process"
        n672 = Unbundle By Name(w1412) -> ("Lockin.DAQ"=w1417:refnum<class "Instrument.DAQ.lvclass">, "Lockin"=w1415:refnum<class "Instrument.Lockin.lvclass">)
        n673 = Unbundle By Name(w1415) -> ("AI.Gain"=w1414:T48)
        n674 = call "DAQ.setInputGain.vi"("error in (no error)"=w1413, "Input Gain"=w1414, "Instrument.DAQ"=w1417) -> ("error out"=w1416:errorcluster)  [unwired: 7 in, 1 out]
        n675 = call <vilib>:"Add State(s) to Queue__jki_lib_state_machine.vi"("State(s) in (\"\")"=w1420) -> ("States Out"=w1419:string)  [unwired: 14 in]
      }
      frame "Lockin SMO: Set Output Gain" {
        # "#lockin:process"
        n676 = Unbundle By Name(w1425) -> ("Lockin.DAQ"=w1424:refnum<class "Instrument.DAQ.lvclass">, "Lockin"=w1426:refnum<class "Instrument.Lockin.lvclass">)
        n677 = Unbundle By Name(w1426) -> ("AO.Gain"=w1422:T48)
        n678 = call "DAQ.setOutputGain.vi"("error in (no error)"=w1423, "Output Gain"=w1422, "Instrument.DAQ"=w1424) -> ("error out"=w1421:errorcluster)  [unwired: 7 in, 1 out]
        n679 = call <vilib>:"Add State(s) to Queue__jki_lib_state_machine.vi"("State(s) in (\"\")"=w1429) -> ("States Out"=w1428:string)  [unwired: 14 in]
      }
      frame "Lockin SMO: Set Prefilter" {
        # "#lockin:process"
        n680 = Unbundle By Name(w1432) -> ("Lockin.DAQ"=w1434:refnum<class "Instrument.DAQ.lvclass">, "Lockin"=w1435:refnum<class "Instrument.Lockin.lvclass">)
        n681 = Unbundle By Name(w1435) -> ("Prefilter"=w1433:T63)
        n682 = call "DAQ.setPreFilter.vi"("error in (no error)"=w1431, "PreFilter"=w1433, "Instrument.DAQ"=w1434) -> ("error out"=w1430:errorcluster)  [unwired: 7 in, 1 out]
        n683 = call <vilib>:"Add State(s) to Queue__jki_lib_state_machine.vi"("State(s) in (\"\")"=w1438) -> ("States Out"=w1437:string)  [unwired: 14 in]
      }
      frame "Lockin SMO: Calibration" {
        # "?????????????????"
        # "#lockin:process"
        # "This will only get the current calibration inf\nActually doing calibration is done via Set State >> Calibration"
        n684 = Unbundle By Name(w1444) -> ("Lockin.DAQ"=w1443:refnum<class "Instrument.DAQ.lvclass">)
        n685 = case shown="\"True\"" w1439 {
          tunnel: [PrivateEvents--DAQ.setCalibration."Check" ("setCalibration") PrivateEvents--DAQ.setCalibration."Check" ("setCalibration")] -> w1440
          frame "False", Default {
            # "check calibration"
          }
          frame "True" {
            # "calibrate"
          }
        }
        n686 = call "DAQ.setCalibration.vi"("error in (no error)"=w1442, "setCalibration"=w1440, "Instrument.DAQ"=w1443) -> ("error out"=w1441:errorcluster)  [unwired: 7 in, 1 out]
        n687 = call <vilib>:"Add State(s) to Queue__jki_lib_state_machine.vi"("State(s) in (\"\")"=w1447) -> ("States Out"=w1446:string)  [unwired: 14 in]
      }
      frame "Lockin SMO: Auto DAQ" {
        # "#lockin:process"
        n688 = Unbundle By Name(w1453) -> ("Lockin.DAQ"=w1452:refnum<class "Instrument.DAQ.lvclass">)
        n689 = call "DAQ.autoConfigureDAQ.vi"("error in (no error)"=w1451, "Instrument.DAQ"=w1452) -> ("error out"=w1450:errorcluster)  [unwired: 8 in, 1 out]
        n690 = call <vilib>:"Add State(s) to Queue__jki_lib_state_machine.vi"("State(s) in (\"\")"=w1456) -> ("States Out"=w1455:string)  [unwired: 14 in]
      }
      frame "Lockin SMO: Reset Phase" {
        # "#lockin:process"
        n691 = Unbundle By Name(w1460) -> ("Lockin.DAQ"=w1459:refnum<class "Instrument.DAQ.lvclass">)
        n692 = call "DAQ.zeroPhase.vi"("error in (no error)"=w1458, "Instrument.DAQ"=w1459) -> ("error out"=w1457:errorcluster)  [unwired: 8 in, 1 out]
        n693 = call <vilib>:"Add State(s) to Queue__jki_lib_state_machine.vi"("State(s) in (\"\")"=w1463) -> ("States Out"=w1462:string)  [unwired: 14 in]
      }
      frame "Lockin SMO: Measure Offset" {
        # "#lockin:process"
        n694 = Unbundle By Name(w1464) -> ("Lockin.DAQ"=w1467:refnum<class "Instrument.DAQ.lvclass">)
        n695 = call "DAQ.measureOffset.vi"("error in (no error)"=w1466, "Instrument.DAQ"=w1467) -> ("error out"=w1465:errorcluster)  [unwired: 8 in, 1 out]
        n696 = call <vilib>:"Add State(s) to Queue__jki_lib_state_machine.vi"("State(s) in (\"\")"=w1470) -> ("States Out"=w1469:string)  [unwired: 14 in]
      }
      frame "Lockin SMO: Remove Offset" {
        # "#lockin:process"
        n697 = Unbundle By Name(w1472) -> ("Lockin.DAQ"=w1474:refnum<class "Instrument.DAQ.lvclass">)
        n698 = call "DAQ.zeroOffset.vi"("error in (no error)"=w1473, "Instrument.DAQ"=w1474) -> ("error out"=w1471:errorcluster)  [unwired: 8 in, 1 out]
        n699 = call <vilib>:"Add State(s) to Queue__jki_lib_state_machine.vi"("State(s) in (\"\")"=w1477) -> ("States Out"=w1476:string)  [unwired: 14 in]
      }
      frame "---------- 4461----------" {
        n700 = call <vilib>:"Add State(s) to Queue__jki_lib_state_machine.vi"("State(s) in (\"\")"=w1482) -> ("States Out"=w1481:string)  [unwired: 14 in]
      }
      frame "4461: SAMPLING SETUP" {
        # "#todo\n*I think* this \"macro\" needs to\nbe handled by Lockin.DAQ\nor Handle Command"
        # "#macro sorta"
        # "#todo\nshould this be in Lockin.DAQ SMO? or in Handle Command?"
        # "Max Fs"
        n701 = Unbundle By Name(w1488) -> ("Lockin"=w1486:refnum<class "Instrument.Lockin.lvclass">)
        n702 = case shown="Default" "DAQ Type" {
          tunnel: [102400.0 ("upper limit") 204800.0 ("upper limit")] -> w1490
          frame "USB 4431" {
          }
          frame Default {
          }
        }
        n703 = case shown="\"Auto Fs\"" "Sampling Mode" {
          tunnel: [w1499 w1500 w1514] -> w1491
          tunnel: w1486 -> [_ w1502 _]
          tunnel: w1490 -> [_ w1505 w1515]
          tunnel: "Max Fs Refresh Rate (Hz)" -> [_ _ w1510]
          frame "Manual", Default {
            n704 = local read "Sampling"() -> (w1499:T11)
          }
          frame "Auto Fs" {
            # "#todo: owned by Lockin or LockinDAQ?"
            # "#todo: make subVI?"
            # "max Fs"
            n705 = Unbundle By Name(w1502) -> ("AO"=w1506:T61)
            n706 = Index Array(array=w1506) -> (element=w1503:T62)  [unwired: 1 in]
            n707 = Unbundle By Name(w1503) -> ("Frequency"=w1501:dbl)
            n708 = Multiply(x="Auto x*F1", y=w1501) -> (x*y=w1504:dbl)
            n709 = In Range and Coerce(upper limit=w1505, x=w1504, lower limit=1000.0) -> (coerced(x)=w1509:dbl)  [unwired: 1 out]
            n710 = call "DAQ.Sampling.Find Integer Period Fs and Ns.vi"("f integer"=w1501, "Max Fs"=w1509) -> ("Timing out"=w1500:T11)  [unwired: 9 in]
          }
          frame "Max Fs" {
            n711 = Divide(x=w1515, y=w1510) -> (x/y=w1513:dbl)
            n712 = To Long Integer(number=w1513) -> (32bit integer=w1512:i32)
            n713 = Bundle By Name(cluster=T11 {"Fs"=204789.0, "#s"=15753} ("Sampling"), "Fs"=w1515, "#s"=w1512) -> (w1514:T11)
          }
        }
        n714 = call "DAQ.Sampling.Coerce Timing.vi"("Max Fs"=w1490, "Sampling in"=w1491) -> ("Sampling out"=w1484:T11)  [unwired: 9 in]
        n715 = Bundle By Name(cluster=w1486, "Sampling"=w1484) -> (w1485:refnum<class "Instrument.Lockin.lvclass">)
        n716 = Bundle By Name(cluster=w1488, "Lockin"=w1485) -> (w1487:T36)
        n717 = local write "Sampling"(w1484) -> ()
        n718 = call <vilib>:"Add State(s) to Queue__jki_lib_state_machine.vi"("State(s) in (\"\")"=w1496) -> ("States Out"=w1495:string)  [unwired: 14 in]
      }
      frame "4461: OUT" {
        # "#todo\nmove to Lockin.DAQ?"
        n719 = Unbundle By Name(w1517) -> ("Lockin"=w1520:refnum<class "Instrument.Lockin.lvclass">)
        n720 = case shown="True" "Enable Output" {
          tunnel: [w1524 w1533] -> w1518
          tunnel: w1520 -> [_ w1536]
          tunnel: w1516 -> [w1524 w1531]
          frame False {
          }
          frame True {
            # "this will act as a self-call\nmeaning after the remote call comes\nin the data on the data bus will get updated\nby other means"
            n721 = Unbundle By Name(w1536) -> ("Results (Dictionary)"=w1532:cluster{"key":string, "value":dbl}[], "AI.Gain"=w1526:T48)
            n722 = call "Parse Results (single).vi"("Type"="Type", "error in (no error)"=w1531, "Reference Channel"="Reference Channel", "AI Channel"="AI Channel", "Results (Dictionary)"=w1532) -> ("error out"=w1530:errorcluster, "Data"=w1534:dbl)  [unwired: 3 in, 2 out]
            n723 = Decrement(x="AI Channel") -> (x-1=w1525:i32)
            n724 = Index Array(array=w1526, index=w1525) -> (element=w1535:T49)
            n725 = Multiply(x=w1534, y=w1535) -> (x*y=w1537:dbl)
            "Output (V)" <- w1537
            n726 = call "setAO_DC.vi"("error in (no error)"=w1530, "DC (V)"=w1537, "AO Channel"="Output Channel", "Instrument.Lockin in"=w1536) -> ("error out"=w1533:errorcluster)  [unwired: 6 in, 1 out]
          }
        }
        n727 = call <vilib>:"Add State(s) to Queue__jki_lib_state_machine.vi"("State(s) in (\"\")"=w1522) -> ("States Out"=w1523:string)  [unwired: 14 in]
      }
      frame "4461: FFT" {
        n728 = Unbundle By Name(w1557) -> ("Lockin"=w1556:refnum<class "Instrument.Lockin.lvclass">)
        n729 = Unbundle By Name(w1556) -> ("AI"=w1546:waveform(dbl)[])
        n730 = Bundle By Name(cluster=T30 {"averaging mode"=enum."No averaging", "weighting mode"=enum."Exponential", "number of averages"=10} ("averaging parameters"), "averaging mode"="averaging mode", "weighting mode"="weighting mode", "number of averages"="# averages") -> (w1549:T30)
        n731 = call-poly <vilib>:"FFT Power Spectrum and PSD.vi"("export mode"="export mode", "averaging parameters"=w1549, "restart averaging (F)"="restart", "error in (no error)"=w1545, "dB On (F)"=TRUE, "window"="window", "time signals"=w1546) -> ("error out"=w1558:errorcluster, "averages completed"=→"averages":dbl, "averaging done"=→"done?":bool, "Power Spectrum / PSD"=w1542:cluster{"f0":dbl, "df":dbl, "magnitude":dbl[]}[])  [unwired: 1 in]
        "PS WFGraph" <- w1542
        n732 = control-ref of="PS WFGraph"() -> (w1539:refnum<vi>)
        n733 = for {
          tunnel: [w1565] -> w1544
          tunnel: w1545 -> [w1564]
          tunnel: w1542 -> [_] mode=indexing
          i -> [w1567]
          n734 = property on="PS WFGraph" class="WFGraph (strict)"(error in=w1564, "Active Plot"=w1567) -> (error out=w1568:errorcluster, "Plot.Visible?"=w1566:bool)  [unwired: 1 in, 1 out]
          n735 = property on="PS Chart" class="WFChart (strict)"(error in=w1568, "Active Plot"=w1567, "Plot.Visible?"=w1566) -> (error out=w1565:errorcluster)  [unwired: 1 in, 1 out]
        }
        n736 = call "PS Chart.vi"("error in (no error)"=w1558, "Power Spectrum / PSD"=w1542, "WFGraph (WDT) in"=w1539) -> ("error out"=w1541:errorcluster, "Chart"=→"PS Chart":dbl[][])  [unwired: 7 in]
        n737 = Merge Errors(w1541, w1544) -> (w1540:errorcluster)
        n738 = call <vilib>:"Add State(s) to Queue__jki_lib_state_machine.vi"("State(s) in (\"\")"=w1559) -> ("States Out"=w1563:string)  [unwired: 14 in]
      }
      frame "---------- AUX ----------" {
        n739 = call <vilib>:"Add State(s) to Queue__jki_lib_state_machine.vi"("State(s) in (\"\")"=w1573) -> ("States Out"=w1572:string)  [unwired: 14 in]
      }
      frame "AUX: Set AUX" {
        # "#todo\nmove to Lockin.DAQ?"
        n740 = call <userlib>:"Voltage Update.vi"("error in (no error)"=w1576, "Amplifier Gain"="Amplifier Gain", "Voltage Output"="Voltage Output (V)", "Physical Channel"="Aux Channel") -> ("error out"=w1575:errorcluster, "Amplified output"=→"Amplified Output (V)":dbl, "DAQ output"=→"DAQ Output (V)":dbl)  [unwired: 5 in]
        n741 = Unbundle By Name(w1578) -> ("Lockin"=w1574:refnum<class "Instrument.Lockin.lvclass">)
        n742 = Bundle By Name(cluster=w1578, "Lockin"=w1574) -> (w1580:T36)
        n743 = call <vilib>:"Add State(s) to Queue__jki_lib_state_machine.vi"("State(s) in Front (\"\")"="" ("State(s) in Front (\"\")"), "State(s) in (\"\")"=w1587) -> ("States Out"=w1586:string)  [unwired: 13 in]
      }
      frame "---------Command----------" {
        n744 = call <vilib>:"Add State(s) to Queue__jki_lib_state_machine.vi"("State(s) in (\"\")"=w1592) -> ("States Out"=w1591:string)  [unwired: 14 in]
      }
      frame "Command: setOffset" {
        # "Convert Data from Message\nto appropriate data type"
        # "Triggers User Event to update front panel\nand put data onto class wire"
        n745 = Unbundle By Name(w1602) -> ("Message"=w1601:T34, "Message.Data"=w1597:variant)  [unwired: 1 out]
        n746 = Variant To Data(error in=w1596, type="" ("String"), Variant=w1597) -> (data=w1598:string, error out=w1600:errorcluster)
        n747 = call "From JSON Text.vim"("Data Type and Default Value"=Offset_Mode--Enum."Remove" ("Offset Mode"), "error in (no error)"=w1600, "JSON"=w1598) -> ("error out"=w1594:errorcluster, "Data out"=w1593:T31)  [unwired: 7 in]
        n748 = case shown="\"Remove\"" w1593 {
          tunnel: ["Lockin SMO: Measure Offset" ("State(s) in Front (\"\")") "Lockin SMO: Remove Offset" ("State(s) in Front (\"\")")] -> w1604
          frame "Measure", Default {
          }
          frame "Remove" {
          }
        }
        n749 = Bundle By Name(cluster=w1601, "Data"=w1593) -> (w1605:T34)
        n750 = Bundle By Name(cluster=w1602, "HandledMessage"=w1605) -> (w1603:T36)
        n751 = call <vilib>:"Add State(s) to Queue__jki_lib_state_machine.vi"("State(s) in Front (\"\")"=w1604, "State(s) in (\"\")"=w1608) -> ("States Out"=w1607:string)  [unwired: 13 in]
      }
      frame "---------- Notes ----------" {
        n752 = call <vilib>:"Add State(s) to Queue__jki_lib_state_machine.vi"("State(s) in (\"\")"=w1615) -> ("States Out"=w1614:string)  [unwired: 14 in]
      }
      frame "Notes: Controls" {
        n753 = call <vilib>:"Add State(s) to Queue__jki_lib_state_machine.vi"("State(s) in (\"\")"=w1620) -> ("States Out"=w1619:string)  [unwired: 14 in]
      }
      frame "Notes: Notes" {
        # "calculate RMS, Noise bandwidth, etc"
        # "Go to \"4461: SETUP\" if Reset, remote mode,\nor IV/continuous mode buttons are pushed"
        # "Multichannel Lockin v2016/06/02 SW TIMED SINGLE POINT\nREF:\nhttp://www.ni.com/white-paper/3215/en/ Example 9"
        # "TO DO:\n- intelligent decimate to dt setpoint\ncalculate RMS, Noise bandwidth, etc"
        n754 = disable-structure shown="Enabled" {
          frame Disabled {
            n755 = call <vilib>:"Open Config Data.vi"() -> ()  [unwired: 9 in, 3 out]
          }
          frame Enabled {
            # "JKI State Machine™\nhttp://jkisoft.com/state-machine/\nCopyright (C) 2005-2008, JKI <info@jkisoft.com>\nALL RIGHTS RESERVED"
            # "State Syntax:\nStateCategory: State >> Argument\nLine Terminator: Line feed\nExample:\nUI: Help >> About\n\nWhere \"UI\" is the state category\nWhere \"Help\" is the state\nWhere \"About\" is the argument\nOther Examples:\nApp Data: Initialize\nUI: Initialize\nHelp >> About\n\nCommenting:\nTo add a comment use \"//\" or \"#\" and all text to the right will be ignored\n\nCommenting Example:\nUI: Initialize // This initializes the UI\n# This whole line is a comment\n// Another comment line"
          }
        }
        n756 = call <vilib>:"Add State(s) to Queue__jki_lib_state_machine.vi"("State(s) in (\"\")"=w1625) -> ("States Out"=w1624:string)  [unwired: 14 in]
      }
    }
    n757 = call <userlib>:"State History.vi"("Current State"=w7) -> ("History"=→"State History":string)  [unwired: 6 in]
  }
